vi "BRig_RT_start_v1,19.vi"() -> ()   [LabVIEW 2014]
uses:
  myRIO_BRig_RT__Case_Exp_stateList.ctl
  myRIO_BRig_RT__Case_NonExp_stateList.ctl
  <vilib>/WebDAVClient/Advanced/SessionHandle.ctl
  <vilib>/Platform/TimedLoop/XDataNode/timing_clust.ctl
  <vilib>/Platform/TimedLoop/XDataNode/nitl_modes.ctl
  <vilib>/Platform/TimedLoop/XDataNode/wakeup.ctl
  <vilib>/myRIO/Common/Instrument Driver Framework/myRIO v1.0/UART/vis/myRIO v1.0 Close UART.vi
  <vilib>/FPGAPlugInAG/myRIO-1900/niLvFpga_Open_myRIO-1900.vi
  <vilib>/rvi/interface/common/dynamic/niFpgaDynamicAddResources.vi
  <vilib>/Utility/error.llb/Error Cluster From Error Code.vi
  <vilib>/rvi/errors/niLvFpgaAdjustHostInterfaceError.vi
  <vilib>/Utility/file.llb/Read From Spreadsheet File (I64).vi
  <vilib>/Utility/file.llb/Write To Spreadsheet File (DBL).vi
  <vilib>/FPGAPlugInAG/Dynamic/niLvFpga_Close_Dynamic.vi
  <vilib>/myRIO/Common/Instrument Driver Framework/Utilities/vis/FPGA Ref Manager.vi
  <vilib>/myRIO/Common/Instrument Driver Framework/myRIO v1.0/myRIO v1.0 Reset FPGA.vi
  <vilib>/myRIO/Common/Instrument Driver Framework/myRIO v1.0/IRQ/vis/myRIO v1.0 IRQ Info FGV.vi
  <vilib>/myRIO/Common/Instrument Driver Framework/myRIO v1.0/IRQ/vis/myRIO v1.0 Timer IRQ Info FGV.vi
  <vilib>/myRIO/Common/Instrument Driver Framework/myRIO v1.0/IRQ/vis/myRIO v1.0 ISR Agent.vi
  <vilib>/rvi/interface/nirviOpenFPGA/nirviOpenFPGA.xnode
  BRig_FPGA_v3,95__build.lvbitx
  BRig_FPGA_v3,95.vi
  <vilib>/rvi/interface/nirviReadWriteControl/nirviReadWriteControl.xnode
  <vilib>/Platform/TimedLoop/XDataNode/XDataNode.xnode
  <vilib>/rvi/interface/nirviCloseFPGA/nirviCloseFPGA.xnode
  <vilib>/Platform/TimedLoop/XDataNode/XDNodeRunTimeDep.lvlib
  <vilib>/rvi/interface/Simulation/niFpgaSimulationCallBeginRW.vi
  <vilib>/myRIO/Instrument Drivers/Utilities/Utilities.lvlib
  NiFpgaLv.dll
  <vilib>/WebDAVClient/NI_WebDAV.lvlib
panel:
  out "DAB_flipLR":bool caption="Flip?\n(DAB)"
  in  "LaserFiber_V_l2":dbl
  in  "LaserFiber_V_l1":dbl
  out "Solenoid R":bool
  out "Solenoid L":bool
  out "Laser2":bool
  out "Laser1":bool
  out "FreeReward_c_R":u16
  out "FreeReward_c_L":u16
  in  "Laser2_LED":bool
  in  "Laser1_LED":bool
  in  "lick_Rising(F)_or_Falling(T)":bool
  out "T_ExpRun_min":dbl
  out "stop_TimedLoop":bool
  out "BTPR_avg_R":dbl
  out "T2R_avg_R":dbl
  out "BTPR_avg_L":dbl
  out "T2R_avg_L":dbl
  out "BTPR_block":u16
  out "T2R_block":u16
  in  "comm_WebDAV_connect":bool
  in  "I_sendData":bool
  in  "comm_TCP_connect":bool
  out "nRewards_total":u16 caption="# Rewards in Current Block"
  out "BUR_target":u16 caption="Target Trials Per Block"
  in  "input_Threshold_reset":bool
  out "nTrial":u16
  out "allReward_R":bool
  out "allReward_L":bool
  out "Threshold":bool
  out "tLoop":dbl format="%#_2g"
  out "L_Power_l2":dbl
  out "comm_TCP":bool
  in  "get_countPerMS":bool
  out "SolenoidReward":bool
  out "L_Power_l1":dbl caption="LaserPower"
  in  "Recording":bool
  out "FPGA_count2ms":dbl=159.0
  out "error out":errorcluster
  out "cSpout":enum16{"Left", "Right"}(ring) caption="Left or Right Spout"
  out "A4":u32 caption="LickCounter_Right"
  out "A2":u32 caption="LickCounter_Left"
  out "nRewards_Right":u16 caption="# Rewards Total (Right)"
  out "nRewards_Left":u16 caption="# Rewards Total (Left)"
  out "nRewards_cur":u16 caption="# Rewards in Current Block"
  out "TpB_target":u16 caption="Target Trials Per Block"
  out "cState_NonExp":T1 caption="WarmUp State"
  out "iBlock":u16 caption="Current Block"
  out "cState":T2 caption="Experimental State"
  out "iTrial":u16 caption="Current Trial"
  in  "Data Set Prefix":string="Exp1_TM2"
  out "comm_WebDAV":bool
  in  "Host Password":string="sabalab"
  in  "Host UserName":string="Test2"
  in  "STOP_abort":bool caption="Stop LabView\n(Stops myRio and FPGA)"
  in  "STOP_endBlock":bool caption="Stop Experiment\n@ End of Block"
  in  "STOP_endTrial":bool caption="Stop Experiment\n@ End of Trial"
  in  "START":bool caption="Start Experiment"
  # "Experimental Run"
  # "Recording Rig"
  # "FPGA Conversion\n[counts per ms]"
  # "RealTime Cycle\nShould be <5ms"
  # "STOP experiment at"
  # "Exp Run Time"
  # "Reset"
  # "min"
  # "Communication with Host"
  # "Lick Counter"
  # "Block Target"
  # "Give Water?\n(Reward)"
  # "# Blocks"
  # "Experimental State"
  # "Left/Right"
  # "# Trials"
  # "# Rewards"
  # "Left           Right"
  # "Bad Trials\nPost Reward"
  # "Trials 2 Reward"
  # "Direction\n(NonSpecific Licking)"
  # "Block"
  # "Laser1"
  # "Laser2"
  # "# Trials"
  # "# Rewards"
  # "Current\nBlock"
  # "L          R"
  # "Power [V]"
  # "avg L"
  # "Toggle\nLED"
  # "Total"
  # "# Rewards"
  # "Laser Trigger"
  # "# Trials"
  # "avg R"
  # "1          2"
  # "Fiber Angle\n[V]"
  # "Left           Right"
  # "FreeRewards"
  # "Solenoid Trigger"
  # "WarmUp State"
  # "Lick Detection\nRising (F) or Falling (T)"
  # "L          R"
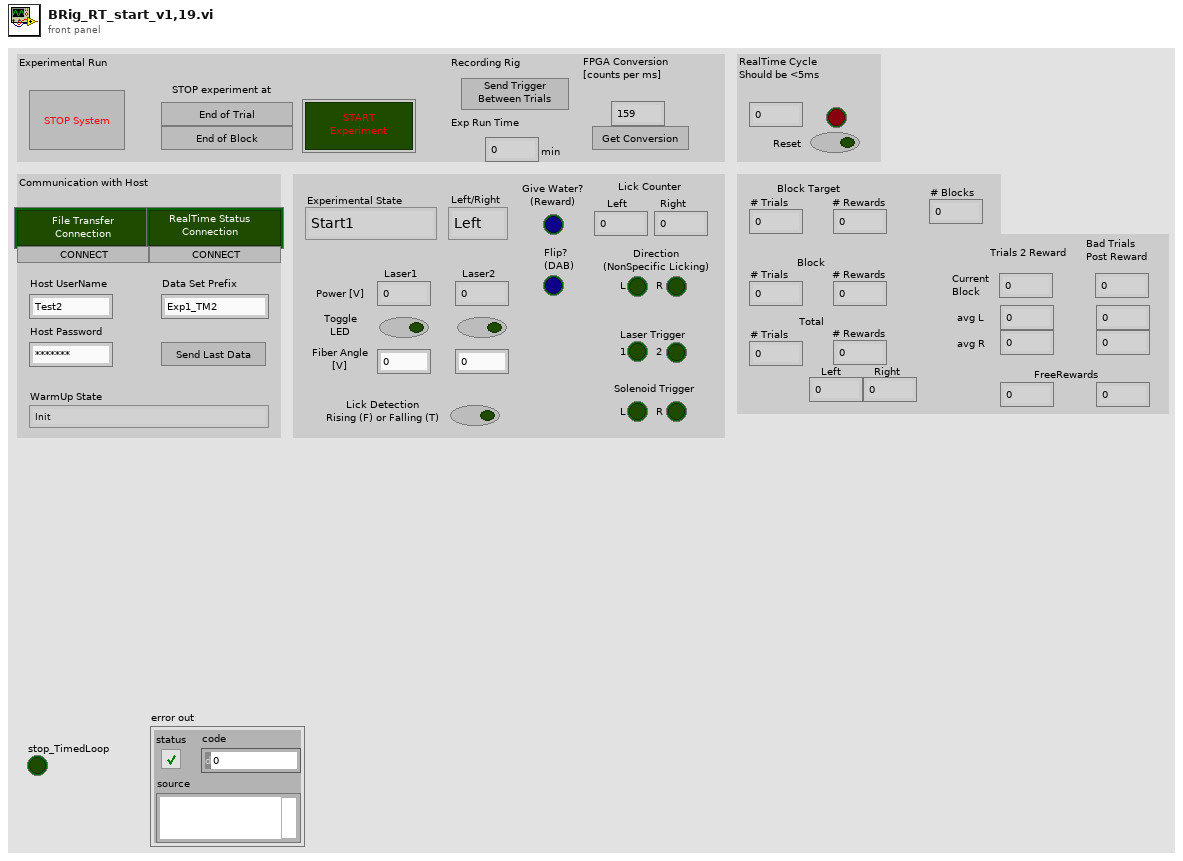
[diagram p1: front panel]
types:
  T1 = typedef "myRIO_BRig_RT__Case_NonExp_stateList.ctl" = enum16{"Init", "UploadSettings_pre", "UploadSettings_Read_dataExp", "UploadSettings_dataExp_1", "UploadSettings_dataExp_2", "UploadSettings_Read_dataLC", "UploadSettings_dataLC_1", "UploadSettings_dataLC_2", "UploadSettings_dataLC_3", "UploadSettings_dataLC_4", "UploadSettings_Read_dataMTrig", "UploadSettings_dataMTrig_1", "UploadSettings_post", "Idle_pre", "IdleEmpty", "IdleEmpty2", "IdleEmpty3", "IdleEmpty4", "Idle", "Idle_2", "Idle_3", "Idle_4", "Idle_5", "Idle_6", "Idle_post", "Cue_pre__pre", "Cue_pre", "Cue", "Cue_LED", "Cue_post", "RewardCalibration_pre", "RewardCalibration", "DispenseWater_pre__pre", "DispenseWater_pre", "DispenseWater", "DispenseWater_post", "TestConnection", "SendData", "Get_FPGA_count_per_ms", "End", "commTCP_connect"}
  T2 = typedef "myRIO_BRig_RT__Case_Exp_stateList.ctl" = enum16{"Start1", "Start2", "Start3", "saveSettings1", "saveSettings2", "saveSettings3", "saveSettings4", "saveSettings_LC_ENL_l1", "saveSettings_LC_ENL_l2", "saveSettings_LC_Cue_l1", "saveSettings_LC_Cue_l2", "saveSettings6_LC_l1_Other", "SaveSettings6_LC_l2_Other", "setSettings_Audio", "setSettings_Laser", "initBlock_pre", "initBlock", "initBlock2", "initBlock_post", "initTrial_pre", "initTrial", "initTrial2", "initTrial3", "initTrial4", "initTrial_LC_ENL1", "initTrial_LC_Cue1", "initTrial_LC_Cue1_2", "initTrial_LC_Sel", "initTrial_post", "ENL1_pre", "ENL1", "ENL1_post", "ENL1Penalty_pre", "ENL1Penalty", "ENL2_pre", "ENL2", "ENL2Penalty_pre", "ENL2Penalty", "Cue1_pre", "Cue1", "Cue1_post", "Cue1Penalty_pre", "Cue1Penalty", "Cue2_pre", "Cue2", "Cue2Penalty_pre", "Cue2Penalty", "Selection_pre", "Selection", "Select_post", "SelectReward_pre", "SelectReward", "SelectRewardPost_pre", "SelectRewardPost", "SelectWrong_pre", "SelectWrong", "SelectWrong_post", "SelectTimeout_pre", "SelectTimeout", "SelectTimeout_post", "endTrial_pre", "endTrial1", "endTrial2", "endTrial3", "endTrial_post", "endBlock_pre", "endBlock", "endBlock_post", "endExp", "commConnect", "commUpload_pre", "commUpload_dataBlock", "commUpload_dataCurrent", "commUpload_dataExp", "commUpload_dataLC", "commUpload_dataTrial", "commUpload_post", "saveData_pre", "saveData_dataBlock", "saveData_dataCurrent", "saveData_dataExp", "saveData_dataLC", "saveData_dataTrial", "saveData_post", "empty_endBlock1", "empty_endBlock2", "empty_endTrial1", "empty_endTrial2", "empty_endTrial3", "empty_endTrial4", "empty_endTrial5", "dummyState", "dummyState_endBlock", "FreeReward_pre", "FreeReward", "FreeRewardPost_pre", "FreeRewardPost"}
  T3 = enum8{"Enabled", "Disabled", "Disabled and Grayed Out"}
  T4 = typedef "NI_WebDAV.lvlib/SessionHandle.ctl" = refnum<k1>
  T5 = typedef "XDNodeRunTimeDep.lvlib/timing_clust.ctl" = cluster{"Expected End [f-1]":u64, "Actual End [f-1]":u64, "Finished Late? [f-1]":bool, "Expected End [i-1]":u64, "Actual End [i-1]":u64, "Finished Late? [i-1]":bool, "Expected Start [i]":u64, "Actual Start [i]":u64, "Expected Start [f]":u64, "Actual Start [f]":u64, "Source Name":string, "Structure Name":string, "Period":i64, "Deadline":i64, "Offset":i64, "Start":i64, "Priority":i32, "Timeout":i32, "Mode":T6, "Wakeup Reason":T7, "Error":errorcluster, "Source Type":string, "Secondary Source Type":string, "Global End Time":u64, "Global Start Time":u64, "Frame Duration":u64, "Iteration Duration":u64, "Assigned CPU":i32, "I/O Scan Engine Mode":u32}
  T6 = typedef "XDNodeRunTimeDep.lvlib/nitl_modes.ctl" = enum32{"No Change", "Process missed periods, maintain original phase", "Discard missed periods, maintain original phase", "Process missed periods, ignore original phase", "Discard missed periods, ignore original phase"}
  T7 = typedef "XDNodeRunTimeDep.lvlib/wakeup.ctl" = enum32{"Normal", "Aborted", "Asynchronous wakeup", "Timing source error", "Timed loop error", "Timeout"}
  T8 = cluster{"read mode":enum16{"polling", "blocking"}, "write mode":enum16{"polling", "blocking"}}
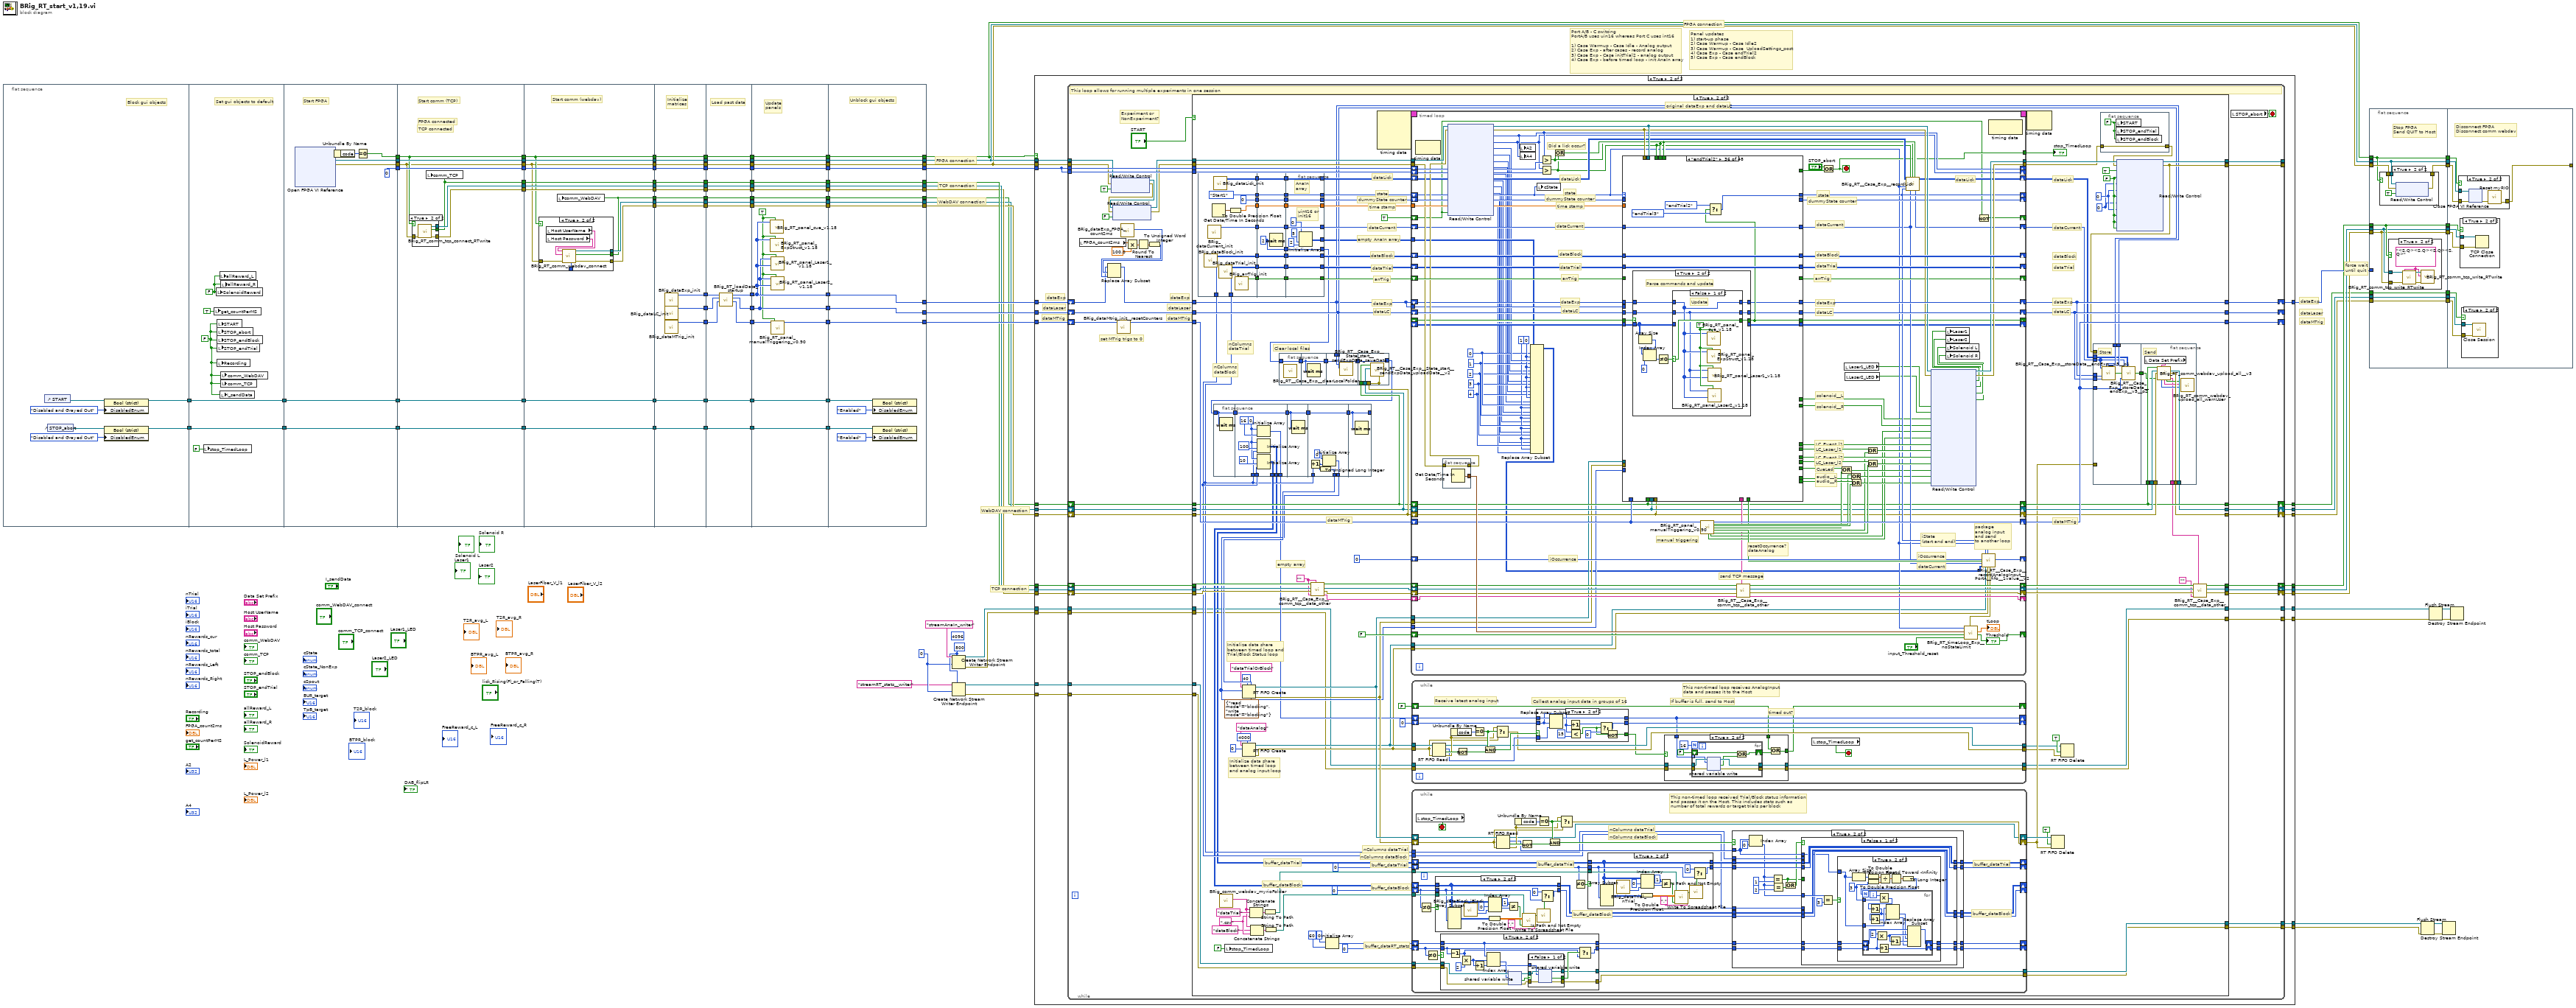
[diagram p0: block diagram]
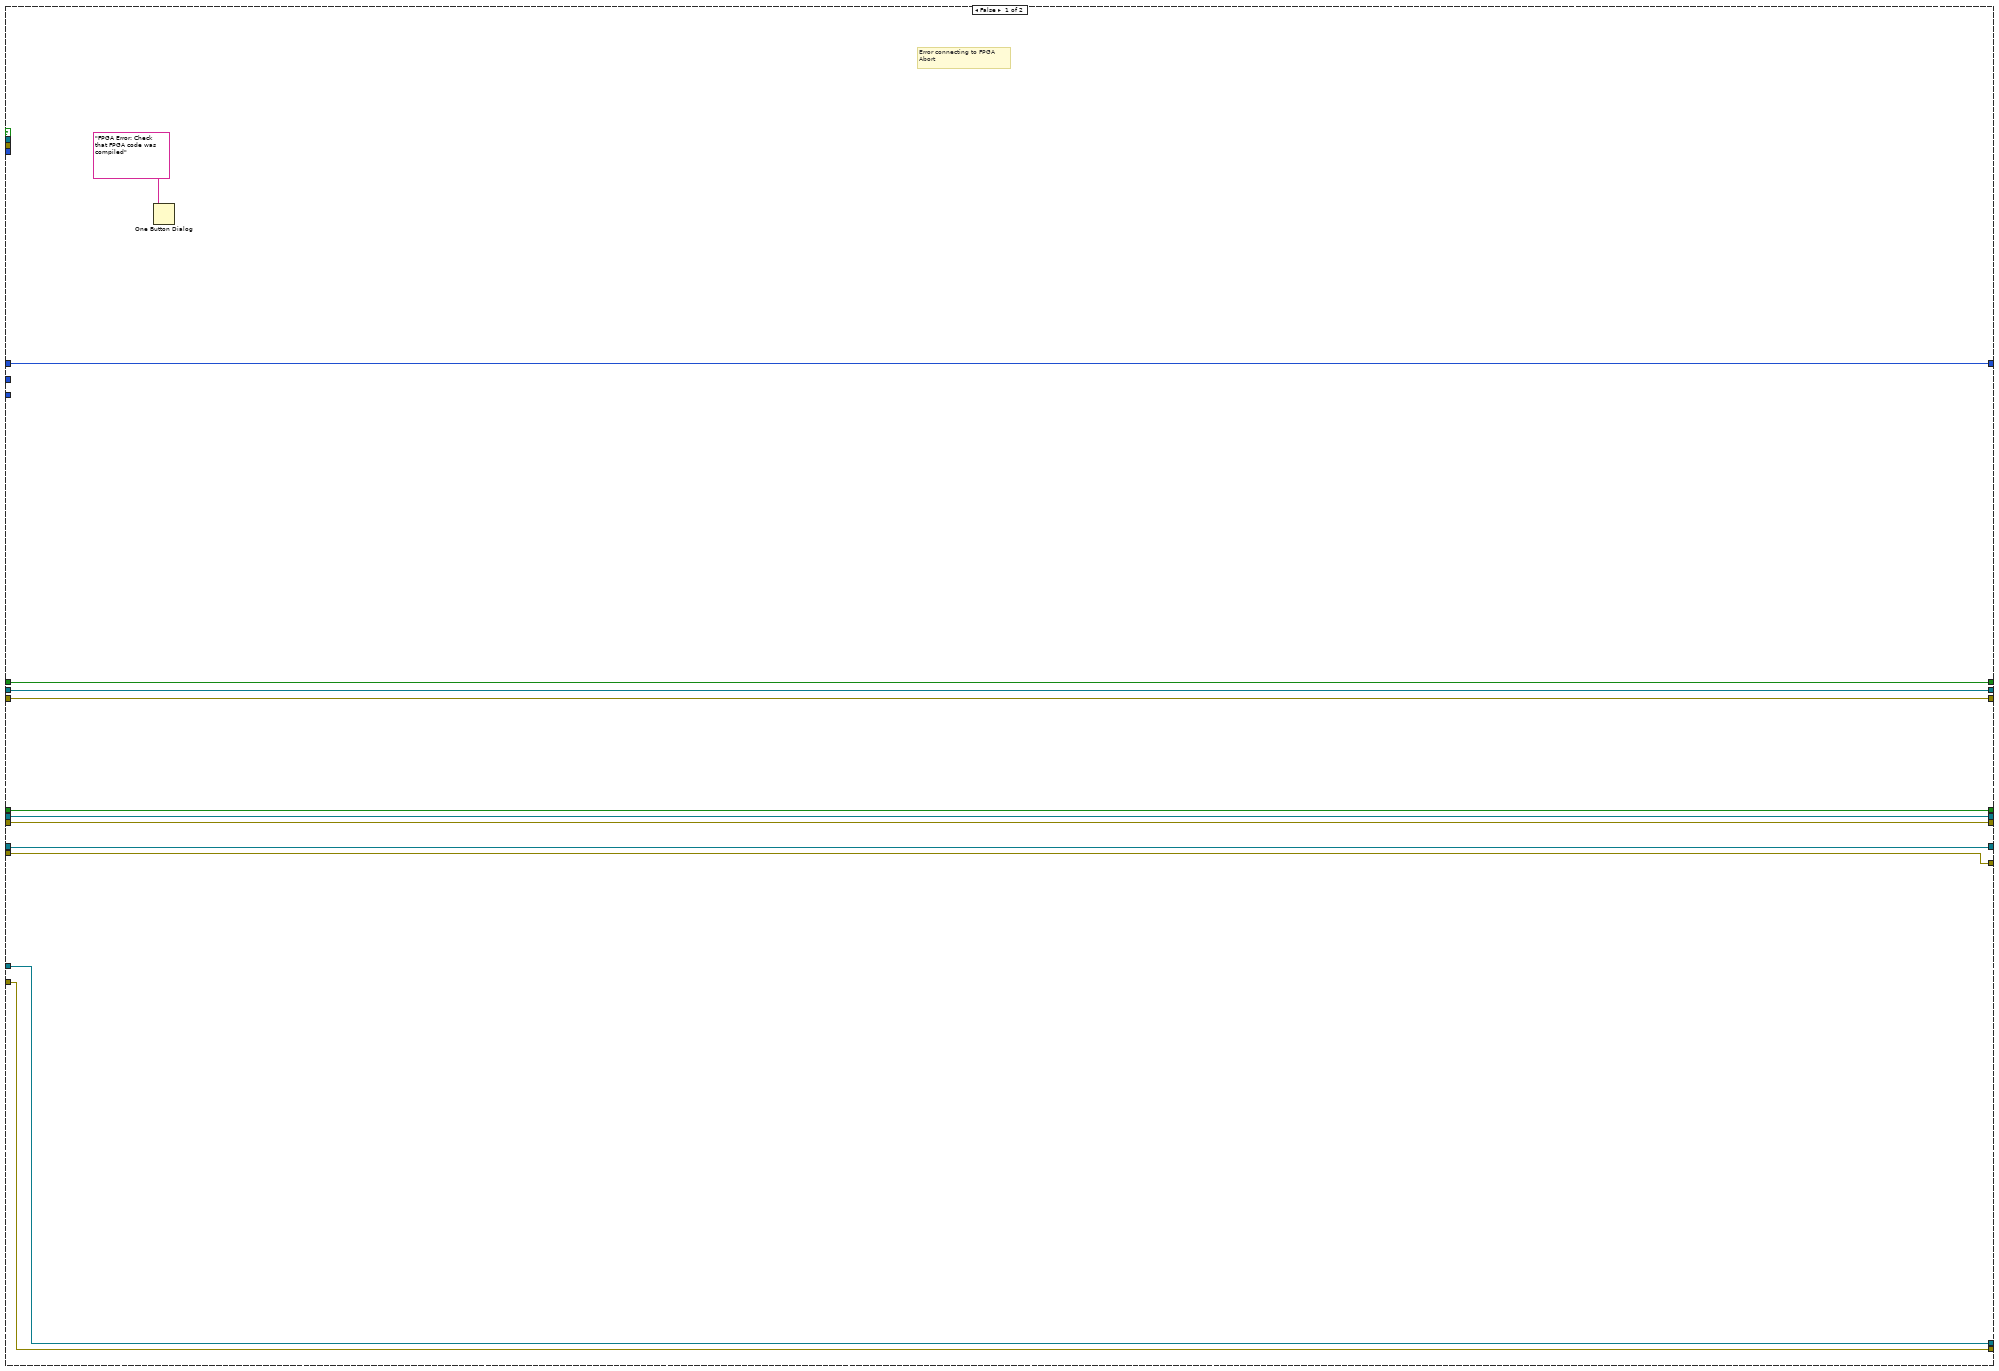
[diagram p2: hidden frame]
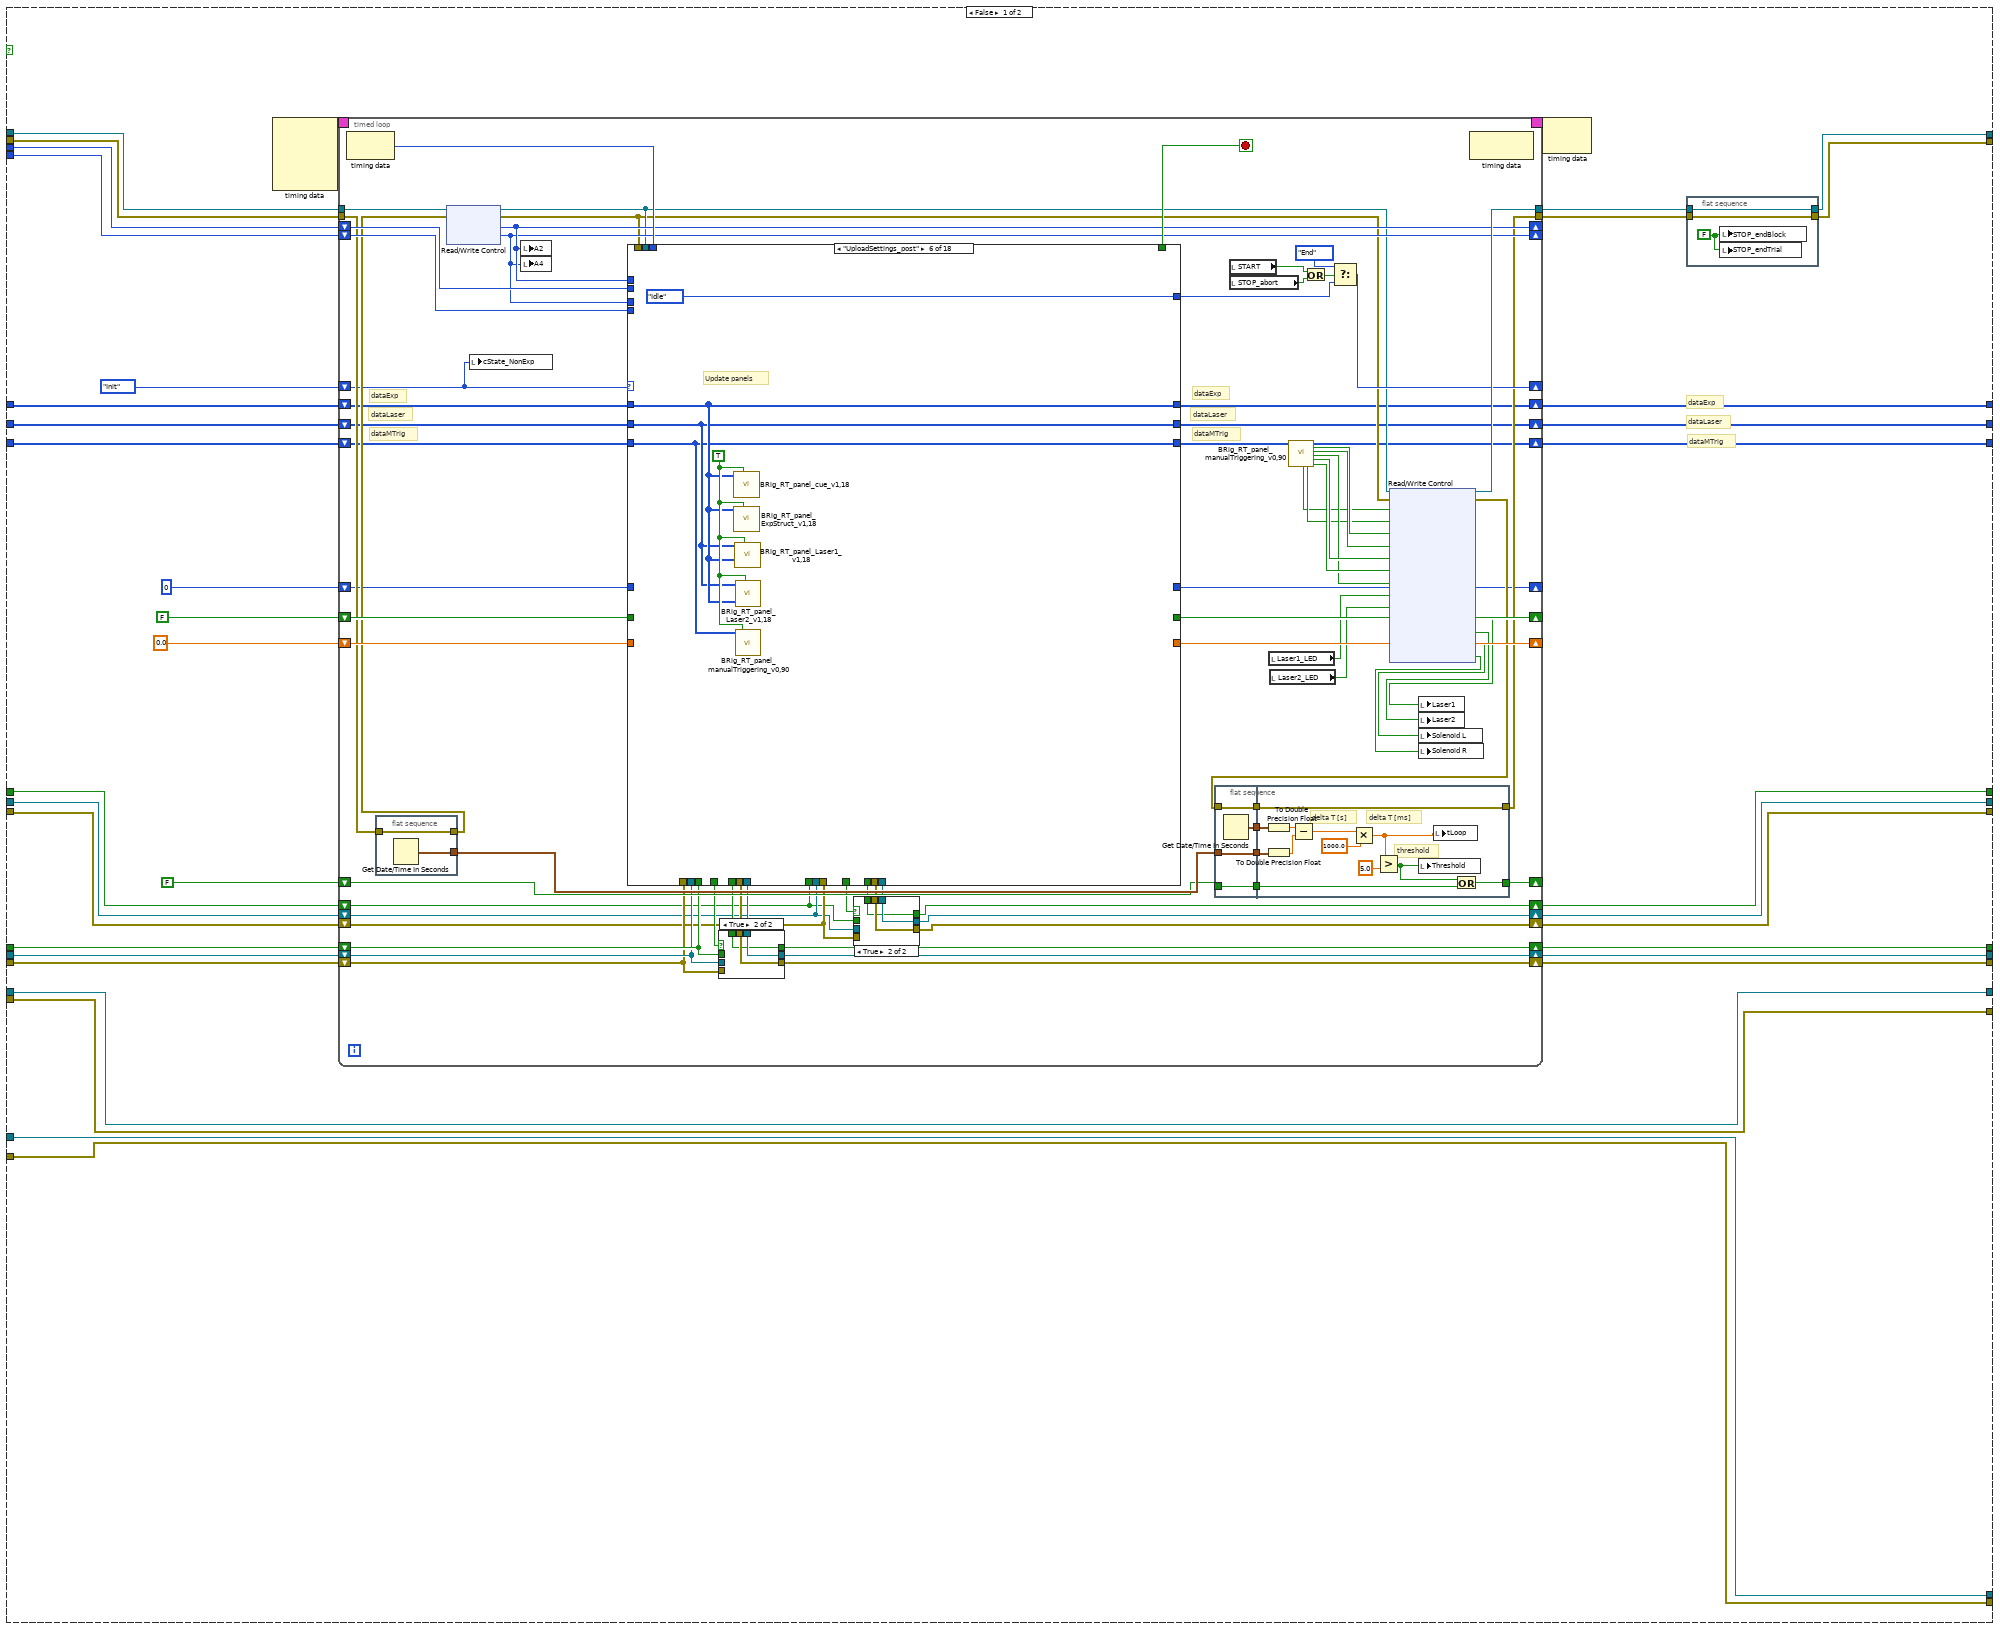
[diagram p3: hidden frame]
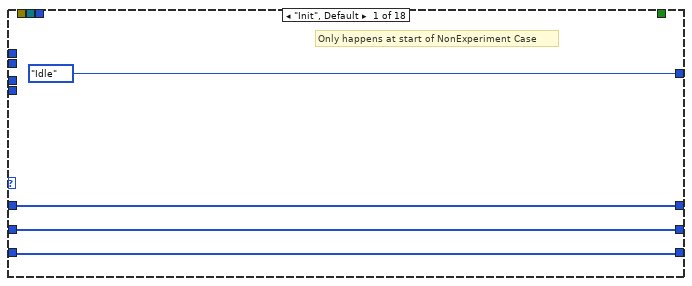
[diagram p6: hidden frame]
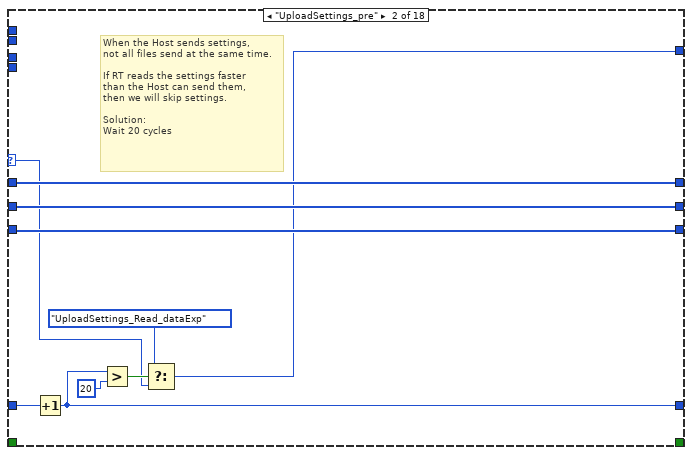
[diagram p7: hidden frame]
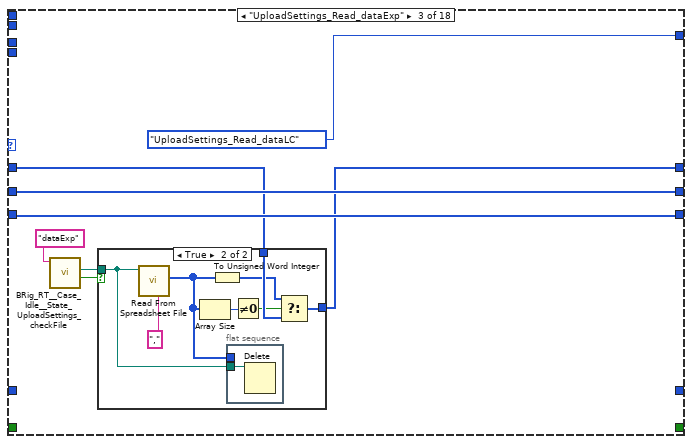
[diagram p8: hidden frame]
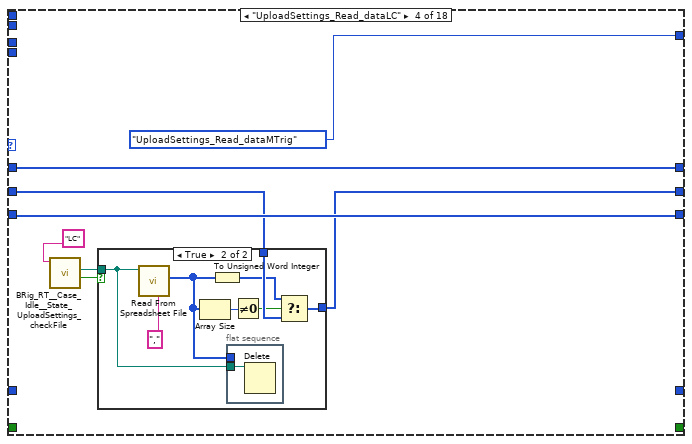
[diagram p10: hidden frame]
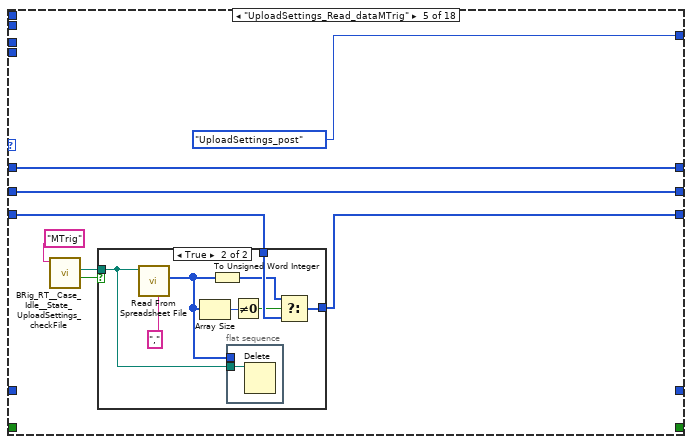
[diagram p12: hidden frame]
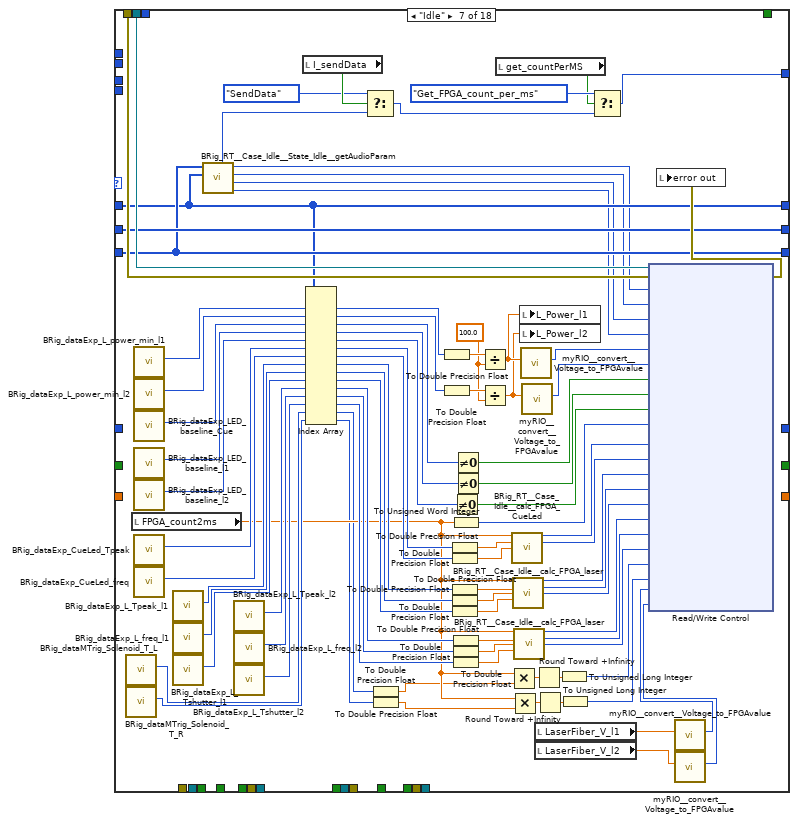
[diagram p14: hidden frame]
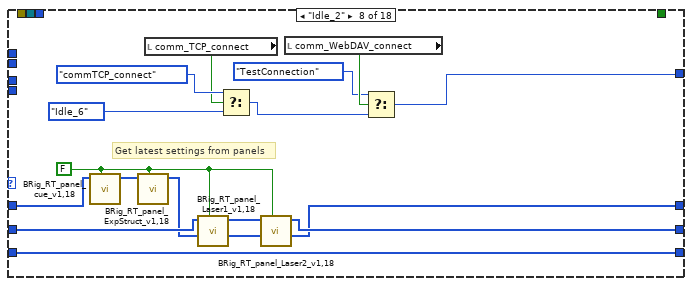
[diagram p15: hidden frame]
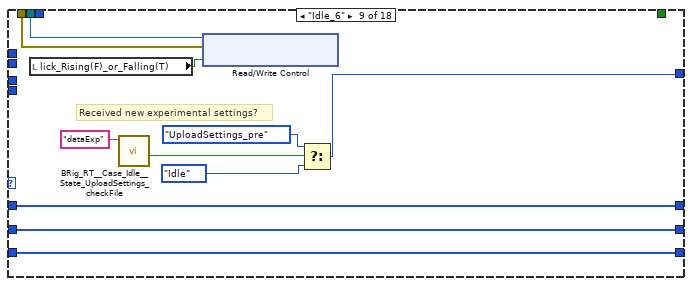
[diagram p16: hidden frame]
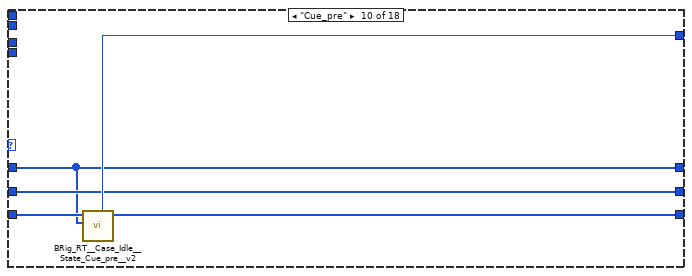
[diagram p17: hidden frame]
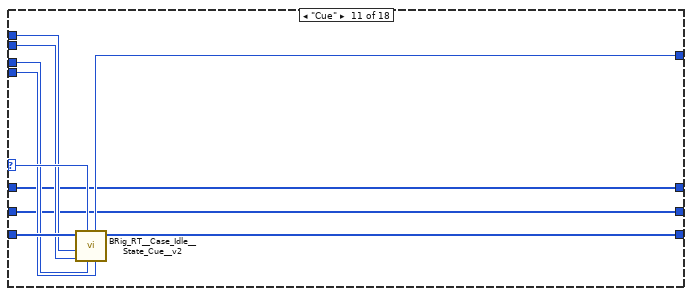
[diagram p18: hidden frame]
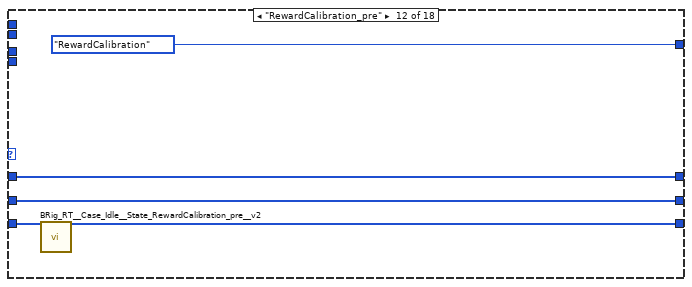
[diagram p19: hidden frame]
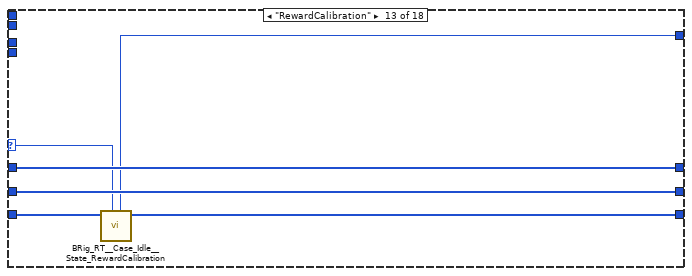
[diagram p20: hidden frame]
diagram:
  w8 = u16 0 ("element")
  (unwired) 4096 ("reader buffer size")
  w9 = 800 ("reader buffer size")
  # "Panel updates\n1) start-up phase\n2) Case Warmup - Case Idle2\n3) Case Warmup - Case  UploadSettings_post\n4) Case Exp - Case endTrial2\n5) Case Exp - Case endBlock"
  # "WebDAV connection"
  # "TCP connection"
  # "WebDAV connection"
  # "TCP connection"
  # "FPGA connection"
  # "FPGA connection"
  # "Port A/B - C switcing\nPortA/B uses uin16 whereas Port C uses int16\n\n1) Case Warmup - Case Idle - Analog output\n2) Case Exp - after cases - record analog\n3) Case Exp - Case initTrial2 - analog output\n4) Case Exp - before timed loop - init AnaIn array"
  # "force wait\nuntil quit"
  # "dataLaser"
  # "dataExp"
  # "dataMTrig"
  n1 = flat-sequence {
    tunnel: [w123] -> w106
    tunnel: [w122] -> w102
    tunnel: [w132] -> w107
    tunnel: w106 -> [w132]
    tunnel: [w131] -> w103
    tunnel: w102 -> [w131]
    tunnel: [w138] -> w120
    tunnel: [w140] -> w119
    tunnel: [u32 0] -> w118
    tunnel: [w136] -> w117
    tunnel: [w135] -> w108
    tunnel: w107 -> [w135]
    tunnel: [w134] -> w104
    tunnel: w103 -> [w134]
    tunnel: w120 -> [w146]
    tunnel: w119 -> [w149]
    tunnel: w118 -> [w148]
    tunnel: w117 -> [w147]
    tunnel: [w146] -> w116
    tunnel: [w149] -> w115
    tunnel: [w148] -> w114
    tunnel: [w147] -> w113
    tunnel: [w141] -> w112
    tunnel: [w145] -> w111
    tunnel: [w144] -> w110
    tunnel: [w143] -> w109
    tunnel: w108 -> [w143]
    tunnel: [w142] -> w105
    tunnel: w104 -> [w142]
    tunnel: w116 -> [w160]
    tunnel: w115 -> [w168]
    tunnel: w114 -> [w167]
    tunnel: w113 -> [w161]
    tunnel: w112 -> [w166]
    tunnel: w111 -> [w165]
    tunnel: w110 -> [w164]
    tunnel: [w160] -> w73
    tunnel: [w168] -> w72
    tunnel: [w167] -> w71
    tunnel: [w161] -> w70
    tunnel: [w166] -> w69
    tunnel: [w165] -> w68
    tunnel: [w164] -> w67
    tunnel: [w163] -> w66
    tunnel: w109 -> [w163]
    tunnel: [w162] -> w65
    tunnel: w105 -> [w162]
    tunnel: [w159] -> w64
    tunnel: [w157] -> w63
    tunnel: [w158] -> w62
    tunnel: w73 -> [w193]
    tunnel: [w193] -> w61
    tunnel: w72 -> [w192]
    tunnel: [w192] -> w60
    tunnel: w71 -> [w191]
    tunnel: [w191] -> w59
    tunnel: w70 -> [w190]
    tunnel: [w190] -> w58
    tunnel: w69 -> [w189]
    tunnel: [w189] -> w57
    tunnel: w68 -> [w188]
    tunnel: [w188] -> w56
    tunnel: w67 -> [w187]
    tunnel: [w187] -> w55
    tunnel: w66 -> [w186]
    tunnel: [w186] -> w54
    tunnel: w65 -> [w185]
    tunnel: [w185] -> w53
    tunnel: w64 -> [w184]
    tunnel: [w184] -> w52
    tunnel: w63 -> [w183]
    tunnel: [w183] -> w51
    tunnel: w62 -> [w182]
    tunnel: [w182] -> w50
    tunnel: [w181] -> w49
    tunnel: [w180] -> w48
    tunnel: [w179] -> w47
    tunnel: w61 -> [w211]
    tunnel: [w211] -> w46
    tunnel: w60 -> [w210]
    tunnel: [w210] -> w44
    tunnel: w59 -> [w209]
    tunnel: [w209] -> w42
    tunnel: w58 -> [w208]
    tunnel: [w208] -> w40
    tunnel: w57 -> [w207]
    tunnel: [w207] -> w38
    tunnel: w56 -> [w206]
    tunnel: [w206] -> w36
    tunnel: w55 -> [w205]
    tunnel: [w205] -> w34
    tunnel: w54 -> [w204]
    tunnel: [w204] -> w32
    tunnel: w53 -> [w203]
    tunnel: [w203] -> w30
    tunnel: w52 -> [w202]
    tunnel: [w202] -> w28
    tunnel: w51 -> [w201]
    tunnel: [w201] -> w26
    tunnel: w50 -> [w200]
    tunnel: [w200] -> w24
    tunnel: w49 -> [w195]
    tunnel: [w194] -> w22
    tunnel: w48 -> [w197]
    tunnel: [w196] -> w20
    tunnel: w47 -> [w199]
    tunnel: [w198] -> w19
    tunnel: w46 -> [w228]
    tunnel: [w228] -> w45
    tunnel: w44 -> [w227]
    tunnel: [w227] -> w43
    tunnel: w42 -> [w226]
    tunnel: [w226] -> w41
    tunnel: w40 -> [w225]
    tunnel: [w225] -> w39
    tunnel: w38 -> [w224]
    tunnel: [w224] -> w37
    tunnel: w36 -> [w223]
    tunnel: [w223] -> w35
    tunnel: w34 -> [w222]
    tunnel: [w222] -> w33
    tunnel: w32 -> [w221]
    tunnel: [w221] -> w31
    tunnel: w30 -> [w220]
    tunnel: [w220] -> w29
    tunnel: w28 -> [w219]
    tunnel: [w219] -> w27
    tunnel: w26 -> [w218]
    tunnel: [w218] -> w25
    tunnel: w24 -> [w217]
    tunnel: [w217] -> w23
    tunnel: w22 -> [w214]
    tunnel: [w213] -> w21
    tunnel: w20 -> [w215]
    tunnel: w19 -> [w216]
    tunnel: [w216] -> w18
    tunnel: [w215] -> w17
    tunnel: [w235] -> w83
    tunnel: [w236] -> w84
    tunnel: [w237] -> w85
    tunnel: [w242] -> w89
    tunnel: [w243] -> w121
    tunnel: [w244] -> w96
    tunnel: [w245] -> w95
    tunnel: w45 -> [w245]
    tunnel: w43 -> [w244]
    tunnel: w41 -> [w243]
    tunnel: w39 -> [w242]
    tunnel: w37 -> [w237]
    tunnel: w35 -> [w236]
    tunnel: w33 -> [w235]
    tunnel: w31 -> [w239]
    tunnel: w29 -> [w238]
    tunnel: w27 -> [w233]
    tunnel: w25 -> [w234]
    tunnel: w23 -> [w232]
    tunnel: [w234] -> w77
    tunnel: [w233] -> w78
    tunnel: [w232] -> w79
    tunnel: [w229] -> w92
    tunnel: [w230] -> w91
    tunnel: [w231] -> w90
    tunnel: w21 -> [w231]
    tunnel: w18 -> [w229]
    tunnel: w17 -> [w230]
    frame #0 {
      # "Block gui objects"
      n2 = control-ref of="START"() -> (w127:refnum<vi>)
      n3 = control-ref of="STOP_abort"() -> (w124:refnum<vi>)
      n4 = property class="Bool (strict)"(reference=w127, "DisabledEnum"=T3."Disabled and Grayed Out" ("Disabled")) -> (reference out=w123:refnum<vi>)  [unwired: 1 in, 1 out]
      n5 = property class="Bool (strict)"(reference=w124, "DisabledEnum"=T3."Disabled and Grayed Out" ("Disabled")) -> (reference out=w122:refnum<vi>)  [unwired: 1 in, 1 out]
    }
    frame #1 {
      w129 = FALSE ("SolenoidReward")
      w130 = FALSE
      # "Set gui objects to default"
      n6 = local write "stop_TimedLoop"(FALSE ("stop_TimedLoop")) -> ()
      n7 = local write "get_countPerMS"(TRUE ("get_countPerMS")) -> ()
      n8 = local write "SolenoidReward"(w129) -> ()
      n9 = local write "START"(w130) -> ()
      n10 = local write "STOP_abort"(w130) -> ()
      n11 = local write "STOP_endBlock"(w130) -> ()
      n12 = local write "STOP_endTrial"(w130) -> ()
      n13 = local write "Recording"(w130) -> ()
      n14 = local write "allReward_L"(w129) -> ()
      n15 = local write "I_sendData"(w130) -> ()
      n16 = local write "comm_WebDAV"(w130) -> ()
      n17 = local write "comm_TCP"(w130) -> ()
      n18 = local write "allReward_R"(w129) -> ()
    }
    frame #2 {
      # "Start FPGA"
      n19 = xnode "Open FPGA VI Reference"() -> ("FPGA VI Reference Out"=w140:refnum<k20>, "error out"=w138:errorcluster)  [unwired: 2 in]
      n20 = Unbundle By Name(w138) -> ("code"=w137:i32)
      n21 = Equal To 0?(x=w137) -> (x = 0?=w136:bool)
    }
    frame #3 {
      # "TCP connected"
      # "Start comm (TCP)"
      # "FPGA connected"
      n22 = case shown="True" w147 {
        selector: w147 -> [w150 _]
        tunnel: w146 -> [w152 w156]
        tunnel: [refnum<k5> refnum ("output_hTCP") w155] -> w145
        tunnel: [w150 w154] -> w141
        tunnel: [w152 w153] -> w144
        frame False {
        }
        frame True {
          n23 = call "BRig_RT_comm_tcp_connect_RTwrite.vi"("input_error"=w156) -> ("output_error"=w153:errorcluster, "output_connected"=w154:bool, "output_hTCP"=w155:refnum<k5>)  [unwired: 8 in]
        }
      }
      n24 = local write "comm_TCP"(w141) -> ()
    }
    frame #4 {
      # "Start comm (webdav)"
      n25 = case shown="True" w161 {
        selector: w161 -> [w170 _]
        tunnel: [w169 w176] -> w159
        tunnel: [w170 w175] -> w157
        tunnel: w160 -> [w171 w174]
        tunnel: [w171 w173] -> w158
        tunnel: [_ w172] -> _
        frame False {
          w169 = T4 refnum items=["Session NI_WebDAV"] ("output_hSession")
        }
        frame True {
          n26 = local read "Host UserName"() -> (w177:string)
          n27 = local read "Host Password"() -> (w178:string)
          n28 = call "BRig_RT_comm_webdav_connect.vi"("input_error"=w174, "input_password"=w178, "input_username"=w177) -> ("output_error"=w173:errorcluster, "output_Iconnected"=w175:bool, "output_hSession"=w176:T4, "output_code"=w172:u8)  [unwired: 5 in]
        }
      }
      n29 = local write "comm_WebDAV"(w157) -> ()
    }
    frame #5 {
      # "Initialize\nmatrices"
      n30 = call "BRig_dataExp_init.vi"() -> ("output_dataExp"=w179:u16[])  [unwired: 11 in]
      n31 = call "BRig_dataLC_init.vi"() -> ("output_dataLC"=w180:u16[])  [unwired: 11 in]
      n32 = call "BRig_dataMTrig_init.vi"() -> ("output_dataMTrig"=w181:u16[])  [unwired: 5 in]
    }
    frame #6 {
      # "Load past data"
      n33 = call "BRig_RT_loadData_startup.vi"("input_dataMTrig"=w195, "input_dataLC"=w197, "input_dataExp"=w199) -> ("output_dataMTrig"=w194:u16[], "output_dataLC"=w196:u16[], "output_dataExp"=w198:u16[])  [unwired: 6 in]
    }
    frame #7 {
      w212 = TRUE ("input_setValues")
      # "Update\npanels"
      n34 = call "BRig_RT_panel_cue_v1,18.vi"("input_setValues"=w212, "input_dataExp"=w216) -> ()  [unwired: 9 in, 1 out]
      n35 = call "BRig_RT_panel_ExpStruct_v1,18.vi"("input_setValues"=w212, "input_dataExp"=w216) -> ()  [unwired: 9 in, 1 out]
      n36 = call "BRig_RT_panel_Laser1_v1,18.vi"("input_setValues"=w212, "input_dataExp"=w216, "input_dataLC"=w215) -> ()  [unwired: 7 in, 2 out]
      n37 = call "BRig_RT_panel_Laser2_v1,18.vi"("input_setValues"=w212, "input_dataExp"=w216, "input_dataLC"=w215) -> ()  [unwired: 7 in, 2 out]
      n38 = call "BRig_RT_panel_manualTriggering_v0,90.vi"("input_dataMTrig"=w214, "input_setValues"=w212) -> ("output_dataMTrig"=w213:u16[])  [unwired: 10 in, 7 out]
    }
    frame #8 {
      # "Unblock gui objects"
      n39 = property class="Bool (strict)"(reference=w239, "DisabledEnum"=T3."Enabled" ("Disabled")) -> ()  [unwired: 1 in, 2 out]
      n40 = property class="Bool (strict)"(reference=w238, "DisabledEnum"=T3."Enabled" ("Disabled")) -> ()  [unwired: 1 in, 2 out]
    }
  }
  n41 = Create Network Stream Writer Endpoint(7:w9, 9:w8, 11:"streamAnaIn_writer" ("reader name")) -> (0:w10:errorcluster, 3:w11:refnum<k21>)  [unwired: 4 in]
  n42 = Create Network Stream Writer Endpoint(7:w9, 9:w8, 11:"streamRT_stats__writer" ("writer name")) -> (0:w5:errorcluster, 3:w6:refnum<k21>)  [unwired: 4 in]
  n43 = case shown="True" w89 {
    tunnel: w121 -> [_ w284]
    tunnel: w96 -> [_ w283]
    tunnel: w95 -> [_ w282]
    tunnel: [w257 w281] -> w93
    tunnel: w92 -> [w257 w280]
    tunnel: w91 -> [_ w279]
    tunnel: w90 -> [_ w278]
    tunnel: w85 -> [w256 w277]
    tunnel: w84 -> [w255 w276]
    tunnel: w83 -> [w254 w275]
    tunnel: [w256 w274] -> w82
    tunnel: [w255 w273] -> w81
    tunnel: [w254 w272] -> w80
    tunnel: w79 -> [w253 w271]
    tunnel: w78 -> [w252 w270]
    tunnel: w77 -> [w251 w269]
    tunnel: [w253 w268] -> w76
    tunnel: [w252 w267] -> w75
    tunnel: [w251 w266] -> w74
    tunnel: [w250 w265] -> w14
    tunnel: [w249 w264] -> w13
    tunnel: w11 -> [w250 w263]
    tunnel: w10 -> [w249 w262]
    tunnel: w6 -> [w247 w261]
    tunnel: w5 -> [w246 w260]
    tunnel: [w247 w259] -> w2
    tunnel: [w246 w258] -> w1
    frame False {
      # "Error connecting to FPGA\nAbort"
      n44 = One Button Dialog(message="FPGA Error: Check that FPGA code was compiled") -> ()  [unwired: 1 in, 1 out]
    }
    frame True {
      # "dataExp"
      # "dataLaser"
      # "dataMTrig"
      n45 = while {
        tunnel: w283 -> [w322]
        tunnel: w282 -> [w327]
        tunnel: w284 -> [w330]
        tunnel: w284 -> [w329]
        tunnel: [w320] -> _
        tunnel: [w319] -> _
        shift-right: [w318] -> _
        shift-left: w278 -> [w315]
        shift-right: [w316] -> _
        shift-left: w279 -> [w317]
        shift-right: [w286] -> w281
        shift-left: w280 -> [w295]
        shift-right: [w310] -> w274
        shift-left: w277 -> [w313]
        shift-right: [w309] -> w273
        shift-left: w276 -> [w312]
        shift-right: [w308] -> w272
        shift-left: w275 -> [w311]
        shift-right: [w304] -> w268
        shift-left: w271 -> [w307]
        shift-right: [w303] -> w267
        shift-left: w270 -> [w306]
        shift-right: [w302] -> w266
        shift-left: w269 -> [w305]
        tunnel: [w294] -> w265
        tunnel: [w293] -> w264
        tunnel: w263 -> [w292]
        tunnel: w262 -> [w291]
        tunnel: w261 -> [w290]
        tunnel: w260 -> [w289]
        tunnel: [w288] -> w259
        tunnel: [w287] -> w258
        stop <- w328 stop-if-true
        # "set MTrig trigs to 0"
        # "dataExp"
        # "dataLaser"
        # "dataMTrig"
        # "Experiment or\nNonExperiment?"
        # "This loop allows for running multiple experiments in one session"
        n46 = local read "FPGA_count2ms"() -> (w299:dbl)
        n47 = xnode "Read/Write Control"("FPGA VI Reference In"=w322, "error in"=w327, "Counts_Reset"=TRUE) -> ("FPGA VI Reference Out"=w324:refnum<k20>, "error out"=w325:errorcluster)
        n48 = xnode "Read/Write Control"("FPGA VI Reference In"=w324, "error in"=w325, "Counts_Reset"=FALSE) -> ("FPGA VI Reference Out"=w321:refnum<k20>, "error out"=w323:errorcluster)
        n49 = call "BRig_dataMtrig_init__resetCounters.vi"("input_dataMTrig"=w315) -> ("output_dataMTrig"=w314:u16[])  [unwired: 10 in]
        n50 = call "BRig_dataExp_FPGA_count2ms.vi"() -> ("output_FPGA_count2ms"=w300:i32)  [unwired: 11 in]
        n51 = Multiply(x=w299, y=100.0) -> (x*y=w297:dbl)
        n52 = Round To Nearest(number=w297) -> (nearest integer value=w296:dbl)
        n53 = To Unsigned Word Integer(number=w296) -> (unsigned 16bit integer=w301:u16)
        n54 = Replace Array Subset(array=w295, new element=w301, index=w300) -> (w285:u16[])
        n55 = case shown="True" "START" {
          tunnel: w330 -> [w366 w956]
          tunnel: w329 -> [w365 w955]
          tunnel: w323 -> [w363 w944]
          tunnel: w321 -> [w364 w945]
          tunnel: [w361 w953] -> w320
          tunnel: [w359 w922] -> w319
          tunnel: w314 -> [w355 w942]
          tunnel: [w354 w928] -> w318
          tunnel: w317 -> [w353 w892]
          tunnel: w285 -> [w333 w845]
          tunnel: [w352 w927] -> w316
          tunnel: [w351 w926] -> w286
          tunnel: w313 -> [w350 w936]
          tunnel: w312 -> [w349 w935]
          tunnel: w311 -> [w348 w934]
          tunnel: [w347 w911] -> w310
          tunnel: [w346 w910] -> w309
          tunnel: [w345 w909] -> w308
          tunnel: w307 -> [w344 w891]
          tunnel: w306 -> [w343 w890]
          tunnel: w305 -> [w342 w889]
          tunnel: [w341 w918] -> w304
          tunnel: [w340 w917] -> w303
          tunnel: [w339 w919] -> w302
          tunnel: w292 -> [w337 w850]
          tunnel: w291 -> [w336 w849]
          tunnel: [w337 w848] -> w294
          tunnel: [w336 w847] -> w293
          tunnel: w290 -> [w335 w841]
          tunnel: w289 -> [w334 w842]
          tunnel: [w335 w836] -> w288
          tunnel: [w334 w835] -> w287
          frame False {
            # "dataExp"
            # "dataLaser"
            # "dataMTrig"
            n56 = node-c288() -> (w369:T5)  [unwired: 4 in]
            n57 = timed-loop {
              timing: w369 -> [_]
              timing-out: [_] -> w368
              shift-right: [w437] -> _
              shift-left: myRIO_BRig_RT__Case_NonExp_stateList."Init" ("Enum") -> [w406]
              shift-right: [w435] -> _
              shift-left: w366 -> [w436]
              shift-right: [w433] -> _
              shift-left: w365 -> [w434]
              tunnel: [w443] -> w362
              tunnel: [w419] -> w360
              tunnel: w363 -> [w426]
              tunnel: w364 -> [w444]
              shift-right: [w429] -> _
              shift-left: FALSE -> [w430]
              shift-right: [w427] -> _
              shift-left: 0.0 -> [w428]
              shift-right: [w416] -> _
              shift-left: FALSE -> [w417]
              shift-right: [w415] -> w354
              shift-left: w355 -> [w407]
              shift-right: [w401] -> w351
              shift-left: w333 -> [w404]
              shift-right: [w402] -> w352
              shift-left: w353 -> [w403]
              shift-right: [w400] -> w347
              shift-left: w350 -> [w396]
              shift-right: [w399] -> w346
              shift-left: w349 -> [w395]
              shift-right: [w398] -> w345
              shift-left: w348 -> [w394]
              shift-right: [w384] -> w341
              shift-left: w344 -> [w390]
              shift-right: [w385] -> w340
              shift-left: w343 -> [w389]
              shift-right: [w386] -> w339
              shift-left: w342 -> [w388]
              shift-right: [w379] -> _
              shift-left: u16 0 ("y") -> [w380]
              stop <- w446 stop-if-true
              # "dataExp"
              # "dataLaser"
              # "dataExp"
              # "dataLaser"
              # "dataMTrig"
              # "dataMTrig"
              n58 = node-c288() -> (w445:i64)  [unwired: 1 in]
              n59 = flat-sequence {
                tunnel: w426 -> [w475]
                tunnel: [w476] -> w418
                tunnel: [w475] -> w425
                frame #0 {
                  n60 = Get Date/Time In Seconds() -> (seconds since 1Jan1904=w476:timestamp)
                }
              }
              n61 = xnode "Read/Write Control"("FPGA VI Reference In"=w444, "error in"=w425) -> ("FPGA VI Reference Out"=w432:refnum<k20>, "error out"=w431:errorcluster, "A2_LickL"=w435:u32, "A4_LickR"=w433:u32)
              n62 = local write "cState_NonExp"(w406) -> ()
              n63 = local write "A2"(w435) -> ()
              n64 = local write "A4"(w433) -> ()
              n65 = case shown="\"UploadSettings_post\"" w406 {
                selector: w406 -> [_ w483 _ _ _ _ _ _ _ _ w678 _ w686 _ _ w730 w773 w779]
                tunnel: [myRIO_BRig_RT__Case_NonExp_stateList."Idle" ("Enum") w484 myRIO_BRig_RT__Case_NonExp_stateList."UploadSettings_Read_dataLC" ("t") myRIO_BRig_RT__Case_NonExp_stateList."UploadSettings_Read_dataMTrig" ("t") myRIO_BRig_RT__Case_NonExp_stateList."UploadSettings_post" ("t") myRIO_BRig_RT__Case_NonExp_stateList."Idle" ("t") w571 w641 w661 w667 w676 myRIO_BRig_RT__Case_NonExp_stateList."RewardCalibration" ("Enum") w685 myRIO_BRig_RT__Case_NonExp_stateList."Idle" ("Enum") myRIO_BRig_RT__Case_NonExp_stateList."Idle" ("Enum") w729 w773 w780] -> w438
                tunnel: [w479 w490 w498 w516 w530 w545 w583 w653 w659 w668 w677 w680 w687 w701 w713 w739 w771 w788] -> w405
                tunnel: [_ _ _ _ _ _ _ _ _ _ _ _ _ _ _ _ TRUE _] -> w446
                tunnel: w407 -> [w479 w490 w498 w516 w527 w545 w583 w653 w659 w669 w679 w681 w688 w701 w713 w739 w771 w788]
                tunnel: w445 -> [_ _ _ _ _ _ _ _ _ _ _ _ _ _ _ _ _ _]
                tunnel: w436 -> [_ _ _ _ _ _ _ _ _ _ w674 _ _ _ _ _ _ _]
                tunnel: w435 -> [_ _ _ _ _ _ _ _ _ _ w675 _ _ _ _ _ _ _]
                tunnel: w434 -> [_ _ _ _ _ _ _ _ _ _ w672 _ _ _ _ _ _ _]
                tunnel: w433 -> [_ _ _ _ _ _ _ _ _ _ w673 _ _ _ _ _ _ _]
                tunnel: w432 -> [_ _ _ _ _ _ w636 _ w656 _ _ _ _ _ _ w734 _ _]
                tunnel: w431 -> [_ _ _ _ _ _ w635 _ w655 _ _ _ _ _ _ w733 _ _]
                tunnel: w430 -> [_ _ _ _ _ _ _ _ _ _ _ _ _ _ _ w738 _ _]
                tunnel: [_ _ _ _ _ _ _ _ _ _ _ _ _ _ _ TRUE _ _] -> w429
                tunnel: w428 -> [_ _ _ _ _ _ _ _ _ _ _ _ _ _ _ w736 _ _]
                tunnel: [_ _ _ _ _ _ _ _ _ _ _ _ _ _ _ w735 _ _] -> w427
                tunnel: w404 -> [w477 w488 w493 w515 w534 w547 w582 w640 w657 w665 w670 w683 w689 w698 w710 w726 w769 w786]
                tunnel: w403 -> [w478 w489 w497 w509 w531 w546 w584 w652 w658 w666 w671 w682 w690 w699 w711 w727 w770 w787]
                tunnel: [w478 w489 w497 w512 w531 w546 w584 w648 w658 w666 w671 w682 w690 w699 w711 w727 w770 w787] -> w402
                tunnel: [w477 w488 w492 w515 w534 w547 w582 w637 w657 w665 w670 w683 w689 w698 w710 w726 w769 w786] -> w401
                tunnel: [_ _ _ _ _ _ _ _ _ _ _ _ _ _ _ _ _ TRUE] -> w397
                tunnel: w396 -> [_ _ _ _ _ _ _ _ _ _ _ _ _ _ w704 _ _ w785]
                tunnel: w395 -> [_ _ _ _ _ _ _ _ _ _ _ _ _ _ w706 _ _ w781]
                tunnel: w394 -> [_ _ _ _ _ _ _ _ _ _ _ _ _ _ w705 _ _ w784]
                tunnel: [_ _ _ _ _ _ _ _ _ _ _ _ _ _ _ _ _ w783] -> w393
                tunnel: [_ _ _ _ _ _ _ _ _ _ _ _ _ _ _ _ _ w782] -> w392
                tunnel: [_ _ _ _ _ _ _ _ _ _ _ _ _ _ _ _ _ w774] -> w391
                tunnel: w388 -> [_ _ _ _ _ _ _ _ _ _ _ _ _ _ w703 _ _ _]
                tunnel: w389 -> [_ _ _ _ _ _ _ _ _ _ _ _ _ _ w709 _ _ _]
                tunnel: w390 -> [_ _ _ _ _ _ _ _ _ _ _ _ _ w691 w708 _ _ _]
                tunnel: [_ _ _ _ _ _ _ _ _ _ _ _ _ TRUE _ _ _ _] -> w387
                tunnel: [_ _ _ _ _ _ _ _ _ _ _ _ _ w693 _ _ _ _] -> w383
                tunnel: [_ _ _ _ _ _ _ _ _ _ _ _ _ w691 _ _ _ _] -> w382
                tunnel: [_ _ _ _ _ _ _ _ _ _ _ _ _ w692 _ _ _ _] -> w381
                tunnel: w380 -> [_ w482 _ _ _ _ _ _ _ _ _ _ _ _ _ _ _ _]
                tunnel: [_ w481 _ _ _ _ _ _ _ _ _ _ _ _ _ _ _ _] -> w379
                frame "Init", Default {
                  # "Only happens at start of NonExperiment Case"
                }
                frame "UploadSettings_pre" {
                  # "When the Host sends settings,\nnot all files send at the same time.\n\nIf RT reads the settings faster\nthan the Host can send them,\nthen we will skip settings.\n\nSolution:\nWait 20 cycles"
                  n66 = Increment(x=w482) -> (x+1=w481:u16)
                  n67 = Greater?(x=w481, y=u16 20) -> (0:w486:bool)
                  n68 = Select(t=myRIO_BRig_RT__Case_NonExp_stateList."UploadSettings_Read_dataExp", s=w486, f=w483) -> (s? t:f=w484:T1)
                }
                frame "UploadSettings_Read_dataExp" {
                  n69 = call "BRig_RT__Case_Idle__State_UploadSettings_checkFile.vi"("input_dataName"="dataExp") -> ("output_Iexist"=w495:bool, "output_dataPath"=w494:path)  [unwired: 9 in]
                  n70 = case shown="True" w495 {
                    tunnel: w494 -> [_ w501]
                    tunnel: w493 -> [w499 w505]
                    tunnel: [w499 w503] -> w492
                    frame False {
                    }
                    frame True {
                      n71 = call-poly <vilib>:"Read From Spreadsheet File.vi"("delimiter (\\t)"="," ("delimiter (\\t)"), "file path (dialog if empty)"=w501) -> ("first row"=w500:i64[])  [unwired: 5 in, 4 out]
                      n72 = Array Size(array=w500) -> (size(s)=w506:i32)
                      n73 = To Unsigned Word Integer(number=w500) -> (unsigned 16bit integer=w504:u16[])
                      n74 = flat-sequence {
                        tunnel: w501 -> [w508]
                        tunnel: w500 -> [_]
                        frame #0 {
                          n75 = Delete(path (use dialog)=w508) -> ()  [unwired: 4 in, 3 out]
                        }
                      }
                      n76 = Not Equal To 0?(x=w506) -> (x != 0?=w502:bool)
                      n77 = Select(t=w504, s=w502, f=w505) -> (s? t:f=w503:u16[])
                    }
                  }
                }
                frame "UploadSettings_Read_dataLC" {
                  n78 = call "BRig_RT__Case_Idle__State_UploadSettings_checkFile.vi"("input_dataName"="LC") -> ("output_Iexist"=w510:bool, "output_dataPath"=w511:path)  [unwired: 9 in]
                  n79 = case shown="True" w510 {
                    tunnel: w511 -> [_ w519]
                    tunnel: w509 -> [w517 w523]
                    tunnel: [w517 w521] -> w512
                    frame False {
                    }
                    frame True {
                      n80 = call-poly <vilib>:"Read From Spreadsheet File.vi"("delimiter (\\t)"="," ("delimiter (\\t)"), "file path (dialog if empty)"=w519) -> ("first row"=w518:i64[])  [unwired: 5 in, 4 out]
                      n81 = Array Size(array=w518) -> (size(s)=w524:i32)
                      n82 = To Unsigned Word Integer(number=w518) -> (unsigned 16bit integer=w522:u16[])
                      n83 = flat-sequence {
                        tunnel: w519 -> [w526]
                        tunnel: w518 -> [_]
                        frame #0 {
                          n84 = Delete(path (use dialog)=w526) -> ()  [unwired: 4 in, 3 out]
                        }
                      }
                      n85 = Not Equal To 0?(x=w524) -> (x != 0?=w520:bool)
                      n86 = Select(t=w522, s=w520, f=w523) -> (s? t:f=w521:u16[])
                    }
                  }
                }
                frame "UploadSettings_Read_dataMTrig" {
                  n87 = call "BRig_RT__Case_Idle__State_UploadSettings_checkFile.vi"("input_dataName"="MTrig") -> ("output_Iexist"=w528:bool, "output_dataPath"=w529:path)  [unwired: 9 in]
                  n88 = case shown="True" w528 {
                    tunnel: w529 -> [_ w537]
                    tunnel: w527 -> [w535 w541]
                    tunnel: [w535 w539] -> w530
                    frame False {
                    }
                    frame True {
                      n89 = call-poly <vilib>:"Read From Spreadsheet File.vi"("delimiter (\\t)"="," ("delimiter (\\t)"), "file path (dialog if empty)"=w537) -> ("first row"=w536:i64[])  [unwired: 5 in, 4 out]
                      n90 = Array Size(array=w536) -> (size(s)=w542:i32)
                      n91 = To Unsigned Word Integer(number=w536) -> (unsigned 16bit integer=w540:u16[])
                      n92 = flat-sequence {
                        tunnel: w537 -> [w544]
                        tunnel: w536 -> [_]
                        frame #0 {
                          n93 = Delete(path (use dialog)=w544) -> ()  [unwired: 4 in, 3 out]
                        }
                      }
                      n94 = Not Equal To 0?(x=w542) -> (x != 0?=w538:bool)
                      n95 = Select(t=w540, s=w538, f=w541) -> (s? t:f=w539:u16[])
                    }
                  }
                }
                frame "UploadSettings_post" {
                  w548 = TRUE ("input_setValues")
                  # "Update panels"
                  n96 = call "BRig_RT_panel_cue_v1,18.vi"("input_setValues"=w548, "input_dataExp"=w547) -> ()  [unwired: 9 in, 1 out]
                  n97 = call "BRig_RT_panel_ExpStruct_v1,18.vi"("input_setValues"=w548, "input_dataExp"=w547) -> ()  [unwired: 9 in, 1 out]
                  n98 = call "BRig_RT_panel_Laser1_v1,18.vi"("input_setValues"=w548, "input_dataExp"=w547, "input_dataLC"=w546) -> ()  [unwired: 7 in, 2 out]
                  n99 = call "BRig_RT_panel_Laser2_v1,18.vi"("input_setValues"=w548, "input_dataExp"=w547, "input_dataLC"=w546) -> ()  [unwired: 7 in, 2 out]
                  n100 = call "BRig_RT_panel_manualTriggering_v0,90.vi"("input_dataMTrig"=w545, "input_setValues"=w548) -> ()  [unwired: 10 in, 8 out]
                }
                frame "Idle" {
                  w628 = 100.0 ("y")
                  n101 = call "BRig_dataMTrig_Solenoid_T_L.vi"() -> ("output_Solenoid_T_L"=w566:i32)  [unwired: 11 in]
                  n102 = call "BRig_dataMTrig_Solenoid_T_R.vi"() -> ("output_Solenoid_T_R"=w565:i32)  [unwired: 11 in]
                  n103 = local read "FPGA_count2ms"() -> (w564:dbl)
                  n104 = call "BRig_dataExp_L_power_min_l1.vi"() -> ("output_L_power_min_l1"=w633:i32)  [unwired: 11 in]
                  n105 = call "BRig_dataExp_L_power_min_l2.vi"() -> ("output_L_power_min_l2"=w632:i32)  [unwired: 11 in]
                  n106 = call "BRig_dataExp_LED_baseline_Cue.vi"() -> ("output_LED_baseline_Cue"=w626:i32)  [unwired: 11 in]
                  n107 = call "BRig_dataExp_LED_baseline_l1.vi"() -> ("output_LED_baseline_l1"=w625:i32)  [unwired: 11 in]
                  n108 = call "BRig_dataExp_LED_baseline_l2.vi"() -> ("output_LED_baseline_l2"=w624:i32)  [unwired: 11 in]
                  n109 = call "BRig_dataExp_CueLed_Tpeak.vi"() -> ("output_CueLed_Tpeak"=w616:i32)  [unwired: 11 in]
                  n110 = call "BRig_dataExp_CueLed_freq.vi"() -> ("output_CueLed_Freq"=w615:i32)  [unwired: 11 in]
                  n111 = call "BRig_dataExp_L_Tpeak_l1.vi"() -> ("output_L_Tpeak_l1"=w608:i32)  [unwired: 11 in]
                  n112 = call "BRig_dataExp_L_freq_l1.vi"() -> ("output_L_freq_l1"=w607:i32)  [unwired: 11 in]
                  n113 = call "BRig_dataExp_L_Tshutter_l1.vi"() -> ("output_L_Tshutter_l1"=w606:i32)  [unwired: 11 in]
                  n114 = call "BRig_RT__Case_Idle__State_Idle__getAudioParam.vi"("input_dataExp"=w582, "input_dataMTrig"=w583) -> ("output_Audio_freq_R"=w578:u8, "output_Audio_amp_R"=w579:u16, "output_Audio_freq_L"=w580:u8, "output_Audio_amp_L"=w581:u16, "output_state"=w577:T1)  [unwired: 5 in]
                  n115 = call "BRig_dataExp_L_Tpeak_l2.vi"() -> ("output_L_Tpeak_l2"=w590:i32)  [unwired: 11 in]
                  n116 = call "BRig_dataExp_L_freq_l2.vi"() -> ("output_L_freq_l2"=w589:i32)  [unwired: 11 in]
                  n117 = call "BRig_dataExp_L_Tshutter_l2.vi"() -> ("output_L_Tshutter_l2"=w588:i32)  [unwired: 11 in]
                  n118 = local read "I_sendData"() -> (w576:bool)
                  n119 = Index Array(array=w582, index #1=w633, index #2=w632, index #3=w626, index #4=w625, index #5=w624, index #6=w616, index #7=w615, index #8=w608, index #9=w607, index #10=w606, index #11=w590, index #12=w589, index #13=w588, index #14=w566, index #15=w565) -> (element #1=w631:u16, element #2=w627:u16, element #3=w623:u16, element #4=w622:u16, element #5=w621:u16, element #6=w612:u16, element #7=w611:u16, element #8=w605:u16, element #9=w604:u16, element #10=w603:u16, element #11=w593:u16, element #12=w592:u16, element #13=w591:u16, element #14=w563:u16, element #15=w562:u16)
                  n120 = Select(t=myRIO_BRig_RT__Case_NonExp_stateList."SendData" ("Enum"), s=w576, f=w577) -> (s? t:f=w573:T1)
                  n121 = To Double Precision Float(number=w563) -> (double precision float=w561:dbl)
                  n122 = To Double Precision Float(number=w562) -> (double precision float=w560:dbl)
                  n123 = To Double Precision Float(number=w631) -> (double precision float=w630:dbl)
                  n124 = To Double Precision Float(number=w627) -> (double precision float=w629:dbl)
                  n125 = To Double Precision Float(number=w612) -> (double precision float=w614:dbl)
                  n126 = To Double Precision Float(number=w611) -> (double precision float=w613:dbl)
                  n127 = To Double Precision Float(number=w605) -> (double precision float=w602:dbl)
                  n128 = To Double Precision Float(number=w604) -> (double precision float=w601:dbl)
                  n129 = To Double Precision Float(number=w603) -> (double precision float=w600:dbl)
                  n130 = To Unsigned Word Integer(number=w564) -> (unsigned 16bit integer=w617:u16)
                  n131 = To Double Precision Float(number=w593) -> (double precision float=w594:dbl)
                  n132 = To Double Precision Float(number=w592) -> (double precision float=w595:dbl)
                  n133 = To Double Precision Float(number=w591) -> (double precision float=w596:dbl)
                  n134 = Not Equal To 0?(x=w621) -> (x != 0?=w618:bool)
                  n135 = Not Equal To 0?(x=w623) -> (x != 0?=w620:bool)
                  n136 = Not Equal To 0?(x=w622) -> (x != 0?=w619:bool)
                  n137 = Divide(x=w630, y=w628) -> (x/y=w557:dbl)
                  n138 = Divide(x=w629, y=w628) -> (x/y=w556:dbl)
                  n139 = local read "get_countPerMS"() -> (w572:bool)
                  n140 = Multiply(x=w564, y=w561) -> (x*y=w570:dbl)
                  n141 = Multiply(x=w564, y=w560) -> (x*y=w568:dbl)
                  n142 = call "BRig_RT__Case_Idle__calc_FPGA_CueLed.vi"("input_FPGA_ms2count"=w564, "input_Tpeak"=w614, "input_Freq"=w613) -> ("output_laser_Npeak"=w610:u32, "output_laser_Nvalley"=w609:u32)  [unwired: 11 in]
                  n143 = call "BRig_RT__Case_Idle__calc_FPGA_laser.vi"("input_FPGA_ms2count"=w564, "input_Tpeak"=w602, "input_Freq"=w601, "input_Tshutter"=w600) -> ("output_laser_Npeak"=w599:u32, "output_laser_Nvalley"=w598:u32, "output_laser_Nshutter"=w597:u32)  [unwired: 9 in]
                  n144 = call "BRig_RT__Case_Idle__calc_FPGA_laser.vi"("input_FPGA_ms2count"=w564, "input_Tpeak"=w594, "input_Freq"=w595, "input_Tshutter"=w596) -> ("output_laser_Npeak"=w587:u32, "output_laser_Nvalley"=w586:u32, "output_laser_Nshutter"=w585:u32)  [unwired: 9 in]
                  n145 = local write "L_Power_l1"(w557) -> ()
                  n146 = local write "L_Power_l2"(w556) -> ()
                  n147 = call "myRIO__convert__Voltage_to_FPGAvalue.vi"("input_voltage"=w557) -> ("output_PortA"=w550:u16)  [unwired: 9 in, 1 out]
                  n148 = call "myRIO__convert__Voltage_to_FPGAvalue.vi"("input_voltage"=w556) -> ("output_PortA"=w551:u16)  [unwired: 9 in, 1 out]
                  n149 = Round Toward +Infinity(x=w570) -> (ceil(x): smallest int >= x=w569:dbl)
                  n150 = Round Toward +Infinity(x=w568) -> (ceil(x): smallest int >= x=w567:dbl)
                  n151 = local read "LaserFiber_V_l1"() -> (w554:dbl)
                  n152 = local read "LaserFiber_V_l2"() -> (w555:dbl)
                  n153 = To Unsigned Long Integer(number=w569) -> (unsigned 32bit integer=w559:u32)
                  n154 = To Unsigned Long Integer(number=w567) -> (unsigned 32bit integer=w558:u32)
                  n155 = Select(t=myRIO_BRig_RT__Case_NonExp_stateList."Get_FPGA_count_per_ms" ("Enum"), s=w572, f=w573) -> (s? t:f=w571:T1)
                  n156 = call "myRIO__convert__Voltage_to_FPGAvalue.vi"("input_voltage"=w554) -> ("output_PortA"=w553:u16)  [unwired: 9 in, 1 out]
                  n157 = call "myRIO__convert__Voltage_to_FPGAvalue.vi"("input_voltage"=w555) -> ("output_PortA"=w552:u16)  [unwired: 9 in, 1 out]
                  n158 = xnode "Read/Write Control"("FPGA VI Reference In"=w636, "error in"=w635, "audioAmp_L"=w581, "audioFreq_L_kHz"=w580, "audioAmp_R"=w579, "audioFreq_R_kHz"=w578, "AnaOut_0"=w550, "AnaOut_1"=w551, "CueLed_Baseline"=w620, "L1Led_Baseline"=w619, "L2Led_Baseline"=w618, "k1__counter_per_ms"=w617, "CueLed_nPeak"=w610, "CueLed_nValley"=w609, "LC_nPeak_l1"=w599, "LC_nValley_l1"=w598, "LC_nShutter_l1"=w597, "LC_nPeak_l2"=w587, "LC_nValley_l2"=w586, "LC_nShutter_l2"=w585, "Solenoid_nTotal_L"=w559, "Solenoid_nTotal_R"=w558, "AnaOut0_Pair"=w553, "AnaOut1_Pair"=w552) -> ("error out"=w634:errorcluster)  [unwired: 1 out]
                  n159 = local write "error out"(w634) -> ()
                }
                frame "Idle_2" {
                  w646 = FALSE
                  # "Get latest settings from panels"
                  n160 = call "BRig_RT_panel_cue_v1,18.vi"("input_setValues"=w646, "input_dataExp"=w640) -> ("output_dataExp"=w639:u16[])  [unwired: 9 in]
                  n161 = call "BRig_RT_panel_ExpStruct_v1,18.vi"("input_setValues"=w646, "input_dataExp"=w639) -> ("output_dataExp"=w638:u16[])  [unwired: 9 in]
                  n162 = local read "comm_TCP_connect"() -> (w645:bool)
                  n163 = call "BRig_RT_panel_Laser1_v1,18.vi"("input_setValues"=w646, "input_dataExp"=w638, "input_dataLC"=w652) -> ("output_dataExp"=w647:u16[], "output_dataLC"=w649:u16[])  [unwired: 7 in]
                  n164 = Select(t=myRIO_BRig_RT__Case_NonExp_stateList."commTCP_connect" ("Enum"), s=w645, f=myRIO_BRig_RT__Case_NonExp_stateList."Idle_6" ("Enum")) -> (s? t:f=w643:T1)
                  n165 = call "BRig_RT_panel_Laser2_v1,18.vi"("input_setValues"=w646, "input_dataExp"=w647, "input_dataLC"=w649) -> ("output_dataExp"=w637:u16[], "output_dataLC"=w648:u16[])  [unwired: 7 in]
                  n166 = local read "comm_WebDAV_connect"() -> (w644:bool)
                  n167 = Select(t=myRIO_BRig_RT__Case_NonExp_stateList."TestConnection" ("Enum"), s=w644, f=w643) -> (s? t:f=w641:T1)
                }
                frame "Idle_6" {
                  # "Received new experimental settings?"
                  n168 = local read "lick_Rising(F)_or_Falling(T)"() -> (w654:bool)
                  n169 = call "BRig_RT__Case_Idle__State_UploadSettings_checkFile.vi"("input_dataName"="dataExp") -> ("output_Iexist"=w663:bool)  [unwired: 9 in, 1 out]
                  n170 = xnode "Read/Write Control"("FPGA VI Reference In"=w656, "error in"=w655, "Rising(F)_or_Falling(T)"=w654) -> ()  [unwired: 2 out]
                  n171 = Select(t=myRIO_BRig_RT__Case_NonExp_stateList."UploadSettings_pre" ("Enum"), s=w663, f=myRIO_BRig_RT__Case_NonExp_stateList."Idle") -> (s? t:f=w661:T1)
                }
                frame "Cue_pre" {
                  n172 = call "BRig_RT__Case_Idle__State_Cue_pre__v2.vi"("input_dataExp"=w665, "input_dataMTrig"=w669) -> ("output_dataMTrig"=w668:u16[], "output_state"=w667:T1)  [unwired: 8 in]
                }
                frame "Cue" {
                  n173 = call "BRig_RT__Case_Idle__State_Cue__v2.vi"("input_cLick_R_prev"=w672, "input_cLick_R"=w673, "input_state"=w678, "input_cLick_L_prev"=w674, "input_cLick_L"=w675, "input_dataMTrig"=w679) -> ("output_dataMTrig"=w677:u16[], "output_state"=w676:T1)  [unwired: 4 in]
                }
                frame "RewardCalibration_pre" {
                  n174 = call "BRig_RT__Case_Idle__State_RewardCalibration_pre__v2.vi"("input_dataMTrig"=w681) -> ("output_dataMTrig"=w680:u16[])  [unwired: 26 in]
                }
                frame "RewardCalibration" {
                  n175 = call "BRig_RT__Case_Idle__State_RewardCalibration.vi"("input_state"=w686, "input_dataMTrig"=w688) -> ("output_dataMtrig"=w687:u16[], "output_state"=w685:T1)  [unwired: 8 in]
                }
                frame "TestConnection" {
                  n176 = local read "Host Password"() -> (w694:string)
                  n177 = local read "Host UserName"() -> (w695:string)
                  n178 = call "BRig_RT_comm_webdav_connect.vi"("input_password"=w694, "input_username"=w695) -> ("output_Iconnected"=w693:bool, "output_hSession"=w692:T4)  [unwired: 6 in, 2 out]
                  n179 = local write "comm_WebDAV_connect"(FALSE ("comm_WebDAV_connect")) -> ()
                  n180 = local write "comm_WebDAV"(w693) -> ()
                }
                frame "SendData" {
                  n181 = And(x=w704, y=w703) -> (x .and. y?=w702:bool)
                  n182 = case shown="True" w702 {
                    tunnel: w703 -> [_ w721]
                    tunnel: w709 -> [_ w720]
                    tunnel: w708 -> [_ w719]
                    tunnel: w706 -> [_ w717]
                    tunnel: w705 -> [_ w716]
                    frame False {
                      n183 = One Button Dialog(message="Unable to send data:\n Missing one or more\n connections") -> ()  [unwired: 1 in, 1 out]
                    }
                    frame True {
                      n184 = local read "Data Set Prefix"() -> (w722:string)
                      n185 = call "BRig_RT_comm_webdav_upload_all__v3.vi"("input_I_connected_webdav"=w721, "input_fileName_prefix"=w722, "input_hSession"=w720, "input_error"=w719, "input_True"=TRUE) -> ("output_nFilenames"=w723:i32, "output_arrFilenames"=w724:string[], "output_uploaded"=w725:bool[], "output_strCmd"=w718:string)  [unwired: 5 in, 2 out]
                      n186 = call "BRig_RT_comm_tcp_write_RTwrite.vi"("input_error"=w716, "input_packet"=w718, "input_hTCP"=w717) -> ()  [unwired: 5 in, 4 out]
                      n187 = call "BRig_RT_comm_webdav_upload_all_warnUser.vi"("input_n"=w723, "input_arrFilenames"=w724, "input_arrUploaded"=w725) -> ()  [unwired: 9 in]
                    }
                  }
                  n188 = local write "I_sendData"(FALSE ("I_sendData")) -> ()
                }
                frame "Get_FPGA_count_per_ms" {
                  # "Used to automatically determine how many FPGA cycles in 1 ms"
                  n189 = case shown="True" w738 {
                    selector: w738 -> [w740 _]
                    tunnel: w736 -> [_ w753]
                    tunnel: [w744 w753] -> w735
                    tunnel: w734 -> [w743 w751]
                    tunnel: w733 -> [w742 w750]
                    tunnel: [w741 w748] -> w728
                    tunnel: [w740 w747] -> w732
                    frame False {
                      n190 = Get Date/Time In Seconds() -> (seconds since 1Jan1904=w745:timestamp)
                      n191 = To Double Precision Float(number=w745) -> (double precision float=w744:dbl)
                      n192 = xnode "Read/Write Control"("FPGA VI Reference In"=w743, "error in"=w742, "timeTrial_trig"=TRUE ("timeTrial")) -> ("error out"=w741:errorcluster)  [unwired: 1 out]
                      n193 = local write "get_countPerMS"(w740) -> ()
                    }
                    frame True {
                      w749 = 1.0
                      # "units are\nseconds"
                      n194 = Get Date/Time In Seconds() -> (seconds since 1Jan1904=w754:timestamp)
                      n195 = To Double Precision Float(number=w754) -> (double precision float=w755:dbl)
                      n196 = Subtract(x=w755, y=w753) -> (x-y=w752:dbl)
                      n197 = Less Or Equal?(x=w749, y=w752) -> (x <= y?=w747:bool)
                      n198 = case shown="True" w747 {
                        tunnel: w751 -> [_ w768]
                        tunnel: w750 -> [w756 w767]
                        tunnel: w749 -> [_ w758]
                        tunnel: [w756 w757] -> w748
                        frame False {
                        }
                        frame True {
                          n199 = xnode "Read/Write Control"("FPGA VI Reference In"=w768, "error in"=w767) -> ("FPGA VI Reference Out"=w765:refnum<k20>, "error out"=w764:errorcluster, "timeTrial_count"=w759:u32)
                          n200 = Multiply(x=w758, y=1000.0) -> (x*y=w762:dbl)
                          n201 = To Double Precision Float(number=w759) -> (double precision float=w761:dbl)
                          n202 = Divide(x=w761, y=w762) -> (x/y=w763:dbl)
                          n203 = local write "FPGA_count2ms"(w763) -> ()
                          n204 = xnode "Read/Write Control"("FPGA VI Reference In"=w765, "error in"=w764, "timeTrial_trig"=FALSE ("timeTrial")) -> ("error out"=w757:errorcluster)  [unwired: 1 out]
                        }
                      }
                    }
                  }
                  n205 = Select(t=myRIO_BRig_RT__Case_NonExp_stateList."Idle" ("Enum"), s=w732, f=w730) -> (s? t:f=w729:T1)
                  n206 = local write "error out"(w728) -> ()
                }
                frame "End" {
                }
                frame "commTCP_connect" {
                  n207 = case shown="True" w785 {
                    tunnel: w784 -> [w795 w804]
                    tunnel: [w794 w800] -> w782
                    tunnel: [w793 w797] -> w774
                    tunnel: [w792 w798] -> w783
                    tunnel: w781 -> [_ w805]
                    frame False {
                      n208 = call "BRig_RT_comm_tcp_connect_RTwrite.vi"("input_error"=w795) -> ("output_error"=w792:errorcluster, "output_connected"=w793:bool, "output_hTCP"=w794:refnum<k5>)  [unwired: 8 in]
                    }
                    frame True {
                      n209 = call "BRig_RT_comm_tcp_write_RTwrite.vi"("input_error"=w804, "input_packet"="<test>", "input_hTCP"=w805) -> ("output_error"=w799:errorcluster, "output_I_NotDisconnected"=w796:bool, "output_I_write"=w802:bool, "output_hTCP"=w801:refnum<k5>)  [unwired: 5 in]
                      n210 = case shown="False" w802 {
                        selector: w802 -> [_ w816]
                        tunnel: w801 -> [w811 w818]
                        tunnel: [w806 w818] -> w800
                        tunnel: w799 -> [w810 w817]
                        tunnel: [w808 w817] -> w798
                        tunnel: [w807 w816] -> w797
                        tunnel: w796 -> [w812 _]
                        frame False {
                          n211 = case shown="True" w812 {
                            tunnel: w811 -> [_ w815]
                            tunnel: w810 -> [w813 w814]
                            tunnel: [w813 w814] -> w809
                            frame False {
                            }
                            frame True {
                              n212 = TCP Close Connection(connection ID=w815, error in (no error)=w814) -> ()  [unwired: 1 in, 2 out]
                            }
                          }
                          n213 = call "BRig_RT_comm_tcp_connect_RTwrite.vi"("input_error"=w809) -> ("output_error"=w808:errorcluster, "output_connected"=w807:bool, "output_hTCP"=w806:refnum<k5>)  [unwired: 8 in]
                        }
                        frame True {
                        }
                      }
                    }
                  }
                  n214 = local read "comm_TCP_connect"() -> (w778:bool)
                  n215 = Not(x=w778) -> (.not. x?=w777:bool)
                  n216 = Or(x=w777, y=w774) -> (x .or. y?=w776:bool)
                  n217 = case shown="True" w776 {
                    tunnel: [w789 myRIO_BRig_RT__Case_NonExp_stateList."Idle" ("Enum")] -> w780
                    tunnel: w779 -> [w789 _]
                    frame False {
                    }
                    frame True {
                      n218 = local write "comm_TCP_connect"(FALSE) -> ()
                    }
                  }
                  n219 = local write "comm_TCP"(w774) -> ()
                }
              }
              n220 = case shown="True" w397 {
                tunnel: [w455 w456] -> w400
                tunnel: [w454 w457] -> w399
                tunnel: [w453 w458] -> w398
                tunnel: w396 -> [w455 _]
                tunnel: w395 -> [w454 _]
                tunnel: w394 -> [w453 _]
                tunnel: w393 -> [_ w458]
                tunnel: w392 -> [_ w457]
                tunnel: w391 -> [_ w456]
                frame False {
                }
                frame True {
                }
              }
              n221 = case shown="True" w387 {
                tunnel: [w449 w450] -> w386
                tunnel: [w448 w451] -> w385
                tunnel: [w447 w452] -> w384
                tunnel: w388 -> [w449 _]
                tunnel: w389 -> [w448 _]
                tunnel: w390 -> [w447 _]
                tunnel: w382 -> [_ w452]
                tunnel: w381 -> [_ w451]
                tunnel: w383 -> [_ w450]
                frame False {
                }
                frame True {
                }
              }
              n222 = flat-sequence {
                tunnel: w420 -> [w462]
                tunnel: w418 -> [w460]
                tunnel: [w462] -> w424
                tunnel: [w461] -> w423
                tunnel: [w460] -> w422
                tunnel: [w459] -> w421
                tunnel: w417 -> [w459]
                tunnel: [w474] -> w419
                tunnel: w424 -> [w474]
                tunnel: w423 -> [w473]
                tunnel: w422 -> [w471]
                tunnel: w421 -> [w466]
                tunnel: [w465] -> w416
                frame #0 {
                  n223 = Get Date/Time In Seconds() -> (seconds since 1Jan1904=w461:timestamp)
                }
                frame #1 {
                  # "threshold"
                  # "delta T [ms]"
                  # "delta T [s]"
                  n224 = To Double Precision Float(number=w473) -> (double precision float=w472:dbl)
                  n225 = To Double Precision Float(number=w471) -> (double precision float=w470:dbl)
                  n226 = Subtract(x=w472, y=w470) -> (x-y=w469:dbl)
                  n227 = Multiply(x=w469, y=1000.0) -> (x*y=w464:dbl)
                  n228 = Greater?(x=w464, y=5.0) -> (0:w463:bool)
                  n229 = local write "Threshold"(w463) -> ()
                  n230 = local write "tLoop"(w464) -> ()
                  n231 = Or(x=w463, y=w466) -> (x .or. y?=w465:bool)
                }
              }
              n232 = local read "START"() -> (w441:bool)
              n233 = local read "STOP_abort"() -> (w440:bool)
              n234 = local read "Laser1_LED"() -> (w378:bool)
              n235 = local read "Laser2_LED"() -> (w377:bool)
              n236 = call "BRig_RT_panel_manualTriggering_v0,90.vi"("input_dataMTrig"=w405) -> ("output_Solenoid_R"=w408:bool, "output_Solenoid_L"=w409:bool, "output_dataMTrig"=w415:u16[], "output_Audio_L"=w410:bool, "output_Audio_R"=w411:bool, "output_CueLed"=w412:bool, "output_Laser_l1"=w413:bool, "output_Laser_l2"=w414:bool)  [unwired: 11 in]
              n237 = Or(x=w441, y=w440) -> (x .or. y?=w439:bool)
              n238 = Select(t=myRIO_BRig_RT__Case_NonExp_stateList."End" ("Enum"), s=w439, f=w438) -> (s? t:f=w437:T1)
              n239 = xnode "Read/Write Control"("FPGA VI Reference In"=w432, "error in"=w431, "A1_SR"=w408, "A3_SL"=w409, "audioTrigger_L"=w410, "audioTrigger_R"=w411, "LC_Laser_l1"=w413, "LC_Laser_l2"=w414, "CueLed_Event"=w412, "L1Led_ON"=w378, "L2Led_ON"=w377) -> ("FPGA VI Reference Out"=w443:refnum<k20>, "error out"=w420:errorcluster, "fpga_laser1"=w373:bool, "fpga_laser2"=w374:bool, "fpga_solenoid_L"=w375:bool, "fpga_solenoid_R"=w376:bool)
              n240 = local write "Laser1"(w373) -> ()
              n241 = local write "Laser2"(w374) -> ()
              n242 = local write "Solenoid L"(w375) -> ()
              n243 = local write "Solenoid R"(w376) -> ()
              n244 = node-c288() -> ()  [unwired: 1 in, 1 out]
            }
            n245 = node-c288(w368) -> ()  [unwired: 1 out]
            n246 = flat-sequence {
              tunnel: w362 -> [w372]
              tunnel: [w372] -> w361
              tunnel: w360 -> [w371]
              tunnel: [w371] -> w359
              frame #0 {
                w370 = FALSE
                n247 = local write "STOP_endBlock"(w370) -> ()
                n248 = local write "STOP_endTrial"(w370) -> ()
              }
            }
          }
          frame True {
            w899 = ".csv" ("string")
            w929 = ""
            w938 = u8 0
            w939 = u16 0 ("AudioLeft_phase_inc")
            w940 = FALSE
            # "empty AnaIn array"
            # "Initialize data share\nbetween timed loop and\nTrial/Block Status loop"
            # "Initialize data share\nbetween timed loop\nand analog input loop"
            # "buffer_dataRT_stats"
            # "Clear local files"
            # "empty array"
            # "buffer_dataBlock"
            # "buffer_dataTrial"
            # "nColumns dataBlock"
            # "nColumns dataTrial"
            # "buffer_dataBlock"
            # "buffer_dataTrial"
            # "nColumns\ndataBlock"
            # "nColumns\ndataTrial"
            # "original dataExp and dataLC"
            # "dataLick"
            # "dataTrial"
            # "dataBlock"
            # "dataCurrent"
            # "arrTrig"
            # "time stamp"
            # "dummyState counter"
            # "dataTrial"
            # "dataLick"
            # "dataLC"
            # "dataLC"
            # "dataBlock"
            # "dataMTrig"
            # "dataMTrig"
            # "dataExp"
            # "dataExp"
            # "dataCurrent"
            # "state"
            n249 = flat-sequence {
              tunnel: [w1036] -> w869
              tunnel: [w1035] -> w873
              tunnel: [w1044] -> w887
              tunnel: [w1043] -> w886
              tunnel: [myRIO_BRig_RT__Case_Exp_stateList."Start1" ("Enum")] -> w885
              tunnel: [w1041] -> w884
              tunnel: [u16 0] -> w883
              tunnel: [w1039] -> w882
              tunnel: [w1038] -> w881
              tunnel: [w1037] -> w880
              tunnel: w887 -> [w1053]
              tunnel: w886 -> [w1052]
              tunnel: w885 -> [w1051]
              tunnel: w884 -> [w1050]
              tunnel: w883 -> [w1049]
              tunnel: w882 -> [w1048]
              tunnel: w881 -> [w1047]
              tunnel: w880 -> [w1046]
              tunnel: [w1053] -> w834
              tunnel: [w1052] -> w833
              tunnel: [w1051] -> w832
              tunnel: [w1050] -> w831
              tunnel: [w1049] -> w830
              tunnel: [w1048] -> w829
              tunnel: [w1047] -> w828
              tunnel: [w1046] -> w827
              tunnel: [w1045] -> w826
              tunnel: [w1058] -> w878
              tunnel: [w1059] -> w895
              tunnel: [w1060] -> w896
              tunnel: [w1061] -> w946
              tunnel: [w1062] -> w948
              tunnel: [w1063] -> w949
              tunnel: [w1064] -> w950
              tunnel: [w1065] -> w951
              tunnel: [w1066] -> w952
              tunnel: w834 -> [w1066]
              tunnel: w833 -> [w1065]
              tunnel: w832 -> [w1064]
              tunnel: w831 -> [w1063]
              tunnel: w830 -> [w1062]
              tunnel: w829 -> [w1061]
              tunnel: w828 -> [w1060]
              tunnel: w827 -> [w1059]
              tunnel: w826 -> [w1058]
              tunnel: [w1054] -> w825
              frame #0 {
                n250 = call "BRig_dataBlock_init.vi"() -> ("output_nCol"=w1035:i32, "output_dataBlock"=w1037:u16[][])  [unwired: 10 in]
                n251 = call "BRig_dataCurrent_init.vi"() -> ("output_dataCurrent"=w1044:u16[])  [unwired: 11 in]
                n252 = Get Date/Time In Seconds() -> (seconds since 1Jan1904=w1034:timestamp)
                n253 = call "BRig_dataLick_init.vi"() -> ("output_dataLick"=w1043:u16[][])  [unwired: 11 in]
                n254 = call "BRig_dataTrial_init.vi"() -> ("output_nCol"=w1036:i32, "output_dataTrial"=w1038:u16[][])  [unwired: 10 in]
                n255 = To Double Precision Float(number=w1034) -> (double precision float=w1041:dbl)
                n256 = call "BRig_arrTrig_init.vi"() -> ("output_arrTrig"=w1039:bool[])  [unwired: 11 in]
              }
              frame #1 {
                w1045 = u32 2 ("milliseconds to wait")
                n257 = Wait (ms)(milliseconds to wait=w1045) -> ()  [unwired: 1 out]
              }
              frame #2 {
                # "uint16 or\ninit16"
                # "AnaIn\narray"
                n258 = Initialize Array(u16 0 ("milliseconds to wait"), 5 ("dimension size"), 2 ("dimension size")) -> (w1054:u16[][])
              }
            }
            n259 = flat-sequence {
              tunnel: w875 -> [w1015]
              tunnel: [w1015] -> w874
              tunnel: w874 -> [w1024]
              tunnel: [w1022] -> w857
              tunnel: [w1021] -> w844
              tunnel: [w1018] -> w872
              tunnel: w873 -> [w1017]
              tunnel: w869 -> [w1016]
              tunnel: [w1024] -> w871
              tunnel: w871 -> [w1026]
              tunnel: [w1026] -> w870
              tunnel: w870 -> [w1032]
              tunnel: w869 -> [w1031]
              tunnel: [w1029] -> w864
              tunnel: [w1027] -> w867
              tunnel: [w1032] -> w868
              tunnel: [w1033] -> _
              tunnel: w868 -> [w1033]
              frame #0 {
                n260 = Wait (ms)(milliseconds to wait=w1015) -> ()  [unwired: 1 out]
              }
              frame #1 {
                w1019 = u16 0 ("element")
                n261 = Initialize Array(w1019, 16 ("dimension size")) -> (w1022:u16[])
                n262 = Initialize Array(w1019, 100 ("dimension size"), w1016) -> (w1021:u16[][])
                n263 = Initialize Array(w1019, 10 ("dimension size"), w1017) -> (w1018:u16[][])
              }
              frame #2 {
                n264 = Wait (ms)(milliseconds to wait=w1026) -> ()  [unwired: 1 out]
              }
              frame #3 {
                n265 = Increment(x=w1031) -> (x+1=w1028:i32)
                n266 = To Unsigned Long Integer(number=w1028) -> (unsigned 32bit integer=w1027:u32)
                n267 = Initialize Array(u16 0 ("element"), w1028) -> (w1029:u16[])
              }
              frame #4 {
                n268 = Wait (ms)(milliseconds to wait=w1033) -> ()  [unwired: 1 out]
              }
            }
            n269 = call "BRig_comm_webdav_myrioFolder.vi"() -> ("output_myrioFolder"=w900:string)  [unwired: 11 in]
            n270 = local write "stop_TimedLoop"(FALSE ("stop_TimedLoop")) -> ()
            n271 = RT FIFO Create(0:"dataTrialOrBlock" ("name (unnamed)"), 1:w864, 4:u32 40 ("size (10)"), 6:w867, 7:T8 {"read mode"=enum."blocking", "write mode"=enum."blocking"} ("r/w modes (polling,polling)")) -> (8:w866:refnum<k33>, 11:w865:errorcluster)  [unwired: 3 in, 1 out]
            n272 = RT FIFO Create(0:"dataAnalog" ("name (unnamed)"), 1:u16 0 ("element"), 4:u32 4000 ("size (10)")) -> (8:w852:refnum<k33>, 11:w851:errorcluster)  [unwired: 5 in, 1 out]
            n273 = Concatenate Strings(w900, "dataTrial" ("input_filename"), w899) -> (w901:string)
            n274 = Concatenate Strings(w900, "dataBlock" ("input_filename"), w899) -> (w902:string)
            n275 = String To Path(string=w901) -> (path=w905:path)
            n276 = String To Path(string=w902) -> (path=w897:path)
            n277 = flat-sequence {
              tunnel: [w1067] -> w879
              tunnel: w878 -> [w1067]
              tunnel: w879 -> [w1068]
              tunnel: [w1068] -> w876
              tunnel: w892 -> [w1071]
              tunnel: w845 -> [w1070]
              tunnel: [w1069] -> w877
              tunnel: w876 -> [w1069]
              tunnel: [w1075] -> _
              tunnel: w891 -> [w1075]
              tunnel: w890 -> [w1074]
              tunnel: w889 -> [w1073]
              tunnel: [w1072] -> w875
              tunnel: w877 -> [w1072]
              frame #0 {
                n278 = call "BRig_RT__Case_Exp__clearLocalFolder.vi"() -> ()  [unwired: 12 in]
              }
              frame #1 {
                n279 = Wait (ms)(milliseconds to wait=w1068) -> ()  [unwired: 1 out]
              }
              frame #2 {
                n280 = call "BRig_RT__Case_Exp__State_start__sendExpData_saveData.vi"("input_dataLC"=w1071, "input_dataExp"=w1070) -> ()  [unwired: 10 in]
              }
              frame #3 {
                n281 = call "BRig_RT__Case_Exp__State_start__sendExpData_uploadData__v2.vi"("input_error"=w1075, "input_hSession"=w1074, "input_connected"=w1073) -> ()  [unwired: 8 in, 1 out]
              }
            }
            n282 = call "BRig_RT__Case_Exp__comm_tcp__data_other.vi"("input_strState"=w929, "input_strAccum"=w929, "input_error"=w934, "input_hTCP"=w935, "input_I_connected_TCP"=w936) -> ("output_strAccum"=w930:string, "output_error"=w931:errorcluster, "output_hTCP"=w932:refnum<k5>, "output_I_connect_TCP"=w933:bool)  [unwired: 3 in]
            n283 = Initialize Array(u16 0 ("element"), 60 ("dimension size")) -> (w839:u16[])
            n284 = node-c288() -> (w958:T5)  [unwired: 4 in]
            n285 = timed-loop {
              timing: w958 -> [_]
              timing-out: [_] -> w957
              shift-right: [w1380] -> _
              shift-left: w950 -> [w1337]
              tunnel: w945 -> [w1424]
              tunnel: w944 -> [w1404]
              shift-right: [w1368] -> _
              shift-left: w956 -> [w1423]
              shift-right: [w1367] -> _
              shift-left: w955 -> [w1422]
              tunnel: [w1415] -> w937
              tunnel: [w1416] -> w954
              shift-right: [w1378] -> w925
              shift-left: w952 -> [w1354]
              shift-right: [w1421] -> w926
              shift-left: w845 -> [w1356]
              shift-right: [w1398] -> w928
              shift-left: w942 -> [w1357]
              shift-right: [w1419] -> _
              shift-left: w895 -> [w1420]
              shift-right: [w1417] -> w927
              shift-left: w892 -> [w1418]
              shift-right: [w1374] -> w924
              shift-left: w951 -> [w1381]
              shift-right: [w1414] -> _
              shift-left: w896 -> [w1355]
              tunnel: w949 -> [w1413]
              shift-right: [w1387] -> _
              shift-left: u16 0 -> [w1386]
              shift-right: [w1407] -> _
              shift-left: w948 -> [w1408]
              shift-right: [w1405] -> _
              shift-left: w946 -> [w1406]
              shift-right: [w1399] -> _
              shift-left: FALSE -> [w1401]
              shift-right: [w1345] -> w916
              shift-left: w933 -> [w1362]
              shift-right: [w1344] -> w915
              shift-left: w932 -> [w1361]
              shift-right: [w1342] -> w914
              shift-left: w931 -> [w1360]
              shift-right: [w1343] -> _
              shift-left: w930 -> [w1359]
              shift-right: [w1351] -> w921
              shift-left: w891 -> [w1351]
              shift-right: [w1353] -> w919
              shift-left: w889 -> [w1353]
              shift-right: [w1352] -> w920
              shift-left: w890 -> [w1352]
              shift-right: [w1350] -> _
              shift-left: _ -> [w1348]
              shift-right: [w1349] -> _
              shift-left: _ -> [w1347]
              tunnel: [w1346] -> w908
              tunnel: w866 -> [w1340]
              tunnel: w865 -> [w1339]
              tunnel: w864 -> [w1338]
              tunnel: w852 -> [w1336]
              tunnel: w851 -> [w1335]
              tunnel: w845 -> [w1334]
              tunnel: w825 -> [w1327]
              shift-right: [w1310] -> _
              shift-left: TRUE -> [w1311]
              stop <- w1346 stop-if-true
              w1319 = 1 ("milliseconds to wait")
              w1325 = 0 ("milliseconds to wait")
              w1320 = 4 ("milliseconds to wait")
              w1321 = 3 ("milliseconds to wait")
              w1322 = 2 ("milliseconds to wait")
              w1323 = 1 ("milliseconds to wait")
              w1324 = 0 ("milliseconds to wait")
              # "send TCP message"
              # "dataCurrent"
              # "package\nanalog input\nand send\nto another loop"
              # "arrTrig"
              # "time stamp"
              # "dummyState counter"
              # "dataTrial"
              # "dataLC"
              # "dataBlock"
              # "dataExp"
              # "dataCurrent"
              # "state"
              # "iOccurrence"
              # "resetOccurrence?\ndataAnalog"
              # "dataLick"
              # "dataLick"
              # "dummyState counter"
              # "iOccurrence"
              # "arrTrig"
              # "CueLed"
              # "LC_Laser_l2"
              # "LC_Event_l2"
              # "LC_Laser_l1"
              # "LC_Event_l1"
              # "iState\n(start and end)"
              # "manual triggering"
              # "dataTrial"
              # "dataBlock"
              # "dataExp"
              # "dataCurrent"
              # "audio__L\naudio__R"
              # "dataLC"
              # "solenoid__R"
              # "solenoid__L"
              # "Did a lick occur?"
              # "state"
              n286 = node-c288() -> ()  [unwired: 1 in, 1 out]
              n287 = flat-sequence {
                tunnel: w1404 -> [w1425]
                tunnel: [w1426] -> w1402
                tunnel: [w1425] -> w1403
                frame #0 {
                  n288 = Get Date/Time In Seconds() -> (seconds since 1Jan1904=w1426:timestamp)
                }
              }
              n289 = xnode "Read/Write Control"("FPGA VI Reference In"=w1424, "error in"=w1403, "AI_newCycleFlag"=w1311) -> ("FPGA VI Reference Out"=w1410:refnum<k20>, "error out"=w1409:errorcluster, "A2_LickL"=w1368:u32, "A4_LickR"=w1367:u32, "AnaIn_0_0"=w1326:u16, "AnaIn_0_1"=w1318:u16, "AnaIn_0_2"=w1317:u16, "AnaIn_0_3"=w1316:u16, "AnaIn_0_4"=w1308:u16, "AnaIn_1_0"=w1315:u16, "AnaIn_1_1"=w1314:u16, "AnaIn_1_2"=w1313:u16, "AnaIn_1_3"=w1312:u16, "AnaIn_1_4"=w1309:u16)
              n290 = local write "A2"(w1368) -> ()
              n291 = local write "A4"(w1367) -> ()
              n292 = Replace Array Subset(array=w1327, new element #1=w1326, index (row) #1=w1324, index (col) #1=w1325, new element #2=w1318, index (row) #2=w1323, index (col) #2=w1325, new element #3=w1317, index (row) #3=w1322, index (col) #3=w1325, new element #4=w1316, index (row) #4=w1321, index (col) #4=w1325, new element #5=w1308, index (row) #5=w1320, index (col) #5=w1325, new element #6=w1315, index (row) #6=w1324, index (col) #6=w1319, new element #7=w1314, index (row) #7=w1323, index (col) #7=w1319, new element #8=w1313, index (row) #8=w1322, index (col) #8=w1319, new element #9=w1312, index (row) #9=w1321, index (col) #9=w1319, new element #10=w1309, index (row) #10=w1320, index (col) #10=w1319) -> (w1307:u16[][])
              n293 = local write "cState"(w1337) -> ()
              n294 = Greater?(x=w1368, y=w1423) -> (0:w1376:bool)
              n295 = Greater?(x=w1367, y=w1422) -> (0:w1375:bool)
              n296 = Or(x=w1376, y=w1375) -> (x .or. y?=w1377:bool)
              n297 = case shown="\"endTrial2\"" w1337 {
                selector: w1337 -> [_ _ _ _ _ _ _ _ _ _ _ _ _ _ w1734 w1750 _ w1779 _ _ w1858 w1885 _ w1911 _ w1955 _ w2052 _ w2071 _ _ w2223 w2233 _ _ _ _ w2369 _ w2393 w2424 w2445 w2470 _ w2535 w2545 _]
                tunnel: [myRIO_BRig_RT__Case_Exp_stateList."Start2" ("Enum") myRIO_BRig_RT__Case_Exp_stateList."Start3" ("Enum") myRIO_BRig_RT__Case_Exp_stateList."saveSettings1" ("Enum") myRIO_BRig_RT__Case_Exp_stateList."initBlock" ("Enum") myRIO_BRig_RT__Case_Exp_stateList."initTrial_LC_ENL1" ("Enum") myRIO_BRig_RT__Case_Exp_stateList."initTrial" ("Enum") myRIO_BRig_RT__Case_Exp_stateList."initTrial2" ("Enum") myRIO_BRig_RT__Case_Exp_stateList."setSettings_Laser" ("Enum") myRIO_BRig_RT__Case_Exp_stateList."ENL1_pre" ("Enum") myRIO_BRig_RT__Case_Exp_stateList."initTrial_LC_Cue1" ("Enum") myRIO_BRig_RT__Case_Exp_stateList."initTrial_LC_Sel" ("Enum") myRIO_BRig_RT__Case_Exp_stateList."initTrial4" ("Enum") w1713 w1724 w1732 w1748 myRIO_BRig_RT__Case_Exp_stateList."ENL1Penalty" ("Enum") w1777 w1792 w1815 w1857 w1884 myRIO_BRig_RT__Case_Exp_stateList."Cue1Penalty" ("Enum") w1912 w1928 w1950 myRIO_BRig_RT__Case_Exp_stateList."SelectReward" ("Enum") w2051 myRIO_BRig_RT__Case_Exp_stateList."SelectRewardPost" ("Enum") w2070 myRIO_BRig_RT__Case_Exp_stateList."SelectWrong" ("Enum") myRIO_BRig_RT__Case_Exp_stateList."SelectTimeout" ("Enum") w2222 w2232 myRIO_BRig_RT__Case_Exp_stateList."saveData_dataTrial" ("Enum") w2267 w2311 w2358 w2369 myRIO_BRig_RT__Case_Exp_stateList."initBlock" ("Enum") w2391 w2425 w2444 w2469 myRIO_BRig_RT__Case_Exp_stateList."FreeReward" ("Enum") w2533 w2543 myRIO_BRig_RT__Case_Exp_stateList."FreeRewardPost" ("Enum")] -> w1380
                tunnel: w1377 -> [_ _ _ _ _ _ _ _ _ _ _ _ w1714 w1725 w1733 w1749 _ _ w1793 w1816 w1859 w1886 _ _ _ _ _ _ _ _ _ _ _ _ _ _ _ _ _ _ _ _ _ _ _ _ _ _]
                tunnel: w1376 -> [_ _ _ _ _ _ _ _ _ _ _ _ _ _ _ _ _ _ _ _ _ _ _ _ w1921 w1951 _ _ _ _ _ _ _ _ _ _ _ _ _ _ _ _ _ _ _ _ _ _]
                tunnel: w1375 -> [_ _ _ _ _ _ _ _ _ _ _ _ _ _ _ _ _ _ _ _ _ _ _ _ w1920 w1952 _ _ _ _ _ _ _ _ _ _ _ _ _ _ _ _ _ _ _ _ _ _]
                tunnel: w1354 -> [w1436 w1442 w1484 w1511 w1514 w1587 w1601 w1620 w1647 w1672 w1682 w1699 w1712 w1723 w1741 w1757 w1768 w1776 w1794 w1817 w1860 w1887 w1904 w1910 w1931 w1948 w1991 w2049 w2061 w2069 w2099 w2170 w2221 w2231 w2247 w2273 w2319 w2348 w2368 w2375 w2394 w2427 w2443 w2460 w2505 w2531 w2542 w2553]
                tunnel: w1356 -> [w1427 w1441 w1474 w1509 w1515 w1586 w1589 w1619 w1641 w1671 w1681 w1691 w1706 w1719 w1744 w1760 w1767 w1784 w1785 w1797 w1863 w1890 w1897 w1918 w1919 w1947 w1977 w2050 w2059 w2076 w2082 w2153 w2228 w2238 w2239 w2265 w2300 w2331 w2359 w2372 w2396 w2429 w2455 w2475 w2488 w2536 w2546 w2552]
                tunnel: [w1436 w1442 w1484 w1511 w1514 w1585 w1600 w1615 w1647 w1675 w1689 w1698 w1705 w1726 w1740 w1756 w1769 w1775 w1786 w1812 w1843 w1870 w1903 w1909 w1927 w1949 w1964 w2053 w2060 w2067 w2093 w2164 w2219 w2230 w2249 w2273 w2319 w2348 w2368 w2375 w2394 w2427 w2443 w2460 w2511 w2532 w2541 w2551] -> w1379
                tunnel: [w1427 w1441 w1473 w1509 w1515 w1586 w1589 w1619 w1641 w1671 w1681 w1691 w1706 w1719 w1744 w1760 w1767 w1784 w1785 w1797 w1863 w1890 w1897 w1918 w1919 w1947 w1977 w2050 w2059 w2076 w2082 w2153 w2228 w2238 w2239 w2262 w2307 w2334 w2359 w2372 w2396 w2429 w2455 w2475 w2489 w2536 w2546 w2552] -> w1421
                tunnel: [_ _ _ _ _ _ _ _ _ _ _ _ _ _ _ _ _ _ _ _ _ _ _ _ _ _ _ w2043 _ _ _ _ _ _ _ _ _ _ _ _ _ _ _ _ _ w2525 _ _] -> w1364
                tunnel: [_ _ _ _ _ _ _ _ _ _ _ _ _ _ _ _ _ _ _ _ _ _ _ _ _ _ _ w2042 _ _ _ _ _ _ _ _ _ _ _ _ _ _ _ _ _ w2526 _ _] -> w1363
                tunnel: w1420 -> [w1435 w1439 w1482 w1513 w1546 w1583 w1605 w1633 w1658 w1677 w1688 w1696 w1716 w1728 w1743 w1759 w1764 w1782 w1796 w1819 w1862 w1889 w1902 w1915 w1937 w1959 w1990 w2054 w2065 w2074 w2097 w2168 w2226 w2237 w2243 w2274 w2309 w2350 w2366 w2374 w2376 w2430 w2453 w2473 w2514 w2538 w2548 w2560]
                tunnel: [w1435 w1439 w1482 w1513 w1546 w1582 w1604 w1633 w1658 w1677 w1688 w1696 w1716 w1728 w1743 w1759 w1764 w1782 w1796 w1819 w1862 w1889 w1902 w1915 w1937 w1959 w1989 w2054 w2065 w2074 w2096 w2167 w2226 w2237 w2243 w2274 w2309 w2350 w2366 w2374 w2376 w2430 w2453 w2473 w2514 w2538 w2548 w2560] -> w1419
                tunnel: w1418 -> [w1428 w1440 w1483 w1512 w1541 w1588 w1612 w1634 w1659 w1676 w1683 w1697 w1715 w1727 w1742 w1758 w1765 w1783 w1795 w1818 w1861 w1888 w1901 w1917 w1936 w1960 w1966 w2041 w2056 w2075 w2077 w2148 w2227 w2236 w2256 w2264 w2320 w2352 w2367 w2371 w2395 w2428 w2454 w2474 w2515 w2539 w2549 w2561]
                tunnel: [w1428 w1440 w1483 w1512 w1541 w1588 w1612 w1634 w1659 w1676 w1683 w1697 w1715 w1727 w1742 w1758 w1765 w1783 w1795 w1818 w1861 w1888 w1901 w1917 w1936 w1960 w1966 w2041 w2056 w2075 w2077 w2148 w2227 w2236 w2256 w2263 w2320 w2352 w2367 w2371 w2395 w2428 w2454 w2474 w2515 w2539 w2549 w2561] -> w1417
                tunnel: [_ _ _ _ _ _ _ _ _ _ _ _ _ _ _ _ _ _ _ _ _ _ _ _ _ _ _ _ _ _ _ _ _ _ _ _ _ _ TRUE _ _ _ _ _ _ _ _ _] -> w1382
                tunnel: [_ _ _ _ _ _ _ _ _ _ _ _ _ _ _ _ _ _ _ _ w1845 w1872 _ _ _ _ _ _ _ _ _ _ _ _ _ _ _ _ _ _ _ _ _ _ _ _ _ _] -> w1412
                tunnel: [_ _ _ _ _ _ _ _ _ _ _ _ _ _ _ _ _ _ _ _ w1844 w1871 _ _ _ _ _ _ _ _ _ _ _ _ _ _ _ _ _ _ _ _ _ _ _ _ _ _] -> w1411
                tunnel: w1355 -> [w1433 w1438 w1480 w1510 w1545 w1581 w1608 w1635 w1651 w1678 w1687 w1695 w1711 w1722 w1731 w1747 w1761 w1781 w1791 w1814 w1848 w1875 w1899 w1914 w1935 w1939 w1988 w2040 w2055 w2073 w2095 w2166 w2225 w2235 w2255 w2272 w2318 w2349 w2364 w2373 w2380 w2407 w2452 w2472 w2509 w2537 w2547 w2559]
                tunnel: [w1433 w1438 w1480 w1510 w1545 w1580 w1603 w1621 w1645 w1674 w1686 w1694 w1710 w1721 w1730 w1746 w1761 w1781 w1790 w1813 w1847 w1874 w1899 w1914 w1935 w1938 w1962 w2040 w2055 w2073 w2092 w2163 w2225 w2235 w2254 w2272 w2318 w2349 w2364 w2373 w2380 w2407 w2452 w2472 w2509 w2537 w2547 w2559] -> w1414
                tunnel: w1413 -> [_ _ _ _ _ _ _ _ _ _ _ _ _ _ _ _ _ _ _ _ _ _ _ _ _ _ _ _ _ _ _ _ _ _ w2248 _ _ _ _ _ _ _ _ _ _ _ _ _]
                tunnel: w1410 -> [w1432 _ _ _ w1542 w1575 w1611 w1639 w1656 _ _ w1702 _ _ _ _ _ _ _ w1799 w1849 w1876 _ _ w1933 w1958 w1987 _ _ _ _ _ _ _ w2251 _ _ _ w2362 _ _ _ _ _ w2495 _ _ _]
                tunnel: w1409 -> [w1431 _ _ _ w1543 w1574 w1602 w1638 w1655 _ _ w1701 _ _ _ _ _ _ _ w1798 w1850 w1877 _ _ w1934 w1957 w1986 _ _ _ _ _ _ _ w2250 _ _ _ w2361 _ _ _ _ _ w2494 _ _ _]
                tunnel: [_ _ _ _ _ _ _ _ _ _ _ _ _ _ w1739 w1755 _ _ _ _ w1855 w1882 _ _ w1926 w1945 _ w2036 _ _ _ _ _ _ _ _ _ _ _ _ _ _ _ _ _ _ _ _] -> w1388
                tunnel: [_ _ _ _ _ _ _ _ _ _ _ _ _ _ w1738 w1754 _ _ _ _ w1854 w1881 _ _ w1925 w1944 _ w2037 _ _ _ _ _ _ _ _ _ _ _ _ _ _ _ _ _ _ _ _] -> w1369
                tunnel: [_ _ _ _ _ _ _ _ TRUE ("Recording") _ _ _ _ _ _ _ _ _ _ _ _ _ _ _ _ _ _ _ _ _ _ _ _ _ _ _ _ _ _ _ _ _ _ _ _ _ _ _] -> w1385
                tunnel: w1408 -> [_ _ _ _ _ _ _ _ _ _ _ _ _ _ _ _ _ _ _ _ _ _ _ _ _ _ _ _ _ _ _ _ _ _ _ _ _ _ _ _ w2392 w2423 w2450 w2457 _ _ _ _]
                tunnel: [_ _ _ _ _ _ _ _ _ _ _ _ _ _ _ _ _ _ _ _ _ _ _ _ _ _ _ _ _ _ _ _ _ _ _ _ _ _ _ _ w2390 w2422 w2448 w2458 _ _ _ _] -> w1407
                tunnel: w1406 -> [_ _ _ _ w1522 _ _ _ w1652 w1679 w1685 w1693 w1708 w1718 w1735 w1751 w1762 w1780 w1789 w1811 w1856 w1883 w1898 w1913 w1922 w1946 _ _ _ _ _ _ _ _ _ _ _ _ _ _ _ _ _ _ _ _ _ _]
                tunnel: [_ _ _ _ w1522 _ _ w1622 w1652 w1673 w1684 w1692 w1707 w1717 w1735 w1751 w1762 w1780 w1788 w1810 w1856 w1883 w1898 w1913 w1922 w1946 _ _ _ _ _ _ _ _ _ _ _ _ _ _ _ _ _ _ _ _ _ _] -> w1405
                tunnel: [_ _ _ _ _ _ _ _ _ _ _ _ _ _ w1737 w1753 _ _ _ _ w1853 w1880 _ _ w1924 w1943 _ w2038 _ _ _ _ _ _ _ _ _ _ _ _ _ _ _ _ _ _ _ _] -> w1392
                tunnel: [_ _ _ _ _ _ _ _ _ _ _ _ _ _ w1736 w1752 _ _ _ _ w1852 w1879 _ _ w1923 w1942 _ w2039 _ _ _ _ _ _ _ _ _ _ _ _ _ _ _ _ _ _ _ _] -> w1393
                tunnel: [_ _ _ _ _ _ _ _ _ _ _ _ _ _ _ _ _ _ _ _ w1846 w1873 _ _ _ _ _ _ _ _ _ _ _ _ _ _ _ _ _ _ _ _ _ _ _ _ _ _] -> w1395
                tunnel: [_ _ "<S,S>" ("string") _ _ _ _ _ w1646 _ _ _ _ _ _ _ _ _ _ _ _ _ _ _ _ _ w1961 _ _ _ w2084 w2155 _ _ w2246 _ _ w2344 _ _ _ _ _ _ _ _ _ _] -> w1358
                tunnel: w1357 -> [_ _ _ _ _ _ _ _ _ _ _ _ _ _ _ _ _ _ _ _ _ _ _ _ _ _ _ _ _ _ _ _ _ _ _ _ _ _ _ _ _ _ _ _ w2500 _ _ _]
                tunnel: w1353 -> [_ _ _ _ _ _ _ _ _ _ _ _ _ _ _ _ _ _ _ _ _ _ _ _ _ _ _ _ _ _ _ _ _ _ _ _ _ w2343 _ _ _ _ _ _ _ _ _ _]
                tunnel: w1352 -> [_ _ _ _ _ _ _ _ _ _ _ _ _ _ _ _ _ _ _ _ _ _ _ _ _ _ _ _ _ _ _ _ _ _ _ _ _ _ _ _ _ _ _ _ _ _ _ _]
                tunnel: w1351 -> [_ _ _ _ _ _ _ _ _ _ _ _ _ _ _ _ _ _ _ _ _ _ _ _ _ _ _ _ _ _ _ _ _ _ _ _ _ _ _ _ _ _ _ _ _ _ _ _]
                tunnel: [_ _ _ _ _ _ _ _ _ _ _ _ _ _ _ _ _ _ _ _ _ _ _ _ _ _ _ _ _ _ _ _ _ _ _ w2266 _ _ _ _ _ _ _ _ _ _ _ _] -> w1350
                tunnel: [_ _ _ _ _ _ _ _ _ _ _ _ _ _ _ _ _ _ _ _ _ _ _ _ _ _ _ _ _ _ _ _ _ _ _ w2271 _ _ _ _ _ _ _ _ _ _ _ _] -> w1349
                tunnel: w1348 -> [_ _ _ _ _ _ _ _ _ _ _ _ _ _ _ _ _ _ _ _ _ _ _ _ _ _ _ _ _ _ _ _ _ _ _ w2270 _ _ _ _ _ _ _ _ _ _ _ _]
                tunnel: w1347 -> [_ _ _ _ _ _ _ _ _ _ _ _ _ _ _ _ _ _ _ _ _ _ _ _ _ _ _ _ _ _ _ _ _ _ _ w2261 _ _ _ _ _ _ _ _ _ _ _ _]
                tunnel: w1340 -> [_ _ w1457 w1495 _ w1564 w1596 _ _ _ _ _ _ _ _ _ _ _ _ _ _ _ _ _ _ _ w1975 _ _ _ w2087 w2158 _ _ _ _ _ _ _ _ w2387 w2410 _ _ w2480 _ _ _]
                tunnel: w1339 -> [_ _ w1456 w1494 _ w1565 w1595 _ _ _ _ _ _ _ _ _ _ _ _ _ _ _ _ _ _ _ w1974 _ _ _ w2085 w2156 _ _ _ _ _ _ _ _ w2386 w2409 _ _ w2479 _ _ _]
                tunnel: w1338 -> [_ _ _ _ _ _ _ _ _ _ _ _ _ _ _ _ _ _ _ _ _ _ _ _ _ _ _ _ _ _ _ _ _ _ _ _ _ _ _ _ w2384 w2408 _ _ _ _ _ _]
                tunnel: w1334 -> [_ _ _ _ _ _ _ _ _ _ _ _ _ _ _ _ _ _ _ _ w1842 w1869 _ _ _ _ _ _ _ _ _ _ _ _ _ _ _ _ _ _ _ _ _ _ _ _ _ _]
                frame "Start1", Default {
                  w1430 = FALSE ("SelectionState")
                  n298 = xnode "Read/Write Control"("FPGA VI Reference In"=w1432, "error in"=w1431, "SelectionState"=w1430, "LR_reward_Laser_l1"=w1430, "LR_wrong_Laser_l1"=w1430, "LR_reward_Event_l1"=w1430, "LR_wrong_Event_l1"=w1430, "Left(F)_or_Right(T)"=w1430, "SelectionState"=w1430, "LR_reward_Laser_l2"=w1430, "LR_wrong_laser_l2"=w1430, "LR_reward_Event_l2"=w1430, "LR_wrong_Event_l2"=w1430, "LC_Event_l1"=w1430, "LC_Laser_l1"=w1430, "LC_Laser_l2"=w1430, "LC_Event_l2"=w1430, "CueLed_Event"=w1430) -> ("error out"=w1429:errorcluster)  [unwired: 1 out]
                  n299 = local write "error out"(w1429) -> ()
                }
                frame "Start2" {
                }
                frame "Start3" {
                  w1445 = u16 3 ("element")
                  w1443 = u16 0 ("element")
                  w1470 = u16 0 ("new element/subarray")
                  w1475 = 0.0 ("BTPR_avg_L")
                  w1478 = FALSE ("SolenoidReward")
                  w1476 = u16 0 ("BTPR_block")
                  w1479 = u16 0 ("nRewards_cur")
                  # "Goal:\nPrepare dataCurrent"
                  n300 = call "BRig_dataExp_FreeReward_c_L.vi"() -> ("output_FreeReward_c_L"=w1472:i32)  [unwired: 11 in]
                  n301 = call "BRig_dataExp_FreeReward_c_R.vi"() -> ("output_FreeReward_c_R"=w1471:i32)  [unwired: 11 in]
                  n302 = local write "nRewards_cur"(w1479) -> ()
                  n303 = local write "nRewards_total"(w1479) -> ()
                  n304 = local write "nRewards_Left"(w1479) -> ()
                  n305 = local write "nRewards_Right"(w1479) -> ()
                  n306 = local write "BUR_target"(w1479) -> ()
                  n307 = local write "TpB_target"(w1479) -> ()
                  n308 = local write "iBlock"(w1479) -> ()
                  n309 = local write "iTrial"(w1479) -> ()
                  n310 = local write "nTrial"(w1479) -> ()
                  n311 = local write "SolenoidReward"(w1478) -> ()
                  n312 = local write "allReward_L"(w1478) -> ()
                  n313 = local write "allReward_R"(w1478) -> ()
                  n314 = local write "BTPR_avg_L"(w1475) -> ()
                  n315 = local write "BTPR_avg_R"(w1475) -> ()
                  n316 = local write "T2R_avg_L"(w1475) -> ()
                  n317 = local write "T2R_avg_R"(w1475) -> ()
                  n318 = Replace Array Subset(array=w1474, new element #1=w1470, index #1=w1472, new element #2=w1470, index #2=w1471) -> (w1473:u16[])
                  n319 = call "BRig_dataRT_stats__T2R_cur.vi"() -> ("output_T2R_cur"=w1469:i32)  [unwired: 11 in]
                  n320 = call "BRig_dataRT_stats__BTPR_cur.vi"() -> ("output_BTPR_cur"=w1468:i32)  [unwired: 11 in]
                  n321 = call "BRig_dataRT_stats__T2R_avg_L.vi"() -> ("output_T2R_avg_L__x100"=w1463:i32)  [unwired: 11 in]
                  n322 = call "BRig_dataRT_stats__T2R_avg_R.vi"() -> ("output_T2R_avg_R__x100"=w1462:i32)  [unwired: 11 in]
                  n323 = call "BRig_dataRT_stats__BTPR_avg_L.vi"() -> ("output_BTPR_avg_L__x100"=w1467:i32)  [unwired: 11 in]
                  n324 = call "BRig_dataRT_stats__BTPR_avg_R.vi"() -> ("output_BTPR_avg_R__x100"=w1459:i32)  [unwired: 11 in]
                  n325 = call "BRig_dataRT_stats__nReward.vi"() -> ("output_nReward"=w1454:i32)  [unwired: 11 in]
                  n326 = call "BRig_dataRT_stats__nReward_left.vi"() -> ("output_nReward_left"=w1453:i32)  [unwired: 11 in]
                  n327 = call "BRig_dataRT_stats__nReward_right.vi"() -> ("output_nReward_right"=w1452:i32)  [unwired: 11 in]
                  n328 = local write "FreeReward_c_L"(w1470) -> ()
                  n329 = local write "FreeReward_c_R"(w1470) -> ()
                  n330 = local write "BTPR_block"(w1476) -> ()
                  n331 = local write "T2R_block"(w1476) -> ()
                  n332 = call "BRig_dataRT_stats__FreeReward_c_L.vi"() -> ("output_FreeReward_c_L"=w1448:i32)  [unwired: 11 in]
                  n333 = call "BRig_dataRT_stats__FreeReward_c_R.vi"() -> ("output_FreeReward_c_R"=w1447:i32)  [unwired: 11 in]
                  n334 = To Unsigned Word Integer(number=w1463) -> (unsigned 16bit integer=w1464:u16)
                  n335 = To Unsigned Word Integer(number=w1469) -> (unsigned 16bit integer=w1466:u16)
                  n336 = To Unsigned Word Integer(number=w1462) -> (unsigned 16bit integer=w1461:u16)
                  n337 = To Unsigned Word Integer(number=w1468) -> (unsigned 16bit integer=w1465:u16)
                  n338 = To Unsigned Word Integer(number=w1467) -> (unsigned 16bit integer=w1460:u16)
                  n339 = To Unsigned Word Integer(number=w1459) -> (unsigned 16bit integer=w1458:u16)
                  n340 = To Unsigned Word Integer(number=w1454) -> (unsigned 16bit integer=w1451:u16)
                  n341 = To Unsigned Word Integer(number=w1453) -> (unsigned 16bit integer=w1450:u16)
                  n342 = To Unsigned Word Integer(number=w1452) -> (unsigned 16bit integer=w1449:u16)
                  n343 = To Unsigned Word Integer(number=w1448) -> (unsigned 16bit integer=w1446:u16)
                  n344 = To Unsigned Word Integer(number=w1447) -> (unsigned 16bit integer=w1444:u16)
                  n345 = Build Array(w1445, w1466, w1443, w1445, w1465, w1443, w1445, w1464, w1443, w1445, w1461, w1443, w1445, w1460, w1443, w1445, w1458, w1443, w1445, w1451, w1443, w1445, w1450, w1443, w1445, w1449, w1443, w1445, w1446, w1443, w1445, w1444, w1443) -> (w1455:u16[])
                  n346 = RT FIFO Write(0:w1457, 1:w1455, 3:w1456) -> ()  [unwired: 2 in, 4 out]
                }
                frame "saveSettings1" {
                  w1497 = u16 3 ("element")
                  w1496 = u16 0 ("element")
                  n347 = call "BRig_dataRT_stats__nTrial.vi"() -> ("output_nTrial"=w1493:i32)  [unwired: 11 in]
                  n348 = call "BRig_dataRT_stats__iTrial.vi"() -> ("output_iTrial"=w1492:i32)  [unwired: 11 in]
                  n349 = call "BRig_dataRT_stats__iBlock.vi"() -> ("output_iBlock"=w1491:i32)  [unwired: 11 in]
                  n350 = call "BRig_dataRT_stats__nReward_cur.vi"() -> ("output_nReward_cur"=w1490:i32)  [unwired: 11 in]
                  n351 = call "BRig_dataRT_stats__TpB_target.vi"() -> ("output_TpB_target"=w1489:i32)  [unwired: 11 in]
                  n352 = call "BRig_dataRT_stats__BUR_target.vi"() -> ("output_BUR_target"=w1488:i32)  [unwired: 11 in]
                  n353 = call "BRig_dataRT_stats__DAB_nReward_HighProb.vi"() -> ("output_DAB_nReward_HighProb"=w1487:i32)  [unwired: 11 in]
                  n354 = call "BRig_dataRT_stats__DAB_nReward_LowProb.vi"() -> ("output_DAB_nReward_LowProb"=w1486:i32)  [unwired: 11 in]
                  n355 = call "BRig_dataRT_stats__DAB_nTimeout.vi"() -> ("output_DAB_nTimeout"=w1485:i32)  [unwired: 11 in]
                  n356 = To Unsigned Word Integer(number=w1491) -> (unsigned 16bit integer=w1505:u16)
                  n357 = To Unsigned Word Integer(number=w1493) -> (unsigned 16bit integer=w1507:u16)
                  n358 = To Unsigned Word Integer(number=w1490) -> (unsigned 16bit integer=w1504:u16)
                  n359 = To Unsigned Word Integer(number=w1492) -> (unsigned 16bit integer=w1506:u16)
                  n360 = To Unsigned Word Integer(number=w1489) -> (unsigned 16bit integer=w1503:u16)
                  n361 = To Unsigned Word Integer(number=w1488) -> (unsigned 16bit integer=w1502:u16)
                  n362 = To Unsigned Word Integer(number=w1487) -> (unsigned 16bit integer=w1500:u16)
                  n363 = To Unsigned Word Integer(number=w1486) -> (unsigned 16bit integer=w1499:u16)
                  n364 = To Unsigned Word Integer(number=w1485) -> (unsigned 16bit integer=w1498:u16)
                  n365 = Build Array(w1497, w1507, w1496, w1497, w1506, w1496, w1497, w1505, w1496, w1497, w1504, w1496, w1497, w1503, w1496, w1497, w1502, w1496, w1497, w1500, w1496, w1497, w1499, w1496, w1497, w1498, w1496) -> (w1501:u16[])
                  n366 = RT FIFO Write(0:w1495, 1:w1501, 3:w1494) -> ()  [unwired: 2 in, 4 out]
                }
                frame "setSettings_Laser" {
                  n367 = call "BRig_dataExp_LED_baseline_Cue.vi"() -> ("output_LED_baseline_Cue"=w1531:i32)  [unwired: 11 in]
                  n368 = call "BRig_dataExp_LED_baseline_l1.vi"() -> ("output_LED_baseline_l1"=w1532:i32)  [unwired: 11 in]
                  n369 = call "BRig_dataExp_LED_baseline_l2.vi"() -> ("output_LED_baseline_l2"=w1530:i32)  [unwired: 11 in]
                  n370 = call "BRig_dataExp_I_trialUntilReward.vi"() -> ("output_I_trialUntilReward"=w1517:i32)  [unwired: 11 in]
                  n371 = local read "FPGA_count2ms"() -> (w1540:dbl)
                  n372 = call "BRig_RT__Case_Exp__State_setLaserSettings__v2.vi"("input_FPGA_count2ms"=w1540, "input_dataExp"=w1515, "input_dataLC"=w1541) -> ("output_LR_nTotal_l1"=w1539:u32, "output_LR_nTotal_l2"=w1538:u32, "output_LR_reward_nDelay_l1"=w1537:u32, "output_LR_wrong_nDelay_l1"=w1536:u32, "output_LR_reward_nDelay_l2"=w1535:u32, "output_LR_wrong_nDelay_l2"=w1534:u32)  [unwired: 11 in]
                  n373 = Index Array(array=w1515, index #1=w1531, index #2=w1532, index #3=w1530, index #4=w1517) -> (element #1=w1529:u16, element #2=w1528:u16, element #3=w1527:u16, element #4=w1516:u16)  [unwired: 1 in, 1 out]
                  n374 = Not Equal To 0?(x=w1528) -> (x != 0?=w1525:bool)
                  n375 = Not Equal To 0?(x=w1529) -> (x != 0?=w1526:bool)
                  n376 = Not Equal To 0?(x=w1527) -> (x != 0?=w1524:bool)
                  n377 = Not Equal To 0?(x=w1516) -> (x != 0?=w1523:bool)
                  n378 = local read "LaserFiber_V_l1"() -> (w1521:dbl)
                  n379 = local read "LaserFiber_V_l2"() -> (w1519:dbl)
                  n380 = call "myRIO__convert__Voltage_to_FPGAvalue.vi"("input_voltage"=w1521) -> ("output_PortA"=w1520:u16)  [unwired: 9 in, 1 out]
                  n381 = call "myRIO__convert__Voltage_to_FPGAvalue.vi"("input_voltage"=w1519) -> ("output_PortA"=w1518:u16)  [unwired: 9 in, 1 out]
                  n382 = xnode "Read/Write Control"("FPGA VI Reference In"=w1542, "error in"=w1543, "LR_reward_nTotal_l1"=w1539, "LR_wrong_nTotal_l1"=w1539, "LR_reward_nTotal_l2"=w1538, "LR_wrong_nTotal_l2"=w1538, "LR_reward_nDelay_l1"=w1537, "LR_wrong_nDelay_l1"=w1536, "LR_reward_nDelay_l2"=w1535, "LR_wrong_nDelay_l2"=w1534, "CueLed_Baseline"=w1526, "L1Led_Baseline"=w1525, "L2Led_Baseline"=w1524, "ignoreWrong"=w1523, "AnaOut0_Pair"=w1520, "AnaOut1_Pair"=w1518) -> ("error out"=→"error out":errorcluster)  [unwired: 1 out]
                }
                frame "initBlock" {
                  w1547 = u16 0 ("element")
                  w1550 = u16 3
                  w1567 = u16 0 ("BTPR_block")
                  n383 = local write "nRewards_cur"(u16 0 ("nRewards_cur")) -> ()
                  n384 = local write "BTPR_block"(w1567) -> ()
                  n385 = local write "T2R_block"(w1567) -> ()
                  n386 = call "BRig_RT__Case_Exp__State_initBlock__v17.vi"("input_dataCurrent"=w1587, "input_dataExp"=w1586, "input_dataBlock"=w1583, "input_dataTrial"=w1581) -> ("output_iSpout"=w1572:u16, "output_speaker_amp_R"=w1576:u16, "output_iBlock"=w1556:u16, "output_speaker_freq_R"=w1577:u8, "output_BUR_target"=w1557:u16, "output_speaker_amp_L"=w1578:u16, "output_TpB_target"=w1558:u16, "output_speaker_freq_L"=w1579:u8, "output_dataCurrent"=w1585:u16[], "output_dataBlock"=w1582:u16[][], "output_dataTrial"=w1580:u16[][])  [unwired: 5 in]
                  n387 = Type Cast(type=enum16{"Left", "Right"}."Left", x=w1572) -> (*(type *) &x=w1569:enum16{"Left", "Right"})
                  n388 = Not Equal To 0?(x=w1572) -> (x != 0?=w1568:bool)
                  n389 = call "BRig_dataRT_stats__TpB_target.vi"() -> ("output_TpB_target"=w1559:i32)  [unwired: 11 in]
                  n390 = call "BRig_dataRT_stats__BUR_target.vi"() -> ("output_BUR_target"=w1560:i32)  [unwired: 11 in]
                  n391 = call "BRig_dataRT_stats__iBlock.vi"() -> ("output_iBlock"=w1561:i32)  [unwired: 11 in]
                  n392 = call "BRig_dataRT_stats__T2R_cur.vi"() -> ("output_T2R_cur"=w1554:i32)  [unwired: 11 in]
                  n393 = call "BRig_dataRT_stats__BTPR_cur.vi"() -> ("output_BTPR_cur"=w1553:i32)  [unwired: 11 in]
                  n394 = call "BRig_dataRT_stats__nReward_cur.vi"() -> ("output_nReward_cur"=w1549:i32)  [unwired: 11 in]
                  n395 = local write "cSpout"(w1569) -> ()
                  n396 = xnode "Read/Write Control"("FPGA VI Reference In"=w1575, "error in"=w1574, "Left(F)_or_Right(T)"=w1568, "audioFreq_L_kHz"=w1579, "audioAmp_L"=w1578, "audioFreq_R_kHz"=w1577, "audioAmp_R"=w1576) -> ("error out"=w1573:errorcluster)  [unwired: 1 out]
                  n397 = To Unsigned Word Integer(number=w1554) -> (unsigned 16bit integer=w1552:u16)
                  n398 = To Unsigned Word Integer(number=w1549) -> (unsigned 16bit integer=w1548:u16)
                  n399 = To Unsigned Word Integer(number=w1559) -> (unsigned 16bit integer=w1566:u16)
                  n400 = To Unsigned Word Integer(number=w1560) -> (unsigned 16bit integer=w1563:u16)
                  n401 = To Unsigned Word Integer(number=w1561) -> (unsigned 16bit integer=w1562:u16)
                  n402 = To Unsigned Word Integer(number=w1553) -> (unsigned 16bit integer=w1551:u16)
                  n403 = local write "error out"(w1573) -> ()
                  n404 = local write "iBlock"(w1556) -> ()
                  n405 = local write "BUR_target"(w1557) -> ()
                  n406 = local write "TpB_target"(w1558) -> ()
                  n407 = Build Array(w1550, w1566, w1558, w1550, w1563, w1557, w1550, w1562, w1556, w1550, w1552, w1547, w1550, w1551, w1547, w1550, w1548, w1547) -> (w1555:u16[])
                  n408 = RT FIFO Write(0:w1564, 1:w1555, 3:w1565) -> ()  [unwired: 2 in, 4 out]
                }
                frame "initTrial" {
                  w1592 = u16 3
                  n409 = xnode "Read/Write Control"("FPGA VI Reference In"=w1611, "error in"=w1602, "SelectionState"=FALSE) -> ("error out"=w1610:errorcluster)  [unwired: 1 out]
                  n410 = call "BRig_RT__Case_Exp__State_initTrial__v18.vi"("input_dataCurrent"=w1601, "input_dataBlock"=w1605, "input_dataTrial"=w1608, "input_dataExp"=w1589) -> ("output_iTrial"=w1590:u16, "output_nTrial"=w1591:u16, "output_SolenoidReward"=w1607:bool, "output_dataCurrent"=w1600:u16[], "output_dataBlock"=w1604:u16[][], "output_dataTrial"=w1603:u16[][])  [unwired: 6 in]
                  n411 = call "BRig_dataRT_stats__nTrial.vi"() -> ("output_nTrial"=w1594:i32)  [unwired: 11 in]
                  n412 = call "BRig_dataRT_stats__iTrial.vi"() -> ("output_iTrial"=w1593:i32)  [unwired: 11 in]
                  n413 = local write "iTrial"(w1590) -> ()
                  n414 = local write "nTrial"(w1591) -> ()
                  n415 = local write "SolenoidReward"(w1607) -> ()
                  n416 = To Unsigned Word Integer(number=w1594) -> (unsigned 16bit integer=w1599:u16)
                  n417 = To Unsigned Word Integer(number=w1593) -> (unsigned 16bit integer=w1597:u16)
                  n418 = local write "error out"(w1610) -> ()
                  n419 = Build Array(w1592, w1599, w1591, w1592, w1597, w1590) -> (w1598:u16[])
                  n420 = RT FIFO Write(0:w1596, 1:w1598, 3:w1595) -> ()  [unwired: 2 in, 4 out]
                }
                frame "initTrial2" {
                  n421 = call "BRig_RT__Case_Exp__State_initTrial2__v17.vi"("input_dataCurrent"=w1620, "input_dataTrial"=w1635, "input_dataExp"=w1619, "input_dataBlock"=w1633, "input_dataLC"=w1634) -> ("output_L_Wrong_Laser_l2"=w1625:bool, "output_L_Wrong_Event_l2"=w1626:bool, "output_L_Power_l1"=w1624:dbl, "output_L_Reward_Laser_l2"=w1627:bool, "output_L_Power_l2"=w1623:dbl, "output_L_Reward_Event_l2"=w1628:bool, "output_dataCurrent"=w1615:u16[], "output_dataTrial"=w1621:u16[][], "output_L_Reward_Event_l1"=w1632:bool, "output_L_Reward_Laser_l1"=w1631:bool, "output_L_Wrong_Event_l1"=w1630:bool, "output_L_Wrong_Laser_l1"=w1629:bool)  [unwired: 3 in]
                  n422 = local write "L_Power_l1"(w1624) -> ()
                  n423 = call "myRIO__convert__Voltage_to_FPGAvalue.vi"("input_voltage"=w1624) -> ("output_PortA"=w1613:u16)  [unwired: 9 in, 1 out]
                  n424 = local write "L_Power_l2"(w1623) -> ()
                  n425 = call "myRIO__convert__Voltage_to_FPGAvalue.vi"("input_voltage"=w1623) -> ("output_PortA"=w1614:u16)  [unwired: 9 in, 1 out]
                  n426 = xnode "Read/Write Control"("FPGA VI Reference In"=w1639, "error in"=w1638, "AnaOut_0"=w1613, "AnaOut_1"=w1614, "LR_reward_Event_l1"=w1632, "LR_reward_Laser_l1"=w1631, "LR_wrong_Event_l1"=w1630, "LR_wrong_Laser_l1"=w1629, "LR_reward_Event_l2"=w1628, "LR_reward_Laser_l2"=w1627, "LR_wrong_Event_l2"=w1626, "LR_wrong_laser_l2"=w1625) -> ("error out"=w1636:errorcluster)  [unwired: 1 out]
                  n427 = local write "error out"(w1636) -> ()
                  n428 = call "BRig_dataCurrent_DAB_flipLR.vi"() -> ("output_DAB_flipLR"=w1618:i32)  [unwired: 11 in]
                  n429 = call "BRig_arrTrig_init.vi"() -> ("output_arrTrig"=w1622:bool[])  [unwired: 11 in]
                  n430 = Index Array(array=w1615, index=w1618) -> (element=w1617:u16)
                  n431 = Not Equal To 0?(x=w1617) -> (x != 0?=w1616:bool)
                  n432 = local write "DAB_flipLR"(w1616) -> ()
                }
                frame "initTrial4" {
                  # "Dual Armed Bandit?"
                  # "resetOccurrence?\ndataAnalog"
                  n433 = local read "FPGA_count2ms"() -> (w1648:dbl)
                  n434 = local read "lick_Rising(F)_or_Falling(T)"() -> (w1644:bool)
                  n435 = call "BRig_dataExp_I_anySelect.vi"() -> ("output_I_anySelect"=w1643:i32)  [unwired: 11 in]
                  n436 = Index Array(array=w1641, index=w1643) -> (element=w1642:u16)
                  n437 = local read "Recording"() -> (w1650:bool)
                  n438 = call "BRig_RT_comm_tcp_write_RTwrite__RunState_Trial_start.vi"("input_dataCurrent"=w1647) -> ("output_strCmd"=w1646:string)  [unwired: 10 in]
                  n439 = Not Equal To 0?(x=w1642) -> (x != 0?=w1640:bool)
                  n440 = call "BRig_RT__Case_Exp__State_initTrial4.vi"("input_Recording"=w1650, "input_FPGA_count2ms"=w1648, "input_dataTrial"=w1651) -> ("output_Solenoid_nTotal"=w1649:u32, "output_dataTrial"=w1645:u16[][])  [unwired: 7 in]
                  n441 = case shown="False" w1640 {
                    tunnel: w1656 -> [w1665 w1670]
                    tunnel: w1655 -> [w1664 w1669]
                    tunnel: [w1663 w1668] -> w1654
                    tunnel: w1650 -> [w1662 w1667]
                    tunnel: w1649 -> [w1661 _]
                    tunnel: w1644 -> [w1660 w1666]
                    frame False {
                      n442 = xnode "Read/Write Control"("FPGA VI Reference In"=w1665, "error in"=w1664, "Solenoid_nTotal_L"=w1661, "Solenoid_nTotal_R"=w1661, "A6_Act"=w1662, "Rising(F)_or_Falling(T)"=w1660) -> ("error out"=w1663:errorcluster)  [unwired: 1 out]
                    }
                    frame True {
                      n443 = xnode "Read/Write Control"("FPGA VI Reference In"=w1670, "error in"=w1669, "A6_Act"=w1667, "Rising(F)_or_Falling(T)"=w1666) -> ("error out"=w1668:errorcluster)  [unwired: 1 out]
                    }
                  }
                  n444 = local write "error out"(w1654) -> ()
                }
                frame "initTrial_LC_ENL1" {
                  n445 = call "BRig_RT__Case_Exp__State_initTrial__LC_ENL__v18.vi"("input_arrTrig"=w1679, "input_dataTrial"=w1678, "input_dataExp"=w1671, "input_dataLC"=w1676, "input_dataCurrent"=w1672) -> ("output_dataTrial"=w1674:u16[][], "output_dataCurrent"=w1675:u16[], "output_arrTrig"=w1673:bool[])  [unwired: 4 in]
                }
                frame "initTrial_LC_Cue1" {
                  n446 = call "BRig_RT__Case_Exp__State_initTrial__LC_Cue__v18.vi"("input_arrTrig"=w1685, "input_dataTrial"=w1687, "input_dataExp"=w1681, "input_dataLC"=w1683, "input_dataCurrent"=w1682) -> ("output_dataTrial"=w1686:u16[][], "output_dataCurrent"=w1689:u16[], "output_arrTrig"=w1684:bool[])  [unwired: 4 in]
                }
                frame "initTrial_LC_Sel" {
                  n447 = call "BRig_RT__Case_Exp__State_initTrial__LC_Select__v18.vi"("input_arrTrig"=w1693, "input_dataTrial"=w1695, "input_dataExp"=w1691, "input_dataLC"=w1697, "input_dataCurrent"=w1699) -> ("output_dataTrial"=w1694:u16[][], "output_dataCurrent"=w1698:u16[], "output_arrTrig"=w1692:bool[])  [unwired: 4 in]
                  n448 = xnode "Read/Write Control"("FPGA VI Reference In"=w1702, "error in"=w1701, "A6_Act"=FALSE) -> ("error out"=w1703:errorcluster)  [unwired: 1 out]
                  n449 = local write "error out"(w1703) -> ()
                }
                frame "ENL1_pre" {
                  n450 = call "BRig_RT__Case_Exp__State_ENLPre__v4.vi"("input_arrTrig"=w1708, "input_ENL2"=FALSE, "input_I_lick"=w1714, "input_dataExp"=w1706, "input_dataTrial"=w1711, "input_dataCurrent"=w1712) -> ("output_arrTrig"=w1707:bool[], "output_dataTrial"=w1710:u16[][], "output_dataCurrent"=w1705:u16[], "output_state"=w1713:T2)  [unwired: 2 in]
                }
                frame "ENL2_pre" {
                  n451 = call "BRig_RT__Case_Exp__State_ENLPre__v4.vi"("input_arrTrig"=w1718, "input_ENL2"=TRUE, "input_I_lick"=w1725, "input_dataExp"=w1719, "input_dataTrial"=w1722, "input_dataCurrent"=w1723) -> ("output_arrTrig"=w1717:bool[], "output_dataTrial"=w1721:u16[][], "output_dataCurrent"=w1726:u16[], "output_state"=w1724:T2)  [unwired: 2 in]
                }
                frame "ENL1" {
                  n452 = call "BRig_RT__Case_Exp__State_ENL__v3.vi"("input_dataCurrent"=w1741, "input_dataTrial"=w1731, "input_ENL2"=FALSE, "input_arrTrig"=w1735, "input_state"=w1734, "I_lick"=w1733) -> ("output_l2_laserOn"=w1736:bool, "output_l2_laserEvent"=w1737:bool, "output_l1_laserOn"=w1738:bool, "output_state"=w1732:T2, "output_l1_laserEvent"=w1739:bool, "output_dataCurrent"=w1740:u16[], "output_dataTrial"=w1730:u16[][])  [unwired: 7 in]
                }
                frame "ENL2" {
                  n453 = call "BRig_RT__Case_Exp__State_ENL__v3.vi"("input_dataCurrent"=w1757, "input_dataTrial"=w1747, "input_ENL2"=TRUE, "input_arrTrig"=w1751, "input_state"=w1750, "I_lick"=w1749) -> ("output_l2_laserOn"=w1752:bool, "output_l2_laserEvent"=w1753:bool, "output_l1_laserOn"=w1754:bool, "output_state"=w1748:T2, "output_l1_laserEvent"=w1755:bool, "output_dataCurrent"=w1756:u16[], "output_dataTrial"=w1746:u16[][])  [unwired: 7 in]
                }
                frame "ENL1Penalty_pre" {
                  n454 = call "BRig_dataCurrent_c_generic.vi"() -> ("output_count_generic"=w1773:i32)  [unwired: 11 in]
                  n455 = call "BRig_dataCurrent_T_generic.vi"() -> ("output_T_generic"=w1771:i32)  [unwired: 11 in]
                  n456 = call "BRig_dataExp_T_ENLPenalty.vi"() -> ("output_ENL_penalty"=w1766:i32)  [unwired: 11 in]
                  n457 = Index Array(array=w1767, index=w1766) -> (element=w1770:u16)
                  n458 = Replace Array Subset(array=w1768, new element #1=u16 0 ("new element/subarray"), index #1=w1773, new element #2=w1770, index #2=w1771) -> (w1769:u16[])
                }
                frame "ENL1Penalty" {
                  n459 = call "BRig_RT__Case_Exp__generic__incrementCountTilThreshold.vi"("input_dataCurrent"=w1776) -> ("output_dataCurrent"=w1775:u16[], "output_underThreshold"=w1774:bool)  [unwired: 9 in]
                  n460 = Select(t=w1779, s=w1774, f=myRIO_BRig_RT__Case_Exp_stateList."ENL1_pre" ("Enum")) -> (s? t:f=w1777:T2)
                }
                frame "Cue1_pre" {
                  n461 = call "BRig_RT__Case_Exp__State_CuePre__v5.vi"("input_dataCurrent"=w1794, "input_dataTrial"=w1791, "input_dataExp"=w1785, "input_Cue2"=FALSE ("input_ENL2"), "input_I_lick"=w1793, "input_arrTrig"=w1789) -> ("output_state"=w1792:T2, "output_arrTrig"=w1788:bool[], "output_dataCurrent"=w1786:u16[], "output_dataTrial"=w1790:u16[][])  [unwired: 10 in]
                }
                frame "Cue2_pre" {
                  # "Two cues?"
                  n462 = call "BRig_dataExp_I_Cue2.vi"() -> ("output_I_Cue2"=w1808:i32)  [unwired: 11 in]
                  n463 = call "BRig_dataExp_Audio_pattern_R.vi"() -> ("output_Audio_sp__R"=w1805:i32)  [unwired: 11 in]
                  n464 = call "BRig_dataExp_Audio_amp_R.vi"() -> ("output_Audio_amp__R"=w1804:i32)  [unwired: 11 in]
                  n465 = call "BRig_dataExp_Audio_freq_R.vi"() -> ("output_Audio_freq__R"=w1803:i32)  [unwired: 11 in]
                  n466 = Index Array(array=w1797, index #1=w1808, index #2=w1805, index #3=w1804, index #4=w1803) -> (element #1=w1807:u16, element #2=w1800:u16, element #3=w1801:u16, element #4=w1802:u16)
                  n467 = call "BRig_RT__Case_Exp__State_CuePre__v5.vi"("input_dataCurrent"=w1817, "input_dataTrial"=w1814, "input_dataExp"=w1797, "input_Cue2"=TRUE ("input_ENL2"), "input_I_lick"=w1816, "input_arrTrig"=w1811) -> ("output_state"=w1815:T2, "output_arrTrig"=w1810:bool[], "output_dataCurrent"=w1812:u16[], "output_dataTrial"=w1813:u16[][])  [unwired: 10 in]
                  n468 = Not Equal To 0?(x=w1807) -> (x != 0?=w1806:bool)
                  n469 = case shown="True" w1806 {
                    tunnel: w1802 -> [_ w1829]
                    tunnel: w1801 -> [_ w1828]
                    tunnel: w1800 -> [_ w1827]
                    tunnel: w1799 -> [_ w1826]
                    tunnel: w1798 -> [_ w1825]
                    frame False {
                    }
                    frame True {
                      n470 = To Unsigned Byte Integer(number=w1829) -> (unsigned 8bit integer=w1830:u8)
                      n471 = case shown="0, Default" w1827 {
                        tunnel: w1828 -> [w1834 w1837 w1839]
                        tunnel: w1830 -> [w1833 w1838 w1840]
                        tunnel: [w1834 u16 0 ("Numeric") w1839] -> w1824
                        tunnel: [w1833 u8 0 w1840] -> w1823
                        tunnel: [u8 0 w1838 w1840] -> w1821
                        tunnel: [u16 0 ("Numeric") w1837 w1839] -> w1822
                        frame 0, Default {
                          # "left only"
                        }
                        frame 1 {
                          # "right only"
                        }
                        frame 2 {
                          # "left and right"
                        }
                      }
                      n472 = xnode "Read/Write Control"("FPGA VI Reference In"=w1826, "error in"=w1825, "audioFreq_L_kHz"=w1823, "audioAmp_L"=w1824, "audioFreq_R_kHz"=w1821, "audioAmp_R"=w1822) -> ("error out"=w1820:errorcluster)  [unwired: 1 out]
                      n473 = local write "error out"(w1820) -> ()
                    }
                  }
                }
                frame "Cue1" {
                  n474 = call "BRig_RT__Case_Exp__State_Cue__v3.vi"("input_dataCurrent"=w1860, "input_dataTrial"=w1848, "input_dataExp"=w1842, "input_Cue2"=FALSE, "input_arrTrig"=w1856, "input_state"=w1858, "I_lick"=w1859) -> ("output_l2_laserOn"=w1852:bool, "output_l2_laserEvent"=w1853:bool, "output_SelectionState"=w1851:bool, "output_l1_laserOn"=w1854:bool, "output_state"=w1857:T2, "output_l1_laserEvent"=w1855:bool, "output_dataCurrent"=w1843:u16[], "output_dataTrial"=w1847:u16[][], "output_CueLed"=w1846:bool, "output_Audio_L"=w1845:bool, "output_Audio_R"=w1844:bool)  [unwired: 2 in]
                  n475 = case shown="True" w1851 {
                    selector: w1851 -> [_ w1866]
                    tunnel: w1850 -> [_ w1865]
                    tunnel: w1849 -> [_ w1864]
                    frame False {
                    }
                    frame True {
                      n476 = xnode "Read/Write Control"("FPGA VI Reference In"=w1864, "error in"=w1865, "SelectionState"=w1866) -> ("error out"=w1867:errorcluster)  [unwired: 1 out]
                      n477 = local write "error out"(w1867) -> ()
                    }
                  }
                }
                frame "Cue2" {
                  n478 = call "BRig_RT__Case_Exp__State_Cue__v3.vi"("input_dataCurrent"=w1887, "input_dataTrial"=w1875, "input_dataExp"=w1869, "input_Cue2"=TRUE, "input_arrTrig"=w1883, "input_state"=w1885, "I_lick"=w1886) -> ("output_l2_laserOn"=w1879:bool, "output_l2_laserEvent"=w1880:bool, "output_SelectionState"=w1878:bool, "output_l1_laserOn"=w1881:bool, "output_state"=w1884:T2, "output_l1_laserEvent"=w1882:bool, "output_dataCurrent"=w1870:u16[], "output_dataTrial"=w1874:u16[][], "output_CueLed"=w1873:bool, "output_Audio_L"=w1872:bool, "output_Audio_R"=w1871:bool)  [unwired: 2 in]
                  n479 = case shown="True" w1878 {
                    selector: w1878 -> [_ w1893]
                    tunnel: w1877 -> [_ w1892]
                    tunnel: w1876 -> [_ w1891]
                    frame False {
                    }
                    frame True {
                      n480 = xnode "Read/Write Control"("FPGA VI Reference In"=w1891, "error in"=w1892, "SelectionState"=w1893) -> ("error out"=w1894:errorcluster)  [unwired: 1 out]
                      n481 = local write "error out"(w1894) -> ()
                    }
                  }
                }
                frame "Cue1Penalty_pre" {
                  n482 = call "BRig_dataCurrent_c_generic.vi"() -> ("output_count_generic"=w1907:i32)  [unwired: 11 in]
                  n483 = call "BRig_dataCurrent_T_generic.vi"() -> ("output_T_generic"=w1905:i32)  [unwired: 11 in]
                  n484 = call "BRig_dataExp_T_CuePenalty.vi"() -> ("output_T_CuePenalty"=w1896:i32)  [unwired: 11 in]
                  n485 = Index Array(array=w1897, index=w1896) -> (element=w1895:u16)
                  n486 = Replace Array Subset(array=w1904, new element #1=u16 0 ("new element/subarray"), index #1=w1907, new element #2=w1895, index #2=w1905) -> (w1903:u16[])
                }
                frame "Cue1Penalty" {
                  n487 = call "BRig_RT__Case_Exp__generic__incrementCountTilThreshold.vi"("input_dataCurrent"=w1910) -> ("output_dataCurrent"=w1909:u16[], "output_underThreshold"=w1908:bool)  [unwired: 9 in]
                  n488 = Select(t=w1911, s=w1908, f=myRIO_BRig_RT__Case_Exp_stateList."ENL1_pre" ("Enum")) -> (s? t:f=w1912:T2)
                }
                frame "Selection_pre" {
                  n489 = xnode "Read/Write Control"("FPGA VI Reference In"=w1933, "error in"=w1934) -> ("error out"=w1932:errorcluster, "SelectReward"=w1929:bool, "SelectWrong"=w1930:bool)  [unwired: 1 out]
                  n490 = call "BRig_RT__Case_Exp__State_SelectPre__v2.vi"("input_dataCurrent"=w1931, "input_SelectWrong"=w1930, "input_SelectReward"=w1929, "input_dataExp"=w1919, "input_LickL"=w1921, "input_LickR"=w1920, "input_arrTrig"=w1922) -> ("output_state"=w1928:T2, "output_dataCurrent"=w1927:u16[], "output_l1_laserEvent"=w1926:bool, "output_l1_laserOn"=w1925:bool, "output_l2_laserOn"=w1923:bool, "output_l2_laserEvent"=w1924:bool)  [unwired: 3 in]
                  n491 = local write "error out"(w1932) -> ()
                }
                frame "Selection" {
                  n492 = xnode "Read/Write Control"("FPGA VI Reference In"=w1958, "error in"=w1957) -> ("error out"=w1956:errorcluster, "SelectReward"=w1953:bool, "SelectWrong"=w1954:bool)  [unwired: 1 out]
                  n493 = call "BRig_RT__Case_Exp__State_Selection__v2.vi"("input_state"=w1955, "input_dataCurrent"=w1948, "input_dataTrial"=w1939, "input_dataExp"=w1947, "input_arrTrig"=w1946, "input_SelectWrong"=w1954, "input_SelectReward"=w1953, "input_LickR"=w1952, "input_LickL"=w1951) -> ("output_l2_laserOn"=w1942:bool, "output_l2_laserEvent"=w1943:bool, "output_l1_laserOn"=w1944:bool, "output_l1_laserEvent"=w1945:bool, "output_state"=w1950:T2, "output_dataCurrent"=w1949:u16[], "output_dataTrial"=w1938:u16[][], "output_allReward_L"=w1940:bool, "output_allReward_R"=w1941:bool)  [unwired: 2 in]
                  n494 = local write "allReward_L"(w1940) -> ()
                  n495 = local write "allReward_R"(w1941) -> ()
                  n496 = local write "error out"(w1956) -> ()
                }
                frame "SelectReward_pre" {
                  # "Dual Armed\nBandit?"
                  n497 = call "BRig_dataExp_I_anySelect.vi"() -> ("output_I_anySelect"=w1979:i32)  [unwired: 11 in]
                  n498 = Index Array(array=w1977, index=w1979) -> (element=w1978:u16)
                  n499 = call "BRig_RT__Case_Exp__State_RewardPre__v11.vi"("input_dataCurrent"=w1991, "input_dataExp"=w1977, "input_dataBlock"=w1990, "input_dataTrial"=w1988, "input_dataLC"=w1966) -> ("output_T_Reward"=w1985:u16, "output_c_nReward_total_R"=w1970:u16, "output_c_nReward_total_L"=w1969:u16, "output_dataCurrent"=w1964:u16[], "output_DAB_L=L"=w1967:bool, "output_DAB_R=HighPorb"=w1968:bool, "output_dataBlock"=w1989:u16[][], "output_c_nReward_total"=w1972:u16, "output_nReward"=w1971:u16, "output_dataTrial"=w1962:u16[][])  [unwired: 1 in]
                  n500 = local read "FPGA_count2ms"() -> (w1984:dbl)
                  n501 = Not Equal To 0?(x=w1978) -> (x != 0?=w1976:bool)
                  n502 = case shown="True" w1976 {
                    tunnel: [w1998 w2028] -> w1973
                    tunnel: w1972 -> [w1997 w2025]
                    tunnel: w1971 -> [w1996 w2024]
                    tunnel: w1970 -> [w1995 w2027]
                    tunnel: w1969 -> [w1994 w2026]
                    tunnel: w1968 -> [_ w2018]
                    tunnel: w1967 -> [_ w2019]
                    tunnel: w1964 -> [w1993 w2013]
                    tunnel: [w1993 w2011] -> w1963
                    frame False {
                      w2002 = u16 3
                      n503 = call "BRig_dataRT_stats__nReward_left.vi"() -> ("output_nReward_left"=w1999:i32)  [unwired: 11 in]
                      n504 = call "BRig_dataRT_stats__nReward_right.vi"() -> ("output_nReward_right"=w2000:i32)  [unwired: 11 in]
                      n505 = call "BRig_dataRT_stats__nReward_cur.vi"() -> ("output_nReward_cur"=w2001:i32)  [unwired: 11 in]
                      n506 = call "BRig_dataRT_stats__nReward.vi"() -> ("output_nReward"=w2004:i32)  [unwired: 11 in]
                      n507 = To Unsigned Word Integer(number=w1999) -> (unsigned 16bit integer=w2007:u16)
                      n508 = To Unsigned Word Integer(number=w2000) -> (unsigned 16bit integer=w2006:u16)
                      n509 = To Unsigned Word Integer(number=w2001) -> (unsigned 16bit integer=w2005:u16)
                      n510 = To Unsigned Word Integer(number=w2004) -> (unsigned 16bit integer=w2003:u16)
                      n511 = local write "nRewards_Right"(w1995) -> ()
                      n512 = local write "nRewards_Left"(w1994) -> ()
                      n513 = local write "nRewards_cur"(w1996) -> ()
                      n514 = local write "nRewards_total"(w1997) -> ()
                      n515 = Build Array(w2002, w2007, w1994, w2002, w2006, w1995, w2002, w2005, w1996, w2002, w2003, w1997) -> (w1998:u16[])
                    }
                    frame True {
                      w2030 = u16 3
                      n516 = call "BRig_dataRT_stats__nReward_left.vi"() -> ("output_nReward_left"=w2023:i32)  [unwired: 11 in]
                      n517 = call "BRig_dataRT_stats__nReward_right.vi"() -> ("output_nReward_right"=w2022:i32)  [unwired: 11 in]
                      n518 = call "BRig_dataRT_stats__DAB_nReward_HighProb.vi"() -> ("output_DAB_nReward_HighProb"=w2021:i32)  [unwired: 11 in]
                      n519 = call "BRig_dataRT_stats__DAB_nReward_LowProb.vi"() -> ("output_DAB_nReward_LowProb"=w2020:i32)  [unwired: 11 in]
                      n520 = call "BRig_dataRT_stats__nReward_cur.vi"() -> ("output_nReward_cur"=w2029:i32)  [unwired: 11 in]
                      n521 = call "BRig_dataRT_stats__nReward.vi"() -> ("output_nReward"=w2032:i32)  [unwired: 11 in]
                      n522 = Select(t=w2023, s=w2019, f=w2022) -> (s? t:f=w2016:i32)
                      n523 = Select(t=w2021, s=w2018, f=w2020) -> (s? t:f=w2017:i32)
                      n524 = To Unsigned Word Integer(number=w2016) -> (unsigned 16bit integer=w2035:u16)
                      n525 = To Unsigned Word Integer(number=w2017) -> (unsigned 16bit integer=w2034:u16)
                      n526 = To Unsigned Word Integer(number=w2029) -> (unsigned 16bit integer=w2033:u16)
                      n527 = To Unsigned Word Integer(number=w2032) -> (unsigned 16bit integer=w2031:u16)
                      n528 = local write "nRewards_cur"(w2024) -> ()
                      n529 = local write "nRewards_total"(w2025) -> ()
                      n530 = call "BRig_dataCurrent_s_Selection.vi"() -> ("output_s_Selection"=w2012:i32)  [unwired: 11 in]
                      n531 = call "BRig_dataCurrent_I_giveReward.vi"() -> ("output_I_giveReward"=w2015:i32)  [unwired: 11 in]
                      n532 = Build Array(w2030, w2035, w2026, w2030, w2034, w2027, w2030, w2033, w2024, w2030, w2031, w2025) -> (w2028:u16[])
                      n533 = Index Array(array=w2013, index=w2015) -> (element=w2009:u16)
                      n534 = Not Equal To 0?(x=w2009) -> (x != 0?=w2014:bool)
                      n535 = local write "SolenoidReward"(w2014) -> ()
                      n536 = Subtract(x=u16 2 ("new element/subarray"), y=w2009) -> (x-y=w2008:u16)
                      n537 = Replace Array Subset(array=w2013, new element=w2008, index=w2012) -> (w2011:u16[])
                    }
                  }
                  n538 = To Double Precision Float(number=w1985) -> (double precision float=w1983:dbl)
                  n539 = Multiply(x=w1984, y=w1983) -> (x*y=w1981:dbl)
                  n540 = Round Toward +Infinity(x=w1981) -> (ceil(x): smallest int >= x=w1982:dbl)
                  n541 = To Unsigned Long Integer(number=w1982) -> (unsigned 32bit integer=w1980:u32)
                  n542 = RT FIFO Write(0:w1975, 1:w1973, 3:w1974) -> ()  [unwired: 2 in, 4 out]
                  n543 = xnode "Read/Write Control"("FPGA VI Reference In"=w1987, "error in"=w1986, "Solenoid_nTotal_L"=w1980, "Solenoid_nTotal_R"=w1980) -> ()  [unwired: 2 out]
                  n544 = call "BRig_RT_comm_tcp_write_RTwrite__RunState_Trial_selResult__v3.vi"("input_dataTrial"=w1962, "iReward_or_iError"=TRUE, "input_dataCurrent"=w1963) -> ("output_strCmd"=w1961:string)  [unwired: 8 in]
                }
                frame "SelectReward" {
                  n545 = call "BRig_dataCurrent_c_generic.vi"() -> ("output_count_generic"=w2048:i32)  [unwired: 11 in]
                  n546 = Index Array(array=w2049, index=w2048) -> (element=w2047:u16)
                  n547 = call "BRig_RT__Case_Exp__State_Reward.vi"("input_dataCurrent"=w2049, "input_state"=w2052, "input_dataTrial"=w2040, "input_dataLC"=w2041, "input_dataExp"=w2050) -> ("output_state"=w2051:T2, "output_dataCurrent"=w2053:u16[], "output_L_event_l1"=w2036:bool, "output_L_trig_l1"=w2037:bool, "output__L"=w2046:bool, "output_L_trig_l2"=w2039:bool, "output_L_event_l2"=w2038:bool, "output__R"=w2045:bool)  [unwired: 3 in]
                  n548 = Equal To 0?(x=w2047) -> (x = 0?=w2044:bool)
                  n549 = And(x=w2046, y=w2044) -> (x .and. y?=w2043:bool)
                  n550 = And(x=w2045, y=w2044) -> (x .and. y?=w2042:bool)
                }
                frame "SelectRewardPost_pre" {
                  n551 = call "BRig_dataExp_T_RewardPost.vi"() -> ("output_T_RewardPost"=w2058:i32)  [unwired: 11 in]
                  n552 = call "BRig_dataCurrent_c_generic.vi"() -> ("output_count_generic"=w2064:i32)  [unwired: 11 in]
                  n553 = call "BRig_dataCurrent_T_generic.vi"() -> ("output_T_generic"=w2063:i32)  [unwired: 11 in]
                  n554 = Index Array(array=w2059, index=w2058) -> (element=w2057:u16)
                  n555 = Replace Array Subset(array=w2061, new element #1=u16 0 ("new element/subarray"), index #1=w2064, new element #2=w2057, index #2=w2063) -> (w2060:u16[])
                }
                frame "SelectRewardPost" {
                  n556 = call "BRig_RT__Case_Exp__generic__incrementCountTilThreshold.vi"("input_dataCurrent"=w2069) -> ("output_dataCurrent"=w2067:u16[], "output_underThreshold"=w2068:bool)  [unwired: 9 in]
                  n557 = Select(t=w2071, s=w2068, f=myRIO_BRig_RT__Case_Exp_stateList."endTrial1" ("Enum")) -> (s? t:f=w2070:T2)
                }
                frame "SelectWrong_pre" {
                  # "Dual Armed\nBandit?"
                  n558 = call "BRig_dataExp_I_anySelect.vi"() -> ("output_I_anySelect"=w2081:i32)  [unwired: 11 in]
                  n559 = Index Array(array=w2082, index=w2081) -> (element=w2083:u16)
                  n560 = call "BRig_RT__Case_Exp__State_WrongOrTimeout_Pre__v11.vi"("input_dataCurrent"=w2099, "input_WorTO"=FALSE, "input_dataLC"=w2077, "input_dataBlock"=w2097, "input_dataTrial"=w2095, "input_dataExp"=w2082) -> ("output_T2R"=w2078:bool, "output_T2R_or_BTPR"=w2079:u16, "output_dataCurrent"=w2093:u16[], "output_dataBlock"=w2096:u16[][], "output_dataTrial"=w2092:u16[][], "output_BTPRavg"=w2088:dbl, "output_T2Ravg"=w2089:dbl, "output_R(F)_or_L(T)"=w2090:bool, "output_haveNewAvg"=w2091:bool)  [unwired: 1 out]
                  n561 = Not Equal To 0?(x=w2083) -> (x != 0?=w2080:bool)
                  n562 = case shown="False" w2080 {
                    tunnel: w2091 -> [_ w2115]
                    tunnel: w2090 -> [_ w2114]
                    tunnel: w2089 -> [_ w2113]
                    tunnel: w2088 -> [_ w2112]
                    tunnel: [w2104 w2110] -> w2086
                    tunnel: w2079 -> [w2102 w2106]
                    tunnel: w2078 -> [_ w2108]
                    frame True {
                      n563 = call "BRig_dataRT_stats__DAB_nTimeout.vi"() -> ("output_DAB_nTimeout"=w2101:i32)  [unwired: 11 in]
                      n564 = To Unsigned Word Integer(number=w2101) -> (unsigned 16bit integer=w2103:u16)
                      n565 = Build Array(u16 3, w2103, w2102) -> (w2104:u16[])
                    }
                    frame False {
                      n566 = case shown="False" w2108 {
                        tunnel: w2106 -> [w2117 w2119]
                        tunnel: [w2116 w2118] -> w2109
                        frame False {
                          n567 = call "BRig_dataRT_stats__BTPR_cur.vi"() -> ("output_BTPR_cur"=w2116:i32)  [unwired: 11 in]
                          n568 = local write "BTPR_block"(w2117) -> ()
                        }
                        frame True {
                          n569 = call "BRig_dataRT_stats__T2R_cur.vi"() -> ("output_T2R_cur"=w2118:i32)  [unwired: 11 in]
                          n570 = local write "T2R_block"(w2119) -> ()
                        }
                      }
                      n571 = To Unsigned Word Integer(number=w2109) -> (unsigned 16bit integer=w2107:u16)
                      n572 = case shown="True" w2115 {
                        tunnel: w2114 -> [_ w2139]
                        tunnel: w2113 -> [_ w2129]
                        tunnel: w2112 -> [_ w2125]
                        tunnel: u16 3 -> [w2123 w2132]
                        tunnel: w2107 -> [w2122 w2128]
                        tunnel: w2106 -> [w2121 w2131]
                        tunnel: [w2120 w2130] -> w2110
                        frame False {
                          n573 = Build Array(w2123, w2122, w2121) -> (w2120:u16[])
                        }
                        frame True {
                          w2124 = 100.0 ("y")
                          n574 = case shown="False" w2139 {
                            tunnel: w2129 -> [w2142 w2147]
                            tunnel: w2125 -> [w2143 w2146]
                            tunnel: [w2140 w2145] -> w2138
                            tunnel: [w2141 w2144] -> w2137
                            frame False {
                              n575 = local write "BTPR_avg_R"(w2143) -> ()
                              n576 = call "BRig_dataRT_stats__BTPR_avg_R.vi"() -> ("output_BTPR_avg_R__x100"=w2141:i32)  [unwired: 11 in]
                              n577 = local write "T2R_avg_R"(w2142) -> ()
                              n578 = call "BRig_dataRT_stats__T2R_avg_R.vi"() -> ("output_T2R_avg_R__x100"=w2140:i32)  [unwired: 11 in]
                            }
                            frame True {
                              n579 = call "BRig_dataRT_stats__BTPR_avg_L.vi"() -> ("output_BTPR_avg_L__x100"=w2144:i32)  [unwired: 11 in]
                              n580 = local write "BTPR_avg_L"(w2146) -> ()
                              n581 = local write "T2R_avg_L"(w2147) -> ()
                              n582 = call "BRig_dataRT_stats__T2R_avg_L.vi"() -> ("output_T2R_avg_L__x100"=w2145:i32)  [unwired: 11 in]
                            }
                          }
                          n583 = Multiply(x=w2129, y=w2124) -> (x*y=w2126:dbl)
                          n584 = Multiply(x=w2125, y=w2124) -> (x*y=w2127:dbl)
                          n585 = To Unsigned Word Integer(number=w2126) -> (unsigned 16bit integer=w2133:u16)
                          n586 = To Unsigned Word Integer(number=w2127) -> (unsigned 16bit integer=w2134:u16)
                          n587 = To Unsigned Word Integer(number=w2137) -> (unsigned 16bit integer=w2135:u16)
                          n588 = To Unsigned Word Integer(number=w2138) -> (unsigned 16bit integer=w2136:u16)
                          n589 = Build Array(w2132, w2136, w2133, w2132, w2135, w2134, w2132, w2128, w2131) -> (w2130:u16[])
                        }
                      }
                    }
                  }
                  n590 = RT FIFO Write(0:w2087, 1:w2086, 3:w2085) -> ()  [unwired: 2 in, 4 out]
                  n591 = call "BRig_RT_comm_tcp_write_RTwrite__RunState_Trial_selResult__v3.vi"("input_dataTrial"=w2092, "iReward_or_iError"=FALSE, "input_dataCurrent"=w2093) -> ("output_strCmd"=w2084:string)  [unwired: 8 in]
                }
                frame "SelectTimeout_pre" {
                  # "Dual Armed\nBandit?"
                  n592 = call "BRig_dataExp_I_anySelect.vi"() -> ("output_I_anySelect"=w2152:i32)  [unwired: 11 in]
                  n593 = Index Array(array=w2153, index=w2152) -> (element=w2154:u16)
                  n594 = call "BRig_RT__Case_Exp__State_WrongOrTimeout_Pre__v11.vi"("input_dataCurrent"=w2170, "input_WorTO"=TRUE, "input_dataLC"=w2148, "input_dataBlock"=w2168, "input_dataTrial"=w2166, "input_dataExp"=w2153) -> ("output_T2R"=w2149:bool, "output_T2R_or_BTPR"=w2150:u16, "output_dataCurrent"=w2164:u16[], "output_dataBlock"=w2167:u16[][], "output_dataTrial"=w2163:u16[][], "output_BTPRavg"=w2159:dbl, "output_T2Ravg"=w2160:dbl, "output_R(F)_or_L(T)"=w2161:bool, "output_haveNewAvg"=w2162:bool)  [unwired: 1 out]
                  n595 = Not Equal To 0?(x=w2154) -> (x != 0?=w2151:bool)
                  n596 = case shown="False" w2151 {
                    tunnel: w2162 -> [_ w2186]
                    tunnel: w2161 -> [_ w2185]
                    tunnel: w2160 -> [_ w2184]
                    tunnel: w2159 -> [_ w2183]
                    tunnel: [w2175 w2181] -> w2157
                    tunnel: w2150 -> [w2173 w2177]
                    tunnel: w2149 -> [_ w2179]
                    frame True {
                      n597 = call "BRig_dataRT_stats__DAB_nTimeout.vi"() -> ("output_DAB_nTimeout"=w2172:i32)  [unwired: 11 in]
                      n598 = To Unsigned Word Integer(number=w2172) -> (unsigned 16bit integer=w2174:u16)
                      n599 = Build Array(u16 3, w2174, w2173) -> (w2175:u16[])
                    }
                    frame False {
                      n600 = case shown="False" w2179 {
                        tunnel: w2177 -> [w2188 w2190]
                        tunnel: [w2187 w2189] -> w2180
                        frame False {
                          n601 = call "BRig_dataRT_stats__BTPR_cur.vi"() -> ("output_BTPR_cur"=w2187:i32)  [unwired: 11 in]
                          n602 = local write "BTPR_block"(w2188) -> ()
                        }
                        frame True {
                          n603 = call "BRig_dataRT_stats__T2R_cur.vi"() -> ("output_T2R_cur"=w2189:i32)  [unwired: 11 in]
                          n604 = local write "T2R_block"(w2190) -> ()
                        }
                      }
                      n605 = To Unsigned Word Integer(number=w2180) -> (unsigned 16bit integer=w2178:u16)
                      n606 = case shown="True" w2186 {
                        tunnel: w2185 -> [_ w2210]
                        tunnel: w2184 -> [_ w2200]
                        tunnel: w2183 -> [_ w2196]
                        tunnel: u16 3 -> [w2194 w2203]
                        tunnel: w2178 -> [w2193 w2199]
                        tunnel: w2177 -> [w2192 w2202]
                        tunnel: [w2191 w2201] -> w2181
                        frame False {
                          n607 = Build Array(w2194, w2193, w2192) -> (w2191:u16[])
                        }
                        frame True {
                          w2195 = 100.0 ("y")
                          n608 = case shown="False" w2210 {
                            tunnel: w2200 -> [w2213 w2218]
                            tunnel: w2196 -> [w2214 w2217]
                            tunnel: [w2211 w2216] -> w2209
                            tunnel: [w2212 w2215] -> w2208
                            frame False {
                              n609 = local write "BTPR_avg_R"(w2214) -> ()
                              n610 = call "BRig_dataRT_stats__BTPR_avg_R.vi"() -> ("output_BTPR_avg_R__x100"=w2212:i32)  [unwired: 11 in]
                              n611 = local write "T2R_avg_R"(w2213) -> ()
                              n612 = call "BRig_dataRT_stats__T2R_avg_R.vi"() -> ("output_T2R_avg_R__x100"=w2211:i32)  [unwired: 11 in]
                            }
                            frame True {
                              n613 = call "BRig_dataRT_stats__BTPR_avg_L.vi"() -> ("output_BTPR_avg_L__x100"=w2215:i32)  [unwired: 11 in]
                              n614 = local write "BTPR_avg_L"(w2217) -> ()
                              n615 = local write "T2R_avg_L"(w2218) -> ()
                              n616 = call "BRig_dataRT_stats__T2R_avg_L.vi"() -> ("output_T2R_avg_L__x100"=w2216:i32)  [unwired: 11 in]
                            }
                          }
                          n617 = Multiply(x=w2200, y=w2195) -> (x*y=w2197:dbl)
                          n618 = Multiply(x=w2196, y=w2195) -> (x*y=w2198:dbl)
                          n619 = To Unsigned Word Integer(number=w2197) -> (unsigned 16bit integer=w2204:u16)
                          n620 = To Unsigned Word Integer(number=w2198) -> (unsigned 16bit integer=w2205:u16)
                          n621 = To Unsigned Word Integer(number=w2208) -> (unsigned 16bit integer=w2206:u16)
                          n622 = To Unsigned Word Integer(number=w2209) -> (unsigned 16bit integer=w2207:u16)
                          n623 = Build Array(w2203, w2207, w2204, w2203, w2206, w2205, w2203, w2199, w2202) -> (w2201:u16[])
                        }
                      }
                    }
                  }
                  n624 = RT FIFO Write(0:w2158, 1:w2157, 3:w2156) -> ()  [unwired: 2 in, 4 out]
                  n625 = call "BRig_RT_comm_tcp_write_RTwrite__RunState_Trial_selResult__v3.vi"("input_dataTrial"=w2163, "iReward_or_iError"=FALSE, "input_dataCurrent"=w2164) -> ("output_strCmd"=w2155:string)  [unwired: 8 in]
                }
                frame "SelectWrong" {
                  n626 = call "BRig_RT__Case_Exp__generic__incrementCountTilThreshold.vi"("input_dataCurrent"=w2221) -> ("output_dataCurrent"=w2219:u16[], "output_underThreshold"=w2220:bool)  [unwired: 9 in]
                  n627 = Select(t=w2223, s=w2220, f=myRIO_BRig_RT__Case_Exp_stateList."endTrial1" ("Enum")) -> (s? t:f=w2222:T2)
                }
                frame "SelectTimeout" {
                  n628 = call "BRig_RT__Case_Exp__generic__incrementCountTilThreshold.vi"("input_dataCurrent"=w2231) -> ("output_dataCurrent"=w2230:u16[], "output_underThreshold"=w2229:bool)  [unwired: 9 in]
                  n629 = Select(t=w2233, s=w2229, f=myRIO_BRig_RT__Case_Exp_stateList."endTrial1" ("Enum")) -> (s? t:f=w2232:T2)
                }
                frame "endTrial1" {
                  n630 = call "BRig_RT_comm_tcp_write_RTwrite__RunState_Trial_end.vi"("input_dataCurrent"=w2247) -> ("output_strCmd"=w2246:string)  [unwired: 10 in]
                  n631 = call "BRig_RT__Case_Exp__State_endTrial__v10.vi"("input_dataBlock"=w2243, "input_timeStamp_start"=w2248, "input_dataTrial"=w2255, "input_dataCurrent"=w2247) -> ("output_BTPRavg"=w2240:dbl, "output_T2Ravg"=w2241:dbl, "output_dataTrial"=w2254:u16[][], "output_dataCurrent"=w2249:u16[], "output_R(F)_or_L(T)"=w2242:bool, "output_runTime"=→"T_ExpRun_min":dbl)  [unwired: 2 in]
                  n632 = xnode "Read/Write Control"("FPGA VI Reference In"=w2251, "error in"=w2250, "SelectionState"=FALSE) -> ("error out"=w2252:errorcluster)  [unwired: 1 out]
                  n633 = case shown="False" w2242 {
                    tunnel: w2241 -> [w2257 w2260]
                    tunnel: w2240 -> [w2258 w2259]
                    frame False {
                      n634 = local write "BTPR_avg_R"(w2258) -> ()
                      n635 = local write "T2R_avg_R"(w2257) -> ()
                    }
                    frame True {
                      n636 = local write "BTPR_avg_L"(w2259) -> ()
                      n637 = local write "T2R_avg_L"(w2260) -> ()
                    }
                  }
                  n638 = local write "error out"(w2252) -> ()
                }
                frame "endTrial2" {
                  n639 = case shown="True" w2270 {
                    tunnel: [w2278 _] -> w2271
                    tunnel: [w2277 w2280] -> w2266
                    tunnel: w2265 -> [w2275 w2288]
                    tunnel: w2264 -> [w2276 w2286]
                    tunnel: [w2276 w2285] -> w2263
                    tunnel: [w2275 w2287] -> w2262
                    tunnel: w2261 -> [_ w2279]
                    frame False {
                      # "Receive commands"
                      n640 = call "BRig_RT__Case_Exp__UploadClosedLoop__v3.vi"() -> ("all rows"=w2278:i64[][], "output_haveCmd"=w2277:bool)  [unwired: 10 in]
                    }
                    frame True {
                      # "Parse commands and update"
                      n641 = Array Size(array=w2279) -> (size(s)=w2284:i32[])
                      n642 = Index Array(array=w2284, index=0) -> (element=w2282:i32)
                      n643 = Not Equal To 0?(x=w2282) -> (x != 0?=w2281:bool)
                      n644 = case shown="False" w2281 {
                        selector: w2281 -> [w2292 w2294]
                        tunnel: w2288 -> [w2290 w2298]
                        tunnel: [w2290 w2297] -> w2287
                        tunnel: w2286 -> [w2289 w2296]
                        tunnel: [w2289 w2295] -> w2285
                        tunnel: [w2292 w2294] -> w2280
                        tunnel: w2279 -> [_ w2293]
                        frame False {
                          w2291 = TRUE ("input_setValues")
                          # "Update"
                          n645 = call "BRig_RT_panel_cue_v1,18.vi"("input_setValues"=w2291, "input_dataExp"=w2290) -> ()  [unwired: 9 in, 1 out]
                          n646 = call "BRig_RT_panel_ExpStruct_v1,18.vi"("input_setValues"=w2291, "input_dataExp"=w2290) -> ()  [unwired: 9 in, 1 out]
                          n647 = call "BRig_RT_panel_Laser1_v1,18.vi"("input_setValues"=w2291, "input_dataExp"=w2290, "input_dataLC"=w2289) -> ()  [unwired: 7 in, 2 out]
                          n648 = call "BRig_RT_panel_Laser2_v1,18.vi"("input_setValues"=w2291, "input_dataExp"=w2290, "input_dataLC"=w2289) -> ()  [unwired: 7 in, 2 out]
                        }
                        frame True {
                          # "Parse"
                          n649 = call "BRig_RT__Case_Exp__UploadClosedLoop__updateSettings.vi"("input_newSettings"=w2293, "input_dataLC"=w2296, "input_dataExp"=w2298) -> ("output_dataLC"=w2295:u16[], "output_dataExp"=w2297:u16[])  [unwired: 7 in]
                        }
                      }
                    }
                  }
                  n650 = Select(t=myRIO_BRig_RT__Case_Exp_stateList."endTrial2", s=w2266, f=myRIO_BRig_RT__Case_Exp_stateList."endTrial3" ("Enum")) -> (s? t:f=w2267:T2)
                }
                frame "endTrial3" {
                  # "Two cues?"
                  # "Dual Armed Bandit?"
                  n651 = call "BRig_dataExp_I_anySelect.vi"() -> ("output_I_anySelect"=w2306:i32)  [unwired: 11 in]
                  n652 = call "BRig_dataExp_I_Cue2.vi"() -> ("output_I_Cue2"=w2304:i32)  [unwired: 11 in]
                  n653 = call "BRig_RT__Case_Exp__endTrial_checkFreeReward__v17.vi"("input_dataBlock"=w2309, "input_dataExp"=w2300, "input_dataTrial"=w2318, "input_dataCurrent"=w2319) -> ("output_state"=w2310:T2, "output_endBlock"=w2308:bool)  [unwired: 6 in]
                  n654 = Index Array(array=w2300, index #1=w2306, index #2=w2304) -> (element #1=w2305:u16, element #2=w2303:u16)  [unwired: 1 in, 1 out]
                  n655 = Not Equal To 0?(x=w2305) -> (x != 0?=w2302:bool)
                  n656 = Not Equal To 0?(x=w2303) -> (x != 0?=w2301:bool)
                  n657 = local read "STOP_endTrial"() -> (w2317:bool)
                  n658 = Or(x=w2302, y=w2301) -> (x .or. y?=w2299:bool)
                  n659 = local read "STOP_abort"() -> (w2316:bool)
                  n660 = case shown="True" w2299 {
                    tunnel: w2300 -> [w2321 w2322]
                    tunnel: [w2321 w2323] -> w2307
                    frame False {
                    }
                    frame True {
                      # "Get latest\nlaserSwitch"
                      n661 = call "BRig_dataExp_Loop_c_ExpStruct.vi"() -> ("output_Loop_c_ExpStruct"=w2329:i32)  [unwired: 11 in]
                      n662 = call "BRig_dataExp_LaserSwitch.vi"() -> ("output_LaserSwitch"=w2325:i32)  [unwired: 11 in]
                      n663 = Replace Array Subset(array=w2322, new element=u16 2 ("new element/subarray"), index=w2329) -> (w2327:u16[])
                      n664 = call "BRig_RT_panel_ExpStruct_v1,14.vi"("input_setValues"=FALSE, "input_dataExp"=w2327) -> ("output_dataExp"=w2326:u16[])  [unwired: 9 in]
                      n665 = Index Array(array=w2326, index=w2325) -> (element=w2324:u16)
                      n666 = Replace Array Subset(array=w2322, new element=w2324, index=w2325) -> (w2323:u16[])
                    }
                  }
                  n667 = local read "START"() -> (w2314:bool)
                  n668 = Not(x=w2314) -> (.not. x?=w2315:bool)
                  n669 = Compound Arithmetic op=OR(w2317, w2315, w2316, w2308) -> (w2313:bool)
                  n670 = Select(t=myRIO_BRig_RT__Case_Exp_stateList."saveData_dataBlock" ("Enum"), s=w2313, f=w2310) -> (s? t:f=w2311:T2)
                }
                frame "endBlock" {
                  # "Get latest\nlaserSwitch"
                  n671 = call "BRig_dataExp_Loop_c_ExpStruct.vi"() -> ("output_Loop_c_ExpStruct"=w2338:i32)  [unwired: 11 in]
                  n672 = call "BRig_dataExp_LaserSwitch.vi"() -> ("output_LaserSwitch"=w2333:i32)  [unwired: 11 in]
                  n673 = local read "START"() -> (w2357:bool)
                  n674 = local read "STOP_endBlock"() -> (w2353:bool)
                  n675 = local read "STOP_endTrial"() -> (w2355:bool)
                  n676 = local read "STOP_abort"() -> (w2354:bool)
                  n677 = Replace Array Subset(array=w2331, new element=u16 2 ("new element/subarray"), index=w2338) -> (w2336:u16[])
                  n678 = call "BRig_RT_panel_ExpStruct_v1,18.vi"("input_setValues"=FALSE, "input_dataExp"=w2336) -> ("output_dataExp"=w2335:u16[])  [unwired: 9 in]
                  n679 = Index Array(array=w2335, index=w2333) -> (element=w2332:u16)
                  n680 = Not(x=w2357) -> (.not. x?=w2356:bool)
                  n681 = Select(t=myRIO_BRig_RT__Case_Exp_stateList."commUpload_dataTrial" ("Enum"), s=w2343, f=myRIO_BRig_RT__Case_Exp_stateList."initBlock" ("Enum")) -> (s? t:f=w2340:T2)
                  n682 = Replace Array Subset(array=w2331, new element=w2332, index=w2333) -> (w2334:u16[])
                  n683 = Compound Arithmetic op=OR(w2356, w2353, w2355, w2354) -> (w2347:bool)
                  n684 = Select(t=myRIO_BRig_RT__Case_Exp_stateList."endExp" ("Enum"), s=w2347, f=w2340) -> (s? t:f=w2358:T2)
                  n685 = Select(t="<S,E>" ("string"), s=w2347, f="") -> (s? t:f=w2344:string)
                }
                frame "endExp" {
                  n686 = xnode "Read/Write Control"("FPGA VI Reference In"=w2362, "error in"=w2361, "A6_Act"=FALSE) -> ("error out"=w2363:errorcluster)  [unwired: 1 out]
                  n687 = local write "error out"(w2363) -> ()
                }
                frame "commUpload_dataTrial" {
                }
                frame "saveData_dataBlock" {
                  n688 = Increment(x=w2392) -> (x+1=w2390:u16)
                  n689 = Replace Array Subset(array=w2384, new element=u16 2 ("new element/subarray"), index=0) -> (w2378:u16[])
                  n690 = Index Array(array=w2376, index (row)=0) -> (element=w2379:u16[])  [unwired: 1 in]
                  n691 = for {
                    tunnel: w2379 -> [w2402] mode=indexing
                    shift-right: [w2401] -> w2377
                    shift-left: w2378 -> [w2405]
                    i -> [w2404]
                    n692 = Increment(x=w2404) -> (x+1=w2403:i32)
                    n693 = Replace Array Subset(array=w2405, new element=w2402, index=w2403) -> (w2401:u16[])
                  }
                  n694 = RT FIFO Write(0:w2387, 1:w2377, 3:w2386) -> (11:w2389:errorcluster)  [unwired: 2 in, 3 out]
                  n695 = Unbundle By Name(w2389) -> ("code"=w2388:i32)
                  n696 = Greater?(x=w2390, y=u16 3) -> (0:w2398:bool)
                  n697 = Equal To 0?(x=w2388) -> (x = 0?=w2385:bool)
                  n698 = Or(x=w2398, y=w2385) -> (x .or. y?=w2397:bool)
                  n699 = Select(t=myRIO_BRig_RT__Case_Exp_stateList."endBlock" ("Enum"), s=w2397, f=w2393) -> (s? t:f=w2391:T2)
                }
                frame "saveData_dataTrial" {
                  n700 = Increment(x=w2423) -> (x+1=w2422:u16)
                  n701 = Replace Array Subset(array=w2408, new element=u16 1 ("new element/subarray"), index=0) -> (w2412:u16[])
                  n702 = Index Array(array=w2407, index (row)=0) -> (element=w2413:u16[])  [unwired: 1 in]
                  n703 = for {
                    tunnel: w2413 -> [w2432] mode=indexing
                    shift-right: [w2431] -> w2411
                    shift-left: w2412 -> [w2435]
                    i -> [w2434]
                    n704 = Increment(x=w2434) -> (x+1=w2433:i32)
                    n705 = Replace Array Subset(array=w2435, new element=w2432, index=w2433) -> (w2431:u16[])
                  }
                  n706 = RT FIFO Write(0:w2410, 1:w2411, 3:w2409) -> (11:w2418:errorcluster)  [unwired: 2 in, 3 out]
                  n707 = Unbundle By Name(w2418) -> ("code"=w2417:i32)
                  n708 = Equal To 0?(x=w2417) -> (x = 0?=w2406:bool)
                  n709 = Greater?(x=w2422, y=u16 3) -> (0:w2420:bool)
                  n710 = Or(x=w2420, y=w2406) -> (x .or. y?=w2419:bool)
                  n711 = Select(t=myRIO_BRig_RT__Case_Exp_stateList."endTrial2" ("Enum"), s=w2419, f=w2424) -> (s? t:f=w2425:T2)
                }
                frame "dummyState" {
                  n712 = call "BRig_dataCurrent_iTrial.vi"() -> ("output_iTrial"=w2442:i32)  [unwired: 11 in]
                  n713 = Index Array(array=w2443, index=w2442) -> (element=w2441:u16)
                  n714 = Equal?(x=w2441, y=u16 1) -> (x = y?=w2439:bool)
                  n715 = Equal To 0?(x=w2450) -> (x = 0?=w2451:bool)
                  n716 = Select(t=u16 13, s=w2439, f=u16 15) -> (s? t:f=w2436:u16)
                  n717 = Select(t=w2436, s=w2451, f=w2450) -> (s? t:f=w2449:u16)
                  n718 = Decrement(x=w2449) -> (x-1=w2448:u16)
                  n719 = Equal To 0?(x=w2448) -> (x = 0?=w2447:bool)
                  n720 = Select(t=myRIO_BRig_RT__Case_Exp_stateList."initTrial" ("Enum"), s=w2447, f=w2445) -> (s? t:f=w2444:T2)
                }
                frame "dummyState_endBlock" {
                  n721 = call "BRig_dataCurrent_iTrial.vi"() -> ("output_iTrial"=w2466:i32)  [unwired: 11 in]
                  n722 = Index Array(array=w2460, index=w2466) -> (element=w2456:u16)
                  n723 = Equal?(x=w2456, y=u16 1) -> (x = y?=w2464:bool)
                  n724 = Equal To 0?(x=w2457) -> (x = 0?=w2468:bool)
                  n725 = Select(t=u16 1, s=w2464, f=u16 3) -> (s? t:f=w2461:u16)
                  n726 = Select(t=w2461, s=w2468, f=w2457) -> (s? t:f=w2467:u16)
                  n727 = Decrement(x=w2467) -> (x-1=w2458:u16)
                  n728 = Equal To 0?(x=w2458) -> (x = 0?=w2459:bool)
                  n729 = Select(t=myRIO_BRig_RT__Case_Exp_stateList."initBlock" ("Enum"), s=w2459, f=w2470) -> (s? t:f=w2469:T2)
                }
                frame "FreeReward_pre" {
                  w2506 = u16 0 ("new element/subarray")
                  # "Duration = MTrig duration"
                  # "Duration = Reward Time"
                  n730 = call "BRig_dataCurrent_FreeReward_c.vi"() -> ("output_FreeReward_c"=w2507:i32)  [unwired: 11 in]
                  n731 = call "BRig_dataCurrent_iSpout.vi"() -> ("output_iSpout"=w2504:i32)  [unwired: 11 in]
                  n732 = call "BRig_dataCurrent_c_generic.vi"() -> ("output_count_generic"=w2513:i32)  [unwired: 11 in]
                  n733 = call "BRig_dataCurrent_T_generic.vi"() -> ("output_T_generic"=w2512:i32)  [unwired: 11 in]
                  n734 = Index Array(array=w2505, index=w2504) -> (element=w2503:u16)
                  n735 = call "BRig_dataMTrig_Solenoid_T_L.vi"() -> ("output_Solenoid_T_L"=w2502:i32)  [unwired: 11 in]
                  n736 = call "BRig_dataMTrig_Solenoid_T_R.vi"() -> ("output_Solenoid_T_R"=w2501:i32)  [unwired: 11 in]
                  n737 = local read "FPGA_count2ms"() -> (w2483:dbl)
                  n738 = call "BRig_dataTrial_T_Reward.vi"() -> ("output_T_Reward"=w2508:i32)  [unwired: 11 in]
                  n739 = Equal To 0?(x=w2503) -> (x = 0?=w2485:bool)
                  n740 = Select(t=w2502, s=w2485, f=w2501) -> (s? t:f=w2499:i32)
                  n741 = Index Array(array=w2509, index (row)=0 ("disabled index (row)"), index (col)=w2508) -> ()  [unwired: 1 out]
                  n742 = Index Array(array=w2500, index=w2499) -> (element=w2496:u16)
                  n743 = Replace Array Subset(array=w2505, new element #1=w2506, index #1=w2507, new element #2=w2506, index #2=w2513, new element #3=w2496, index #3=w2512) -> (w2511:u16[])
                  n744 = To Double Precision Float(number=w2496) -> (double precision float=w2484:dbl)
                  n745 = Multiply(x=w2484, y=w2483) -> (x*y=w2497:dbl)
                  n746 = call "BRig_dataExp_FreeReward_c_L.vi"() -> ("output_FreeReward_c_L"=w2490:i32)  [unwired: 11 in]
                  n747 = call "BRig_dataExp_FreeReward_c_R.vi"() -> ("output_FreeReward_c_R"=w2491:i32)  [unwired: 11 in]
                  n748 = Round Toward +Infinity(x=w2497) -> (ceil(x): smallest int >= x=w2498:dbl)
                  n749 = Select(t=w2490, s=w2485, f=w2491) -> (s? t:f=w2487:i32)
                  n750 = To Unsigned Long Integer(number=w2498) -> (unsigned 32bit integer=w2493:u32)
                  n751 = xnode "Read/Write Control"("FPGA VI Reference In"=w2495, "error in"=w2494, "Solenoid_nTotal_L"=w2493, "Solenoid_nTotal_R"=w2493) -> ()  [unwired: 2 out]
                  n752 = Index Array(array=w2488, index=w2487) -> (element=w2486:u16)
                  n753 = Increment(x=w2486) -> (x+1=w2476:u16)
                  n754 = case shown="True" w2485 {
                    tunnel: w2476 -> [w2517 w2519]
                    tunnel: [w2516 w2518] -> w2478
                    frame True {
                      n755 = local write "FreeReward_c_L"(w2517) -> ()
                      n756 = call "BRig_dataRT_stats__FreeReward_c_L.vi"() -> ("output_FreeReward_c_L"=w2516:i32)  [unwired: 11 in]
                    }
                    frame False {
                      n757 = local write "FreeReward_c_R"(w2519) -> ()
                      n758 = call "BRig_dataRT_stats__FreeReward_c_R.vi"() -> ("output_FreeReward_c_R"=w2518:i32)  [unwired: 11 in]
                    }
                  }
                  n759 = To Unsigned Word Integer(number=w2478) -> (unsigned 16bit integer=w2477:u16)
                  n760 = Build Array(u16 3, w2477, w2476) -> (w2482:u16[])
                  n761 = Replace Array Subset(array=w2488, new element=w2476, index=w2487) -> (w2489:u16[])
                  n762 = RT FIFO Write(0:w2480, 1:w2482, 3:w2479) -> ()  [unwired: 2 in, 4 out]
                }
                frame "FreeReward" {
                  n763 = call "BRig_dataCurrent_iSpout.vi"() -> ("output_iSpout"=w2530:i32)  [unwired: 11 in]
                  n764 = call "BRig_dataCurrent_c_generic.vi"() -> ("output_count_generic"=w2524:i32)  [unwired: 11 in]
                  n765 = Index Array(array=w2531, index #1=w2530, index #2=w2524) -> (element #1=w2529:u16, element #2=w2523:u16)
                  n766 = Equal To 0?(x=w2529) -> (x = 0?=w2527:bool)
                  n767 = Equal To 0?(x=w2523) -> (x = 0?=w2522:bool)
                  n768 = Not(x=w2527) -> (.not. x?=w2528:bool)
                  n769 = call "BRig_RT__Case_Exp__generic__incrementCountTilThreshold.vi"("input_dataCurrent"=w2531) -> ("output_dataCurrent"=w2532:u16[], "output_underThreshold"=w2521:bool)  [unwired: 9 in]
                  n770 = Select(t=w2535, s=w2521, f=myRIO_BRig_RT__Case_Exp_stateList."FreeRewardPost_pre" ("Enum")) -> (s? t:f=w2533:T2)
                  n771 = And(x=w2521, y=w2522) -> (x .and. y?=w2520:bool)
                  n772 = And(x=w2520, y=w2527) -> (x .and. y?=w2525:bool)
                  n773 = And(x=w2520, y=w2528) -> (x .and. y?=w2526:bool)
                }
                frame "FreeRewardPost" {
                  n774 = call "BRig_RT__Case_Exp__generic__incrementCountTilThreshold.vi"("input_dataCurrent"=w2542) -> ("output_dataCurrent"=w2541:u16[], "output_underThreshold"=w2540:bool)  [unwired: 9 in]
                  n775 = Select(t=w2545, s=w2540, f=myRIO_BRig_RT__Case_Exp_stateList."initTrial" ("Enum")) -> (s? t:f=w2543:T2)
                }
                frame "FreeRewardPost_pre" {
                  n776 = call "BRig_dataExp_T_RewardPost.vi"() -> ("output_T_RewardPost"=w2555:i32)  [unwired: 11 in]
                  n777 = call "BRig_dataCurrent_c_generic.vi"() -> ("output_count_generic"=w2558:i32)  [unwired: 11 in]
                  n778 = call "BRig_dataCurrent_T_generic.vi"() -> ("output_T_generic"=w2557:i32)  [unwired: 11 in]
                  n779 = Index Array(array=w2552, index=w2555) -> (element=w2554:u16)
                  n780 = Replace Array Subset(array=w2553, new element #1=u16 0 ("new element/subarray"), index #1=w2558, new element #2=w2554, index #2=w2557) -> (w2551:u16[])
                }
              }
              n781 = call "BRig_RT_panel_manualTriggering_v0,90.vi"("input_dataMTrig"=w1357) -> ("output_Solenoid_R"=w1366:bool, "output_Solenoid_L"=w1365:bool, "output_dataMTrig"=w1398:u16[], "output_Audio_L"=w1397:bool, "output_Audio_R"=w1396:bool, "output_CueLed"=w1394:bool, "output_Laser_l1"=w1370:bool, "output_Laser_l2"=w1390:bool)  [unwired: 11 in]
              n782 = call "BRig_RT__Case_Exp__comm_tcp__data_other.vi"("input_strState"=w1358, "input_strAccum"=w1359, "input_error"=w1360, "input_hTCP"=w1361, "input_I_connected_TCP"=w1362) -> ("output_strAccum"=w1343:string, "output_error"=w1342:errorcluster, "output_hTCP"=w1344:refnum<k5>, "output_I_connect_TCP"=w1345:bool)  [unwired: 3 in]
              n783 = Or(x="STOP_abort", y=w1382) -> (x .or. y?=w1346:bool)
              n784 = Or(x=w1395, y=w1394) -> (x .or. y?=w1373:bool)
              n785 = local read "Laser1_LED"() -> (w1333:bool)
              n786 = local read "Laser2_LED"() -> (w1332:bool)
              n787 = Or(x=w1397, y=w1412) -> (x .or. y?=w1372:bool)
              n788 = Or(x=w1411, y=w1396) -> (x .or. y?=w1371:bool)
              n789 = Or(x=w1369, y=w1370) -> (x .or. y?=w1389:bool)
              n790 = Or(x=w1393, y=w1390) -> (x .or. y?=w1391:bool)
              n791 = call "BRig_RT__Case_Exp__recordLick.vi"("input_dataLick"=w1381, "input_lick__R"=w1375, "input_lick__L"=w1376, "input_lick"=w1377, "intput_state__trialStart"=w1337, "intput_state__trialEnd"=w1380, "input_dataCurrent"=w1379) -> ("output_dataLick"=w1374:u16[][], "output_dataCurrent"=w1378:u16[])  [unwired: 7 in]
              n792 = xnode "Read/Write Control"("FPGA VI Reference In"=w1410, "error in"=w1409, "L1Led_ON"=w1333, "L2Led_ON"=w1332, "Solenoid_trig_L"=w1364, "Solenoid_trig_R"=w1363, "A3_SL"=w1365, "A1_SR"=w1366, "LC_Event_l1"=w1388, "LC_Laser_l1"=w1389, "LC_Event_l2"=w1392, "LC_Laser_l2"=w1391, "CueLed_Event"=w1373, "audioTrigger_L"=w1372, "audioTrigger_R"=w1371) -> ("FPGA VI Reference Out"=w1416:refnum<k20>, "error out"=w1415:errorcluster, "fpga_laser1"=w1331:bool, "fpga_laser2"=w1330:bool, "fpga_solenoid_L"=w1329:bool, "fpga_solenoid_R"=w1328:bool)
              n793 = local write "Laser1"(w1331) -> ()
              n794 = local write "Laser2"(w1330) -> ()
              n795 = local write "Solenoid L"(w1329) -> ()
              n796 = local write "Solenoid R"(w1328) -> ()
              n797 = Not(x=w1311) -> (.not. x?=w1310:bool)
              n798 = call "BRig_RT__Case_Exp__recordAnalogInput__PortA__fifo__1value__v2.vi"("input_iOccurence"=w1386, "resetOccurrence"=w1385, "input_dataCurrent"=w1379, "input_AnaIn_array"=w1307, "input_iState_start"=w1337, "rt fifo"=w1336, "input_iState_end"=w1380, "input_fifo_error"=w1335) -> ("output_fifo_error"=w1341:errorcluster, "output_iOccurrence"=w1387:u16)  [unwired: 9 in, 1 out]
              n799 = call "BRig_RT_timeLoop_Exp__noStateLimit.vi"("input_error"=w1341, "input_Threshold_reset"="input_Threshold_reset", "input_Threshold"=w1401, "input_timestamp"=w1402, "input_state"=w1337) -> ("output_Threshold"=w1399:bool, "output_duration"=→"tLoop":dbl)  [unwired: 4 in, 1 out]
              "Threshold" <- w1399
              n800 = node-c288() -> ()  [unwired: 1 in, 1 out]
            }
            "stop_TimedLoop" <- w908
            n801 = while {
              tunnel: w852 -> [w976]
              tunnel: w851 -> [w975]
              shift-right: [w970] -> _
              shift-left: 0 ("element") -> [w971]
              shift-right: [w966] -> _
              shift-left: w857 -> [w972]
              tunnel: [w969] -> w854
              tunnel: [w968] -> w853
              tunnel: w850 -> [w965]
              tunnel: w849 -> [w964]
              tunnel: [w963] -> w848
              tunnel: [w962] -> w847
              shift-right: [w960] -> _
              shift-left: FALSE -> [w961]
              stop <- w959 stop-if-true
              # "If buffer is full, send to Host"
              # "Collect analog input data in groups of 16"
              # "Receive latest analog input"
              # "This non-timed loop receives AnalogInput\ndata and passes it to the Host"
              # "timed out?"
              n802 = RT FIFO Read(0:w976, 3:w975) -> (8:w969:refnum<k33>, 9:w973:u16, 10:w980:bool, 11:w977:errorcluster)  [unwired: 2 in, 1 out]
              n803 = Unbundle By Name(w977) -> ("code"=w981:i32)
              n804 = Not(x=w980) -> (.not. x?=w979:bool)
              n805 = Equal To 0?(x=w981) -> (x = 0?=w978:bool)
              n806 = And(x=w978, y=w979) -> (x .and. y?=w974:bool)
              n807 = Select(t=w977, s=w978, f=w975) -> (s? t:f=w968:errorcluster)
              n808 = case shown="True" w974 {
                tunnel: w973 -> [_ w1012]
                tunnel: w972 -> [w1004 w1014]
                tunnel: w971 -> [w1003 w1011]
                tunnel: [w1004 w1013] -> w966
                tunnel: [w1003 w1007] -> w970
                tunnel: [_ w1005] -> w967
                frame False {
                }
                frame True {
                  n809 = Replace Array Subset(array=w1014, new element=w1012, index=w1011) -> (w1013:u16[])
                  n810 = Increment(x=w1011) -> (x+1=w1009:i32)
                  n811 = Less?(x=w1011, y=15 ("dimension size")) -> (x < y?=w1006:bool)
                  n812 = Select(t=w1009, s=w1006, f=0) -> (s? t:f=w1007:i32)
                  n813 = Not(x=w1006) -> (.not. x?=w1005:bool)
                }
              }
              n814 = case shown="True" w967 {
                tunnel: w966 -> [_ w993]
                tunnel: w965 -> [w984 w992]
                tunnel: w964 -> [w983 w991]
                tunnel: [w984 w989] -> w963
                tunnel: [w983 w988] -> w962
                tunnel: w961 -> [w982 w986]
                tunnel: [w982 w985] -> w960
                frame False {
                }
                frame True {
                  n815 = for {
                    N: 16 -> [_]
                    tunnel: w993 -> [w1000] mode=indexing
                    tunnel: w992 -> [w1002]
                    tunnel: w991 -> [w1001]
                    shift-right: [w995] -> w987
                    shift-left: FALSE -> [w999]
                    tunnel: [w998] -> w989
                    tunnel: [w997] -> w988
                    n816 = shared-variable-write(w1002, w1001, w1000) -> (w998:refnum<k21>, w997:errorcluster, w996:bool)  [unwired: 1 in]
                    n817 = Or(x=w999, y=w996) -> (x .or. y?=w995:bool)
                  }
                  n818 = Or(x=w986, y=w987) -> (x .or. y?=w985:bool)
                }
              }
              n819 = local read "stop_TimedLoop"() -> (w959:bool)
            }
            n820 = while {
              shift-right: [w1098] -> _
              shift-left: 0 -> [w1087]
              tunnel: w905 -> [w1105]
              tunnel: w897 -> [w1107]
              shift-right: [w1094] -> _
              shift-left: 0 -> [w1089]
              shift-right: [w1099] -> _
              shift-left: w844 -> [w1106]
              shift-right: [w1095] -> _
              shift-left: w872 -> [w1108]
              shift-right: [w1102] -> w894
              shift-left: w866 -> [w1115]
              shift-right: [w1103] -> w888
              shift-left: w865 -> [w1109]
              tunnel: w869 -> [w1092]
              tunnel: w873 -> [w1091]
              shift-right: [w1080] -> _
              shift-left: w839 -> [w1086]
              shift-right: [w1079] -> _
              shift-left: 0 -> [w1085]
              tunnel: w842 -> [w1083]
              tunnel: w841 -> [w1084]
              tunnel: [w1078] -> w836
              tunnel: [w1077] -> w835
              stop <- w1116 stop-if-true
              # "This non-timed loop received Trial/Block status information\nand passes it on the Host. This includes stats such as\nnumber of total rewards or target trials per block"
              # "nColumns dataBlock"
              # "nColumns dataTrial"
              # "buffer_dataTrial"
              # "buffer_dataBlock"
              # "buffer_dataTrial"
              # "buffer_dataBlock"
              n821 = local read "stop_TimedLoop"() -> (w1116:bool)
              n822 = Not Equal To 0?(x=w1089) -> (x != 0?=w1090:bool)
              n823 = Not Equal To 0?(x=w1085) -> (x != 0?=w1076:bool)
              n824 = case shown="True" w1090 {
                tunnel: w1108 -> [w1268 w1271]
                tunnel: w1089 -> [w1269 w1273]
                tunnel: w1107 -> [_ w1282]
                tunnel: [w1269 w1270] -> w1096
                tunnel: [w1268 w1271] -> w1097
                frame False {
                }
                frame True {
                  n825 = Array Subset(array=w1271, length (row)=w1273) -> (w1284:u16[][])  [unwired: 3 in]
                  n826 = call "BRig_dataBlock_iBlock.vi"() -> ("output_iBlock"=w1279:i32)  [unwired: 11 in]
                  n827 = Index Array(array=w1271, index (row)=0, index (col)=w1279) -> (element=w1278:u16)
                  n828 = To Double Precision Float(number=w1284) -> (double precision float=w1283:dbl[][])
                  n829 = Not Equal?(x=u16 1, y=w1278) -> (x != y?=w1276:bool)
                  n830 = call-poly <vilib>:"Write To Spreadsheet File.vi"("delimiter (\\t)"="," ("delimiter (\\t)"), "append to file? (new file:F)"=w1276, "2D data"=w1283, "file path (dialog if empty)"=w1282) -> ("new file path (Not A Path if cancelled)"=w1275:path)  [unwired: 4 in]
                  n831 = call <vilib>:"Is Path and Not Empty.vi"("path"=w1275) -> ("Is Path and Not Empty?"=w1274:bool)  [unwired: 4 in]
                  n832 = Select(t=0, s=w1274, f=w1273) -> (s? t:f=w1270:i32)
                }
              }
              n833 = case shown="True" w1076 {
                tunnel: w1086 -> [w1120 w1129]
                tunnel: w1085 -> [w1119 w1122]
                tunnel: [w1119 w1128] -> w1081
                tunnel: [w1120 w1129] -> w1082
                tunnel: w1084 -> [w1118 w1137]
                tunnel: w1083 -> [w1117 w1136]
                tunnel: [w1118 w1127] -> w1078
                tunnel: [w1117 w1126] -> w1077
                frame False {
                }
                frame True {
                  n834 = Decrement(x=w1122) -> (x-1=w1121:i32)
                  n835 = Multiply(x=w1121, y=2 ("index")) -> (x*y=w1123:i32)
                  n836 = Increment(x=w1123) -> (x+1=w1124:i32)
                  n837 = Index Array(array=w1129, index #1=w1123, index #2=w1124) -> (element #1=w1135:u16, element #2=w1131:u16)
                  n838 = shared-variable-write(w1137, w1136, w1135) -> (w1132:refnum<k21>, w1133:errorcluster, w1134:bool)  [unwired: 1 in]
                  n839 = case shown="False" w1134 {
                    selector: w1134 -> [_ w1146]
                    tunnel: w1133 -> [w1143 w1144]
                    tunnel: w1132 -> [w1142 w1145]
                    tunnel: w1131 -> [w1141 _]
                    tunnel: [w1140 w1146] -> w1130
                    tunnel: [w1139 w1145] -> w1127
                    tunnel: [w1138 w1144] -> w1126
                    frame False {
                      n840 = shared-variable-write(w1142, w1143, w1141) -> (w1139:refnum<k21>, w1138:errorcluster, w1140:bool)  [unwired: 1 in]
                    }
                    frame True {
                    }
                  }
                  n841 = Select(t=w1122, s=w1130, f=w1121) -> (s? t:f=w1128:i32)
                }
              }
              n842 = RT FIFO Read(0:w1115, 3:w1109) -> (8:w1102:refnum<k33>, 9:w1093:u16[], 10:w1113:bool, 11:w1110:errorcluster)  [unwired: 2 in, 1 out]
              n843 = Unbundle By Name(w1110) -> ("code"=w1114:i32)
              n844 = Not(x=w1113) -> (.not. x?=w1112:bool)
              n845 = Equal To 0?(x=w1114) -> (x = 0?=w1111:bool)
              n846 = And(x=w1111, y=w1112) -> (x .and. y?=w1104:bool)
              n847 = Select(t=w1110, s=w1111, f=w1109) -> (s? t:f=w1103:errorcluster)
              n848 = Not Equal To 0?(x=w1087) -> (x != 0?=w1088:bool)
              n849 = case shown="True" w1088 {
                tunnel: w1106 -> [w1251 w1254]
                tunnel: w1087 -> [w1252 w1256]
                tunnel: w1105 -> [_ w1265]
                tunnel: [w1252 w1253] -> w1100
                tunnel: [w1251 w1254] -> w1101
                frame False {
                }
                frame True {
                  n850 = Array Subset(array=w1254, length (row)=w1256) -> (w1267:u16[][])  [unwired: 3 in]
                  n851 = call "BRig_dataTrial_nTrial.vi"() -> ("output_nTrial"=w1262:i32)  [unwired: 11 in]
                  n852 = Index Array(array=w1254, index (row)=0, index (col)=w1262) -> (element=w1261:u16)
                  n853 = To Double Precision Float(number=w1267) -> (double precision float=w1266:dbl[][])
                  n854 = Not Equal?(x=u16 1, y=w1261) -> (x != y?=w1259:bool)
                  n855 = call-poly <vilib>:"Write To Spreadsheet File.vi"("delimiter (\\t)"="," ("delimiter (\\t)"), "append to file? (new file:F)"=w1259, "2D data"=w1266, "file path (dialog if empty)"=w1265) -> ("new file path (Not A Path if cancelled)"=w1258:path)  [unwired: 4 in]
                  n856 = call <vilib>:"Is Path and Not Empty.vi"("path"=w1258) -> ("Is Path and Not Empty?"=w1257:bool)  [unwired: 4 in]
                  n857 = Select(t=0, s=w1257, f=w1256) -> (s? t:f=w1253:i32)
                }
              }
              n858 = case shown="True" w1104 {
                tunnel: w1101 -> [w1153 w1173]
                tunnel: w1100 -> [w1152 w1171]
                tunnel: [w1153 w1172] -> w1099
                tunnel: [w1152 w1170] -> w1098
                tunnel: w1097 -> [w1151 w1169]
                tunnel: w1096 -> [w1150 w1167]
                tunnel: [w1151 w1168] -> w1095
                tunnel: [w1150 w1166] -> w1094
                tunnel: w1093 -> [_ w1174]
                tunnel: w1092 -> [_ w1165]
                tunnel: w1091 -> [_ w1164]
                tunnel: w1082 -> [w1148 w1157]
                tunnel: w1081 -> [w1147 w1156]
                tunnel: [w1148 w1155] -> w1080
                tunnel: [w1147 w1154] -> w1079
                frame False {
                  n859 = Wait (ms)(milliseconds to wait=u32 10) -> ()  [unwired: 1 out]
                }
                frame True {
                  n860 = Index Array(array=w1174, index=0) -> (element=w1158:u16)
                  n861 = Equal?(x=w1158, y=u16 1) -> (x = y?=w1159:bool)
                  n862 = Equal?(x=w1158, y=u16 2) -> (x = y?=w1161:bool)
                  n863 = Or(x=w1159, y=w1161) -> (x .or. y?=w1160:bool)
                  n864 = case shown="False" w1160 {
                    tunnel: w1174 -> [w1182 w1230]
                    tunnel: w1173 -> [w1186 w1223]
                    tunnel: [w1186 w1222] -> w1172
                    tunnel: w1171 -> [w1185 w1221]
                    tunnel: [w1185 w1220] -> w1170
                    tunnel: w1169 -> [w1184 w1227]
                    tunnel: [w1184 w1225] -> w1168
                    tunnel: w1167 -> [w1183 w1226]
                    tunnel: [w1183 w1224] -> w1166
                    tunnel: w1165 -> [_ w1229]
                    tunnel: w1164 -> [_ w1228]
                    tunnel: w1159 -> [_ w1219]
                    tunnel: w1158 -> [w1187 _]
                    tunnel: w1157 -> [w1179 w1218]
                    tunnel: w1156 -> [w1180 w1217]
                    tunnel: [w1178 w1218] -> w1155
                    tunnel: [w1177 w1217] -> w1154
                    frame False {
                      n865 = Equal?(x=w1187, y=u16 3) -> (x = y?=w1176:bool)
                      n866 = case shown="True" w1176 {
                        tunnel: w1182 -> [_ w1194]
                        tunnel: w1180 -> [w1188 w1193]
                        tunnel: w1179 -> [w1189 w1192]
                        tunnel: [w1189 w1191] -> w1178
                        tunnel: [w1188 w1190] -> w1177
                        frame False {
                        }
                        frame True {
                          w1201 = 3 ("y")
                          n867 = Array Size(array=w1194) -> (size(s)=w1195:i32)
                          n868 = To Double Precision Float(number=w1195) -> (double precision float=w1196:dbl)
                          n869 = To Double Precision Float(number=w1201) -> (double precision float=w1200:dbl)
                          n870 = Divide(x=w1196, y=w1200) -> (x/y=w1197:dbl)
                          n871 = Round Toward -Infinity(1:w1197) -> (0:w1198:dbl)
                          n872 = To Long Integer(number=w1198) -> (32bit integer=w1199:i32)
                          n873 = for {
                            N: w1199 -> [_]
                            tunnel: w1201 -> [w1216]
                            tunnel: w1194 -> [w1213]
                            shift-right: [w1202] -> w1190
                            shift-left: w1193 -> [w1208]
                            shift-right: [w1203] -> w1191
                            shift-left: w1192 -> [w1210]
                            i -> [w1215]
                            n874 = Multiply(x=2 ("index"), y=w1208) -> (x*y=w1207:i32)
                            n875 = Multiply(x=w1215, y=w1216) -> (x*y=w1214:i32)
                            n876 = Increment(x=w1214) -> (x+1=w1212:i32)
                            n877 = Increment(x=w1212) -> (x+1=w1211:i32)
                            n878 = Increment(x=w1208) -> (x+1=w1202:i32)
                            n879 = Index Array(array=w1213, index #1=w1212, index #2=w1211) -> (element #1=w1205:u16, element #2=w1204:u16)
                            n880 = Increment(x=w1207) -> (x+1=w1206:i32)
                            n881 = Replace Array Subset(array=w1210, new element #1=w1205, index #1=w1207, new element #2=w1204, index #2=w1206) -> (w1203:u16[])
                          }
                        }
                      }
                    }
                    frame True {
                      n882 = case shown="True" w1219 {
                        tunnel: w1230 -> [w1238 w1250]
                        tunnel: w1229 -> [w1236 _]
                        tunnel: w1228 -> [_ w1245]
                        tunnel: w1227 -> [w1240 w1244]
                        tunnel: w1226 -> [w1239 w1246]
                        tunnel: [w1240 w1243] -> w1225
                        tunnel: [w1239 w1242] -> w1224
                        tunnel: w1223 -> [w1235 w1247]
                        tunnel: [w1233 w1247] -> w1222
                        tunnel: w1221 -> [w1232 w1241]
                        tunnel: [w1231 w1241] -> w1220
                        frame True {
                          n883 = Array Subset(array=w1238, index=1, length=w1236) -> (w1234:u16[])
                          n884 = Increment(x=w1232) -> (x+1=w1231:i32)
                          n885 = Replace Array Subset(array=w1235, new element=w1234, index (row)=w1232) -> (w1233:u16[][])  [unwired: 1 in]
                        }
                        frame False {
                          n886 = Array Subset(array=w1250, index=1, length=w1245) -> (w1248:u16[])
                          n887 = Increment(x=w1246) -> (x+1=w1242:i32)
                          n888 = Replace Array Subset(array=w1244, new element=w1248, index (row)=w1246) -> (w1243:u16[][])  [unwired: 1 in]
                        }
                      }
                    }
                  }
                }
              }
            }
            n889 = node-c288(w957) -> ()  [unwired: 1 out]
            n890 = RT FIFO Delete(0:w894, 2:TRUE ("force destroy? (F)"), 3:w888) -> ()  [unwired: 1 out]
            n891 = RT FIFO Delete(0:w854, 2:TRUE ("force destroy? (F)"), 3:w853) -> ()  [unwired: 1 out]
            n892 = flat-sequence {
              tunnel: w928 -> [w1286]
              tunnel: w927 -> [w1289]
              tunnel: w926 -> [w1288]
              tunnel: w925 -> [w1287]
              tunnel: w924 -> [w1291]
              tunnel: w922 -> [_]
              tunnel: w845 -> [w1293]
              tunnel: w892 -> [w1292]
              tunnel: [w1285] -> w903
              tunnel: w888 -> [_]
              tunnel: w921 -> [w1304]
              tunnel: w920 -> [w1303]
              tunnel: w919 -> [w1302]
              tunnel: [w1301] -> w918
              tunnel: [w1300] -> w917
              tunnel: [w1295] -> w913
              tunnel: w903 -> [w1294]
              frame #0 {
                # "Store"
                n893 = call "BRig_RT__Case_Exp__storeData__endExp__v5__p1.vi"("input_dataCurrent"=w1287, "input_dataLC"=w1292, "input_dataExp"=w1293, "input_dataExp_end"=w1288, "input_dataLC_end"=w1289) -> ("output_True"=w1290:bool)  [unwired: 10 in]
                n894 = call "BRig_RT__Case_Exp__storeData__endExp__v5__p2.vi"("input_dataCurrent"=w1287, "input_dataLick"=w1291, "input_True"=w1290, "input_dataMTrig"=w1286) -> ("output_True"=w1285:bool)  [unwired: 11 in]
              }
              frame #1 {
                # "Send"
                n895 = local read "Data Set Prefix"() -> (w1296:string)
                n896 = call "BRig_RT_comm_webdav_upload_all__v3.vi"("input_I_connected_webdav"=w1302, "input_fileName_prefix"=w1296, "input_hSession"=w1303, "input_error"=w1304, "input_True"=w1294) -> ("output_hSession"=w1300:T4, "error out"=w1301:errorcluster, "output_nFilenames"=w1297:i32, "output_arrFilenames"=w1298:string[], "output_uploaded"=w1299:bool[], "output_strCmd"=w1295:string)  [unwired: 5 in]
                n897 = call "BRig_RT_comm_webdav_upload_all_warnUser.vi"("input_n"=w1297, "input_arrFilenames"=w1298, "input_arrUploaded"=w1299) -> ()  [unwired: 9 in]
              }
            }
            n898 = flat-sequence {
              tunnel: w937 -> [w1305]
              tunnel: [w1305] -> w923
              frame #0 {
                w1306 = FALSE ("START")
                n899 = local write "START"(w1306) -> ()
                n900 = local write "STOP_endTrial"(w1306) -> ()
                n901 = local write "STOP_endBlock"(w1306) -> ()
              }
            }
            n902 = xnode "Read/Write Control"("FPGA VI Reference In"=w954, "error in"=w923, "Counts_Reset"=TRUE, "audioTrigger_L"=w940, "audioFreq_L_kHz"=w938, "audioAmp_L"=w939, "audioTrigger_R"=w940, "audioFreq_R_kHz"=w938, "audioAmp_R"=w939, "A3_SL"=w940, "A1_SR"=w940, "A6_Act"=w940) -> ("FPGA VI Reference Out"=w953:refnum<k20>, "error out"=w922:errorcluster)
            n903 = call "BRig_RT__Case_Exp__comm_tcp__data_other.vi"("input_strState"=w913, "input_strAccum"="" ("f"), "input_error"=w914, "input_hTCP"=w915, "input_I_connected_TCP"=w916) -> ("output_error"=w909:errorcluster, "output_hTCP"=w910:refnum<k5>, "output_I_connect_TCP"=w911:bool)  [unwired: 3 in, 1 out]
          }
        }
        n904 = local read "STOP_abort"() -> (w328:bool)
      }
    }
  }
  n905 = flat-sequence {
    tunnel: w96 -> [w2573]
    tunnel: w95 -> [w2575]
    tunnel: w89 -> [w2574]
    tunnel: [w2574] -> w101
    tunnel: [w2573] -> w100
    tunnel: [w2572] -> w99
    tunnel: w74 -> [w2571]
    tunnel: [w2571] -> w98
    tunnel: w75 -> [w2570]
    tunnel: [w2570] -> w97
    tunnel: w82 -> [w2568]
    tunnel: w81 -> [w2567]
    tunnel: w80 -> [w2566]
    tunnel: w76 -> [w2569]
    tunnel: [w2569] -> w94
    tunnel: w93 -> [_]
    tunnel: [w2568] -> w88
    tunnel: [w2567] -> w87
    tunnel: [w2566] -> w86
    tunnel: w101 -> [w2595]
    tunnel: w100 -> [w2594]
    tunnel: w99 -> [w2593]
    tunnel: [w2592] -> _
    tunnel: w98 -> [w2591]
    tunnel: w97 -> [w2590]
    tunnel: w94 -> [w2589]
    tunnel: w88 -> [w2588]
    tunnel: w87 -> [w2587]
    tunnel: w86 -> [w2586]
    frame #0 {
      # "Stop FPGA\nSend QUIT to Host"
      n906 = case shown="True" w2574 {
        tunnel: w2573 -> [_ w2584]
        tunnel: w2575 -> [w2581 w2583]
        tunnel: [w2581 w2582] -> w2572
        frame False {
        }
        frame True {
          n907 = xnode "Read/Write Control"("FPGA VI Reference In"=w2584, "error in"=w2583, "FPGA_Stop"=TRUE) -> ("error out"=w2582:errorcluster)  [unwired: 1 out]
        }
      }
      n908 = case shown="True" w2568 {
        tunnel: w2567 -> [_ w2580]
        tunnel: w2566 -> [_ w2579]
        frame False {
        }
        frame True {
          w2576 = "<S,Q><S,Q><S,Q><S,Q>" ("input_packet")
          n909 = call "BRig_RT_comm_tcp_write_RTwrite.vi"("input_error"=w2579, "input_packet"=w2576, "input_hTCP"=w2580) -> ("output_error"=w2578:errorcluster, "output_hTCP"=w2577:refnum<k5>)  [unwired: 5 in, 2 out]
          n910 = call "BRig_RT_comm_tcp_write_RTwrite.vi"("input_error"=w2578, "input_packet"=w2576, "input_hTCP"=w2577) -> ()  [unwired: 5 in, 4 out]
        }
      }
    }
    frame #1 {
      # "Disconnect FPGA\nDisconnect comm webdav"
      n911 = case shown="True" w2595 {
        tunnel: w2593 -> [w2600 w2603]
        tunnel: w2594 -> [_ w2602]
        tunnel: [w2600 w2601] -> w2592
        frame False {
        }
        frame True {
          n912 = xnode "Close FPGA VI Reference"("FPGA VI Reference In"=w2602, "error in"=w2603) -> ("error out"=w2604:errorcluster)
          n913 = call <vilib>:"Reset myRIO.vi"("error in (no error)"=w2604) -> ("error out"=w2601:errorcluster)  [unwired: 10 in]
        }
      }
      n914 = case shown="True" w2588 {
        tunnel: w2587 -> [_ w2597]
        tunnel: w2586 -> [_ w2596]
        frame False {
        }
        frame True {
          n915 = TCP Close Connection(connection ID=w2597, error in (no error)=w2596) -> ()  [unwired: 1 in, 2 out]
        }
      }
      n916 = case shown="True" w2591 {
        tunnel: w2590 -> [_ w2599]
        tunnel: w2589 -> [_ w2598]
        frame False {
        }
        frame True {
          n917 = call <vilib>:"Close Session.vi"("session handle"=w2599, "error in (no error)"=w2598) -> ()  [unwired: 13 in, 1 out]
        }
      }
    }
  }
  n918 = Flush Stream(8:w1, 11:w2) -> (0:w3:errorcluster, 3:w4:refnum<k21>)  [unwired: 2 in, 1 out]
  n919 = Flush Stream(8:w13, 11:w14) -> (0:w15:errorcluster, 3:w16:refnum<k21>)  [unwired: 2 in, 1 out]
  n920 = Destroy Stream Endpoint(8:w3, 11:w4) -> ()  [unwired: 1 out]
  n921 = Destroy Stream Endpoint(8:w15, 11:w16) -> ()  [unwired: 1 out]
